vi "SpectrometerSpinCoater_v11.vi"() -> ()   [LabVIEW 2020]
uses:
  <instrlib>/Classes/CCD/Abstract_CCD/Abstract_CCD.lvclass
  <instrlib>/Classes/SpinCoater/SpinCoater.lvclass
  TypDef/DeviceQueue_TypeDef.ctl
  TypDef/DeviceQueue_Action.ctl
  TypDef/TabControl.ctl
  TypDef/DataQueue_TypeDef.ctl
  TypDef/DataQueue_Action.ctl
  <vilib>/Utility/error.llb/DialogType.ctl
  <instrlib>/Classes/CCD/Avantes/Avantes.lvclass
  C:/Program Files/National Instruments/LabVIEW 2020/instr.lib/Classes/CCD/Abstract_CCD/Abstract_CCD.lvclass
  <vilib>/Analysis/baseanly.llb/A x Vector.vi
  <vilib>/Analysis/NI_AALBase.lvlib
panel:
  out "UpperWLLimit":i32=713
  out "LowerWLLimit":i32=149
  out "Nr After Spin":u16
  out "Action":string="TimeOut"
  out "Time.spin":refnum<file>
  out "Meas.spin":refnum<file>
  out "Arduino":bool
  out "NKT":bool
  out "Spectromter":bool
  in  "Abort Button":bool
  in  "Stop Button":bool=TRUE
  in  "Tab Control":T1(tab)
  in  "Trim\nSpec":bool=TRUE
  in  "Wl \nUp":dbl[unit]=7.102291259765626e-07
  in  "Wl \nLow":dbl[unit]=3.7998095703125003e-07
  in  "Frames for Ref/Dark":dbl=10000.0
  in  "Shutter Toggle":bool
  in  "Spin at end":bool
  in  "Duration after":dbl[unit]
  in  "periodic time":dbl[unit]=2.0
  in  "Program Spin Coater":T2(array[cluster])=[{"Speed (rpm)"=1500.0, "Time (s)"=5.0, "Acc (rpm/s)"=0.0}]
  in  "Spectra Count":u16
  in  "Measure_MeasureSpectrum":bool
  out "Overall Time":dbl=13.0
  in  "Seconds after Spin":dbl[unit]=3.0
  in  "Seconds to Spin":dbl[unit]=5.0
  in  "Calculate Frames":bool=TRUE
  in  "Frames":i32=34211
  in  "StartMeasurement_Button":bool
  in  "Measure_Preview":bool
  out "Measure_Graph":T3(graph) caption="XY Graph"
  in  "Measure_FramesSpectrometer":dbl=200.0 caption="Frames for Spectrometer"
  in  "StartSpin_Button":bool
  in  "Record RefSpec":bool
  in  "Measure:\nRecord_Darkspec":bool
  in  "Measure_Comments":string="Just for testing" caption="Comments"
  in  "Measure_FileName":string="TestCutting_WithLight" caption="File Name"
  in  "Measure_SavePath":path=path "C:/Users/Cerberus/Desktop/Test/V11Test" caption="Save Path"
  out "Measure_FrameRate":dbl[unit]=2631.5791015625 caption="Frame Rate"
  in  "Measure_IntegrationTime":dbl[unit]=3e-05 caption="Integration Time"
  out "SS_StepsLeft":dbl
  out "SS_TimePrediction":dbl[unit]=-6.0
  out "Horizontal Progress Bar":u8(slide) scale=0.0..100.0
  in  "SpectralStability:\nRecord_Darkspec":bool
  in  "SpectralStability_Record":bool
  in  "SpectralStability_\nMeasurementNumber":u32 caption="Measurement Number"
  in  "SpectralStability_Duration":dbl[unit] caption="Duration"
  in  "Duration/Times":bool
  in  "SpectralStability_\nPeriodicTime":dbl[unit] caption="Periodic Time"
  in  "SpectralStability_MeasureSpectrum":bool
  in  "SpectralStability_Preview":bool
  out "SpectralStability_Graph":T3(graph) caption="XY Graph"
  in  "SpectralStability_FramesSpectrometer":dbl=200.0 caption="Frames for Spectrometer"
  in  "SpectralStability_Comments":string="Just for testing" caption="Comments"
  in  "SpectralStability_FileName":string="TestingAfter" caption="File Name"
  in  "SpectralStability_SavePath":path=path "C:/Users/Timo/Desktop/Test/180824" caption="Save Path"
  out "SpectralStability_FrameRate":dbl[unit]=2631.5791015625 caption="Frame Rate"
  in  "SpectralStability_IntegrationTime":dbl[unit]=3e-05 caption="Integration Time"
  in  "Shutter Close":bool
  in  "Shutter Open":bool
  in  "SHUTTER DEBUG":bool
  in  "Shutter Position":u16=1000
  in  "Dividider Get Spectra":u32=1 min=1
  in  "Automatically \nadjust count":bool=TRUE
  in  "Reset Count\nafter Spin Coating":bool=TRUE
  in  "ESC_Speed":dbl
  in  "ESC_Milliseconds":dbl
  in  "ESC DEBUG":bool
  in  "Port Arduino":refnum<visa-resource-name>="COM7"
  out "Error Arduino":bool caption="Error"
  in  "Init_Arduino":bool caption="Init"
  out "Caption_Settings_Arduino":string="Arduino"
  out "Caption_Settings_NKT":string="NKT Laser"
  out "Error_Spectromter":bool caption="Error"
  in  "Init_Spectrometer":bool caption="Init"
  out "Caption_Settings_Spectrometer":string="Spectromter"
  # "Speed (rpm)   Time (s)        Acceleration \n                                               (rpm/s)"
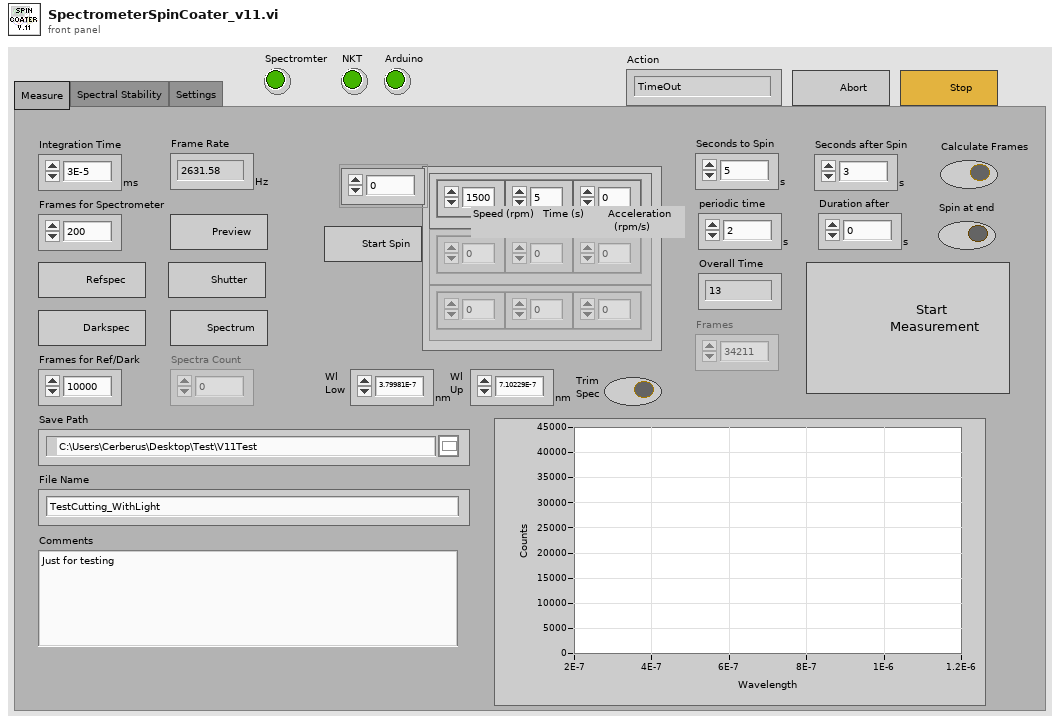
[diagram p1: front panel]
types:
  T1 = enum32{"Measure", "Spectral Stability", "Settings"}
  T2 = cluster{"Speed (rpm)":dbl, "Time (s)":dbl, "Acc (rpm/s)":dbl}[]
  T3 = cluster{"Wavlength":dbl[unit][], "Image":dbl[]}[]
  T4 = cluster{"Dark":cluster{"Image":dbl[][][], "Frame Size":cluster{"F":i32, "Y":i32, "X":i32}}[], "Ref":cluster{"Image":dbl[][][], "Frame Size":cluster{"F":i32, "Y":i32, "X":i32}}[], "Wavlength":dbl[unit][], "Wavlength Trim":dbl[unit][], "spec":dbl[][]}
  T5 = cluster{"Abstract_CCD.lvclass":refnum<class "Abstract_CCD.lvclass">, "SpinCoater.lvclass":refnum<class "SpinCoater.lvclass">}
  T6 = typedef "DataQueue_TypeDef.ctl" = cluster{"QueueAction":T7, "Data":cluster{"Image":dbl[][][], "Frame Size":cluster{"F":i32, "Y":i32, "X":i32}}[], "Data_Raw":cluster{"Image":dbl[][][], "Frame Size":cluster{"F":i32, "Y":i32, "X":i32}}[], "Data_Dark":cluster{"Image":dbl[][][], "Frame Size":cluster{"F":i32, "Y":i32, "X":i32}}[], "Data_Ref":cluster{"Image":dbl[][][], "Frame Size":cluster{"F":i32, "Y":i32, "X":i32}}[], "Device Information":string[], "Numeric Control":dbl, "Boolean":bool, "Wavelength":dbl[unit][], "Time":dbl[], "Time Stamp":timestamp, "Numeric Control 2":dbl, "TabControl":T8}
  T7 = typedef "DataQueue_Action.ctl" = enum16{"TimeOut", "Close_Program", "Abort", "Stop_Measurement", "Measure_InSituSpinCoating", "Measure_Spectrum", "Measure_SpectrumAdvanced", "Measure_SpectralStability", "Save_InSitu", "Save_SpectralStability", "Set_Ref", "Set_Dark", "Set_Wavelength", "Spectrometer_Measure", "Spectrometer_Preview", "Transfer_Settings", "Change_TrimSettings"}
  T8 = typedef "TabControl.ctl" = enum16{"Measure", "Spectral Stability", "Settings"}
  T9 = typedef "DeviceQueue_TypeDef.ctl" = cluster{"QueueAction":T10, "Numeric 1":dbl, "Numeric 2":dbl, "Boolean 1":bool, "Boolean 2":bool, "Spin Program":dbl[][], "Spin Prg v07":cluster{"Speed (rpm)":dbl, "Time (s)":dbl, "Acc (rpm/s)":dbl}[], "Time Stamp":timestamp, "TabControl":T8}
  T10 = typedef "DeviceQueue_Action.ctl" = enum16{"TimeOut", "Wait", "Close_Program", "Abort", "Spectrometer_Init", "Spectrometer_Close", "Spectrometer_DeviceInformation", "Spectrometer_Measure", "Spectrometer_MeasureAdvanced", "Spectrometer_Preview", "Spectrometer_Abort", "Spectrometer_StartMeasurement", "Spectrometer_GetData", "Spectrometer_StopMeasurement", "Spectrometer_SetIntegrationTime", "Spectrometer_SetFrames", "Spectrometer_SetDarkspec", "Spectrometer_SetReference", "Spectrometer_SetTriggerMode", "Laser_Init", "Laser_Close", "Arduino_Init", "Arduino_Close", "Arduino_LoadProgram", "Arduino_StartProgram", "Arduino_SetSpeed", "Arduino_SetMillis", "Arduino_StopSpin", "Arduino_Shutter_SetPosition", "Arduino_Shutter_Close", "Arduino_Shutter_Open", "Measure_InSitu", "Measure_Spectrum", "Measure_InSituAdvanced", "Measure_SpectralStability", "Measure_Stop"}
  T11 = cluster{"Image":dbl[][][], "Frame Size":cluster{"F":i32, "Y":i32, "X":i32}}[]
  T12 = typedef "DialogType.ctl" = u16
  T13 = enum16{"open", "replace", "create", "open or create", "replace or create", "replace or create with confirmation"}
  T14 = cluster{"Image":dbl[][][], "Frame Size":cluster{"F":i32, "Y":i32, "X":i32}}
  T15 = cluster{"Wavlength":dbl[unit][], "A x Vector":dbl[]}
  T16 = cluster{"Wavlength":dbl[unit][], "A x Vector":dbl[]}[]
  T17 = cluster{u16[][][], u16[][][], dbl[], "Numeric Control":dbl, "Numeric Control 2":dbl}
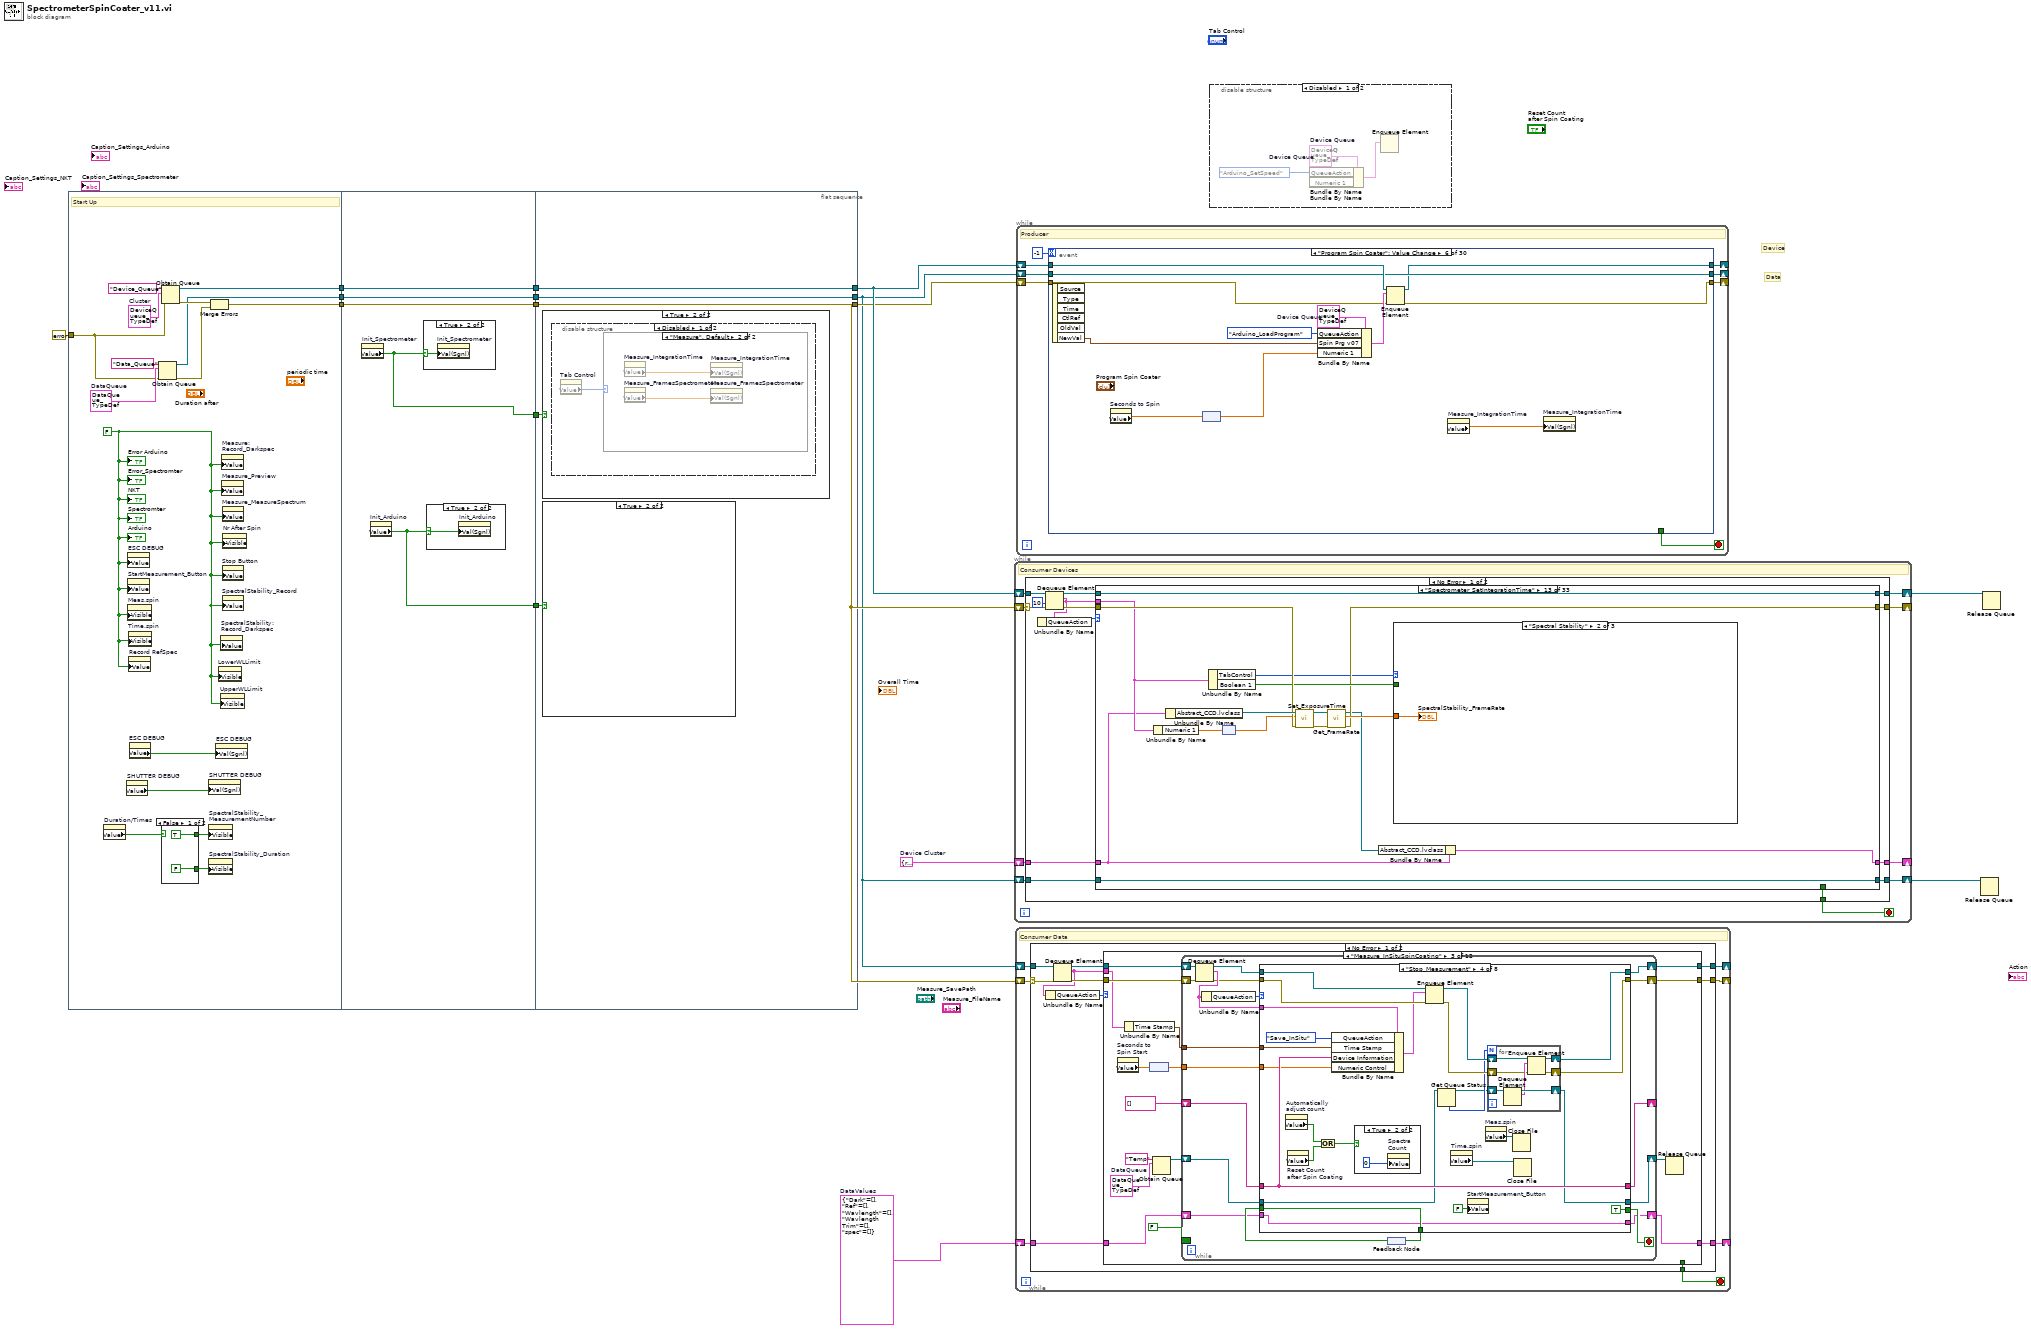
[diagram p0: block diagram]
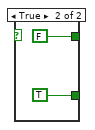
[diagram p3: hidden frame]
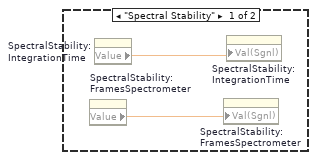
[diagram p8: hidden frame]
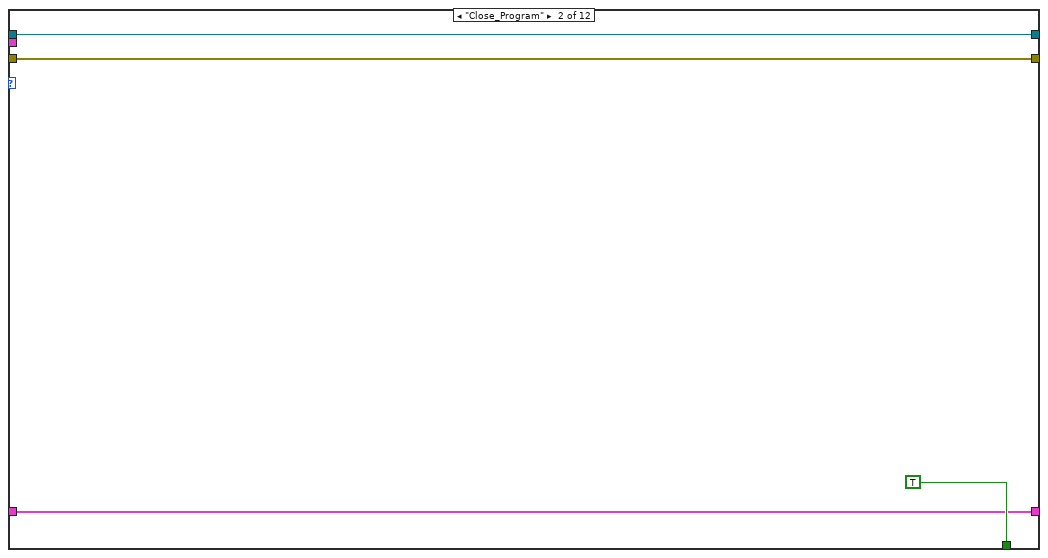
[diagram p11: hidden frame]
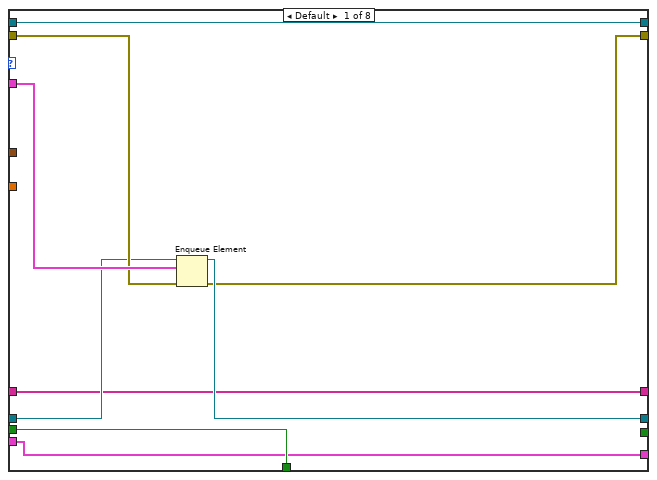
[diagram p12: hidden frame]
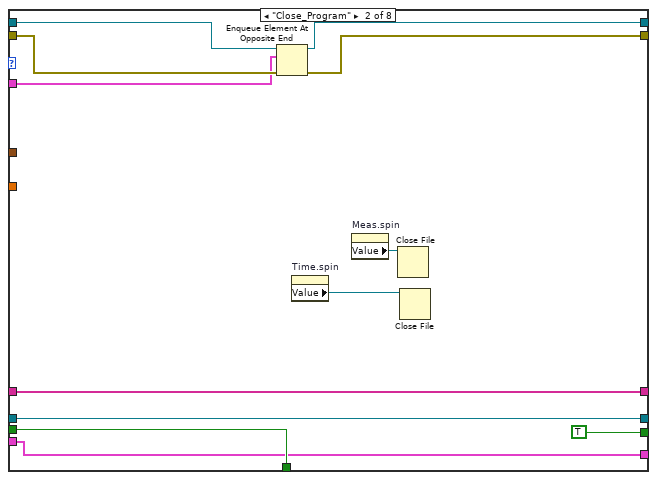
[diagram p13: hidden frame]
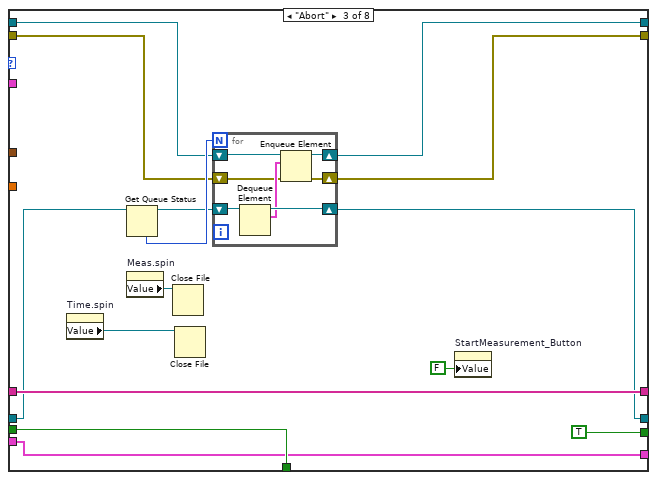
[diagram p14: hidden frame]
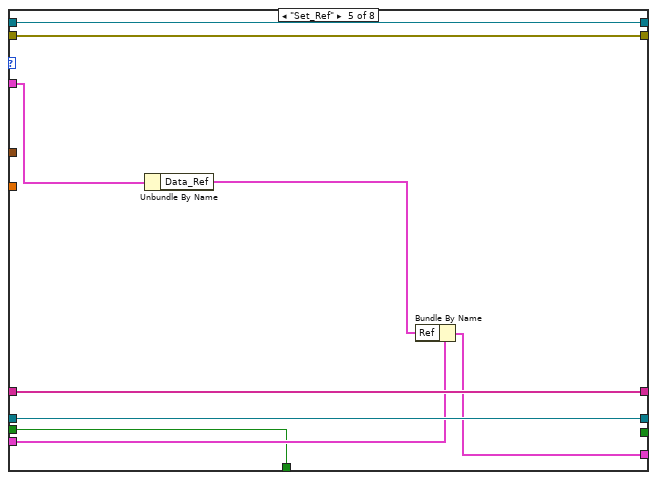
[diagram p16: hidden frame]
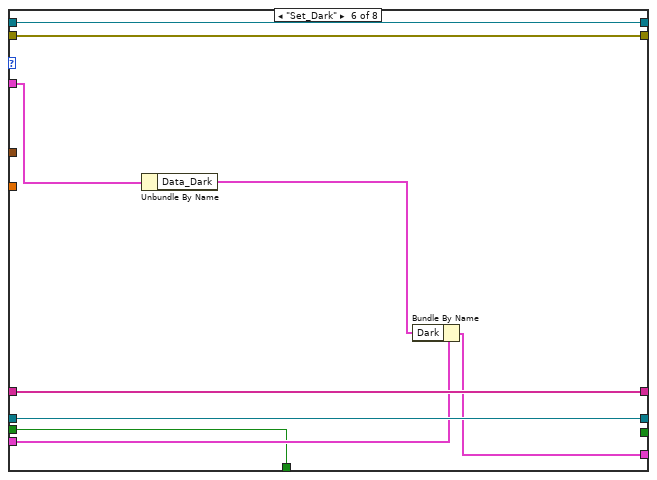
[diagram p17: hidden frame]
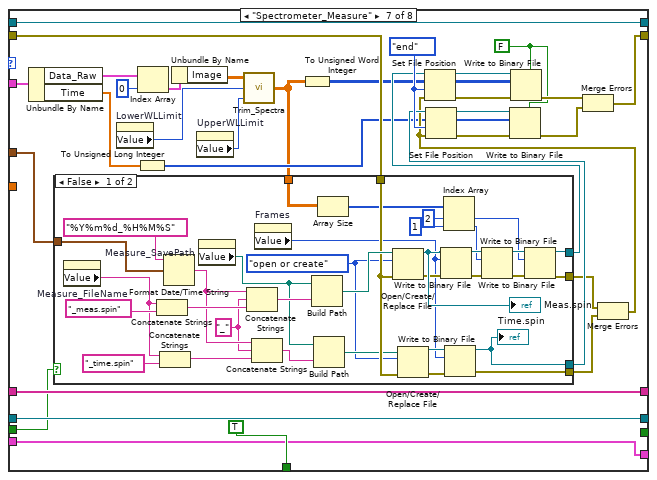
[diagram p18: hidden frame]
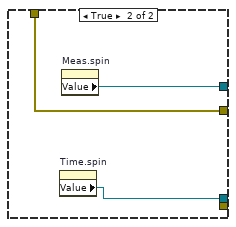
[diagram p19: hidden frame]
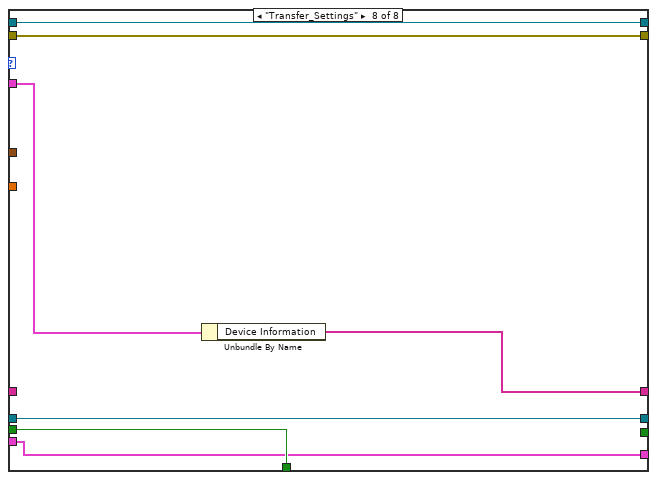
[diagram p20: hidden frame]
diagram:
  w6 = T4 {"Dark"=[], "Ref"=[], "Wavlength"=[], "Wavlength Trim"=[], "spec"=[]}  # DataValues
  w11 = T5 {"Abstract_CCD.lvclass"=refnum, "SpinCoater.lvclass"=refnum}  # Device Cluster
  # "Data"
  # "Device"
  n1 = flat-sequence {
    tunnel: errorcluster {"status"=FALSE, "code"=0, "source"=""} ("error constant") -> [w27]
    tunnel: [w30] -> w15
    tunnel: [w24] -> w14
    tunnel: [w23] -> w13
    tunnel: w15 -> [w41]
    tunnel: w14 -> [w40]
    tunnel: w13 -> [w39]
    tunnel: [w41] -> w5
    tunnel: [w40] -> w4
    tunnel: [w39] -> w3
    tunnel: [w38] -> w2
    tunnel: [w37] -> w1
    tunnel: [w46] -> w8
    tunnel: [w47] -> w7
    tunnel: [w48] -> w12
    tunnel: w5 -> [w48]
    tunnel: w4 -> [w47]
    tunnel: w3 -> [w46]
    tunnel: w2 -> [w45]
    tunnel: w1 -> [w44]
    frame #0 {
      w28 = T6 {"QueueAction"=enum."TimeOut", "Data"=[], "Data_Raw"=[], "Data_Dark"=[], "Data_Ref"=[], "Device Information"=[], "Numeric Control"=0.0, "Boolean"=FALSE, "Wavelength"=[], "Time"=[], "Time Stamp"=timestamp(0 s since 1904-01-01), "Numeric Control 2"=0.0, "TabControl"=enum."Measure"}  # DataQueue
      w31 = T9 {"QueueAction"=enum."TimeOut", "Numeric 1"=0.0, "Numeric 2"=0.0, "Boolean 1"=FALSE, "Boolean 2"=FALSE, "Spin Program"=[], "Spin Prg v07"=[], "Time Stamp"=timestamp(0 s since 1904-01-01), "TabControl"=enum."Measure"}  # Cluster
      w17 = FALSE ("Error Arduino")
      # "Start Up"
      n2 = property on="Duration/Times" class="Bool (strict)"() -> ("Value"=w19:bool)  [unwired: 2 in, 2 out]
      n3 = property on="SHUTTER DEBUG" class="Bool (strict)"() -> ("Value"=w18:bool)  [unwired: 2 in, 2 out]
      n4 = property on="ESC DEBUG" class="Bool (strict)"("Value"=w17) -> ()  [unwired: 2 in, 2 out]
      n5 = property on="StartMeasurement_Button" class="Bool (strict)"("Value"=w17) -> ()  [unwired: 2 in, 2 out]
      n6 = property on="Meas.spin" class="Ref (strict)"("Visible"=w17) -> ()  [unwired: 2 in, 2 out]
      n7 = property on="Time.spin" class="Ref (strict)"("Visible"=w17) -> ()  [unwired: 2 in, 2 out]
      n8 = property on="Record RefSpec" class="Bool (strict)"("Value"=w17) -> ()  [unwired: 2 in, 2 out]
      n9 = property on="ESC DEBUG" class="Bool (strict)"() -> ("Value"=w22:bool)  [unwired: 2 in, 2 out]
      n10 = Obtain Queue(name (unnamed)="Data_Queue", element data type=w28, error in (no error)=w27) -> (queue out=w24:refnum<queue>, error out=w25:errorcluster)  [unwired: 2 in, 1 out]
      n11 = case shown="False" w19 {
        tunnel: [FALSE TRUE] -> w21
        tunnel: [TRUE FALSE] -> w20
        frame False {
        }
        frame True {
        }
      }
      n12 = Obtain Queue(name (unnamed)="Device_Queue", element data type=w31, error in (no error)=w27) -> (queue out=w30:refnum<queue>, error out=w26:errorcluster)  [unwired: 2 in, 1 out]
      n13 = property on="SHUTTER DEBUG" class="Bool (strict)"("Val(Sgnl)"=w18) -> ()  [unwired: 2 in, 2 out]
      n14 = property on="SpectralStability_\nMeasurementNumber" class="DigNum (strict)"("Visible"=w20) -> ()  [unwired: 2 in, 2 out]
      n15 = property on="SpectralStability_Duration" class="DigNum (strict)"("Visible"=w21) -> ()  [unwired: 2 in, 2 out]
      n16 = Merge Errors(w26, w25) -> (w23:errorcluster)
      n17 = property on="ESC DEBUG" class="Bool (strict)"("Val(Sgnl)"=w22) -> ()  [unwired: 2 in, 2 out]
      n18 = property on="LowerWLLimit" class="DigNum (strict)"("Visible"=w17) -> ()  [unwired: 2 in, 2 out]
      n19 = property on="UpperWLLimit" class="DigNum (strict)"("Visible"=w17) -> ()  [unwired: 2 in, 2 out]
      n20 = property on="SpectralStability:\nRecord_Darkspec" class="Bool (strict)"("Value"=w17) -> ()  [unwired: 2 in, 2 out]
      n21 = property on="Measure:\nRecord_Darkspec" class="Bool (strict)"("Value"=w17) -> ()  [unwired: 2 in, 2 out]
      n22 = property on="Measure_Preview" class="Bool (strict)"("Value"=w17) -> ()  [unwired: 2 in, 2 out]
      n23 = property on="Measure_MeasureSpectrum" class="Bool (strict)"("Value"=w17) -> ()  [unwired: 2 in, 2 out]
      n24 = property on="Stop Button" class="Bool (strict)"("Value"=w17) -> ()  [unwired: 2 in, 2 out]
      n25 = property on="SpectralStability_Record" class="Bool (strict)"("Value"=w17) -> ()  [unwired: 2 in, 2 out]
      n26 = property on="Nr After Spin" class="DigNum (strict)"("Visible"=w17) -> ()  [unwired: 2 in, 2 out]
      "Error_Spectromter" <- w17
      "Error Arduino" <- w17
      "Spectromter" <- w17
      "NKT" <- w17
      "Arduino" <- w17
    }
    frame #1 {
      n27 = property on="Init_Spectrometer" class="Bool (strict)"() -> ("Value"=w38:bool)  [unwired: 2 in, 2 out]
      n28 = property on="Init_Arduino" class="Bool (strict)"() -> ("Value"=w37:bool)  [unwired: 2 in, 2 out]
      n29 = case shown="True" w38 {
        selector: w38 -> [_ w43]
        frame False {
        }
        frame True {
          n30 = property on="Init_Spectrometer" class="Bool (strict)"("Val(Sgnl)"=w43) -> ()  [unwired: 2 in, 2 out]
        }
      }
      n31 = case shown="True" w37 {
        selector: w37 -> [_ w42]
        frame False {
        }
        frame True {
          n32 = property on="Init_Arduino" class="Bool (strict)"("Val(Sgnl)"=w42) -> ()  [unwired: 2 in, 2 out]
        }
      }
    }
    frame #2 {
      n33 = case shown="True" w45 {
        frame False {
        }
        frame True {
          n34 = disable-structure shown="Disabled" {
            frame Disabled {
              n35 = property on="Tab Control" class="TabCtl (strict)"() -> ("Value"=w49:T1)  [unwired: 2 in, 2 out]
              n36 = case shown="\"Measure\", Default" w49 {
                frame "Spectral Stability" {
                  n37 = property on="SpectralStability:\nFramesSpectrometer" class="DigNum (strict)"() -> ("Value"=w50:dbl)  [unwired: 2 in, 2 out]
                  n38 = property on="SpectralStability:\nIntegrationTime" class="DigNum (strict)"() -> ("Value"=w51:dbl[unit])  [unwired: 2 in, 2 out]
                  n39 = property on="SpectralStability:\nFramesSpectrometer" class="DigNum (strict)"("Val(Sgnl)"=w50) -> ()  [unwired: 2 in, 2 out]
                  n40 = property on="SpectralStability:\nIntegrationTime" class="DigNum (strict)"("Val(Sgnl)"=w51) -> ()  [unwired: 2 in, 2 out]
                }
                frame "Measure", Default {
                  n41 = property on="Measure_IntegrationTime" class="DigNum (strict)"() -> ("Value"=w52:dbl[unit])  [unwired: 2 in, 2 out]
                  n42 = property on="Measure_FramesSpectrometer" class="DigNum (strict)"() -> ("Value"=w53:dbl)  [unwired: 2 in, 2 out]
                  n43 = property on="Measure_IntegrationTime" class="DigNum (strict)"("Val(Sgnl)"=w52) -> ()  [unwired: 2 in, 2 out]
                  n44 = property on="Measure_FramesSpectrometer" class="DigNum (strict)"("Val(Sgnl)"=w53) -> ()  [unwired: 2 in, 2 out]
                }
              }
            }
            frame Enabled {
            }
          }
        }
      }
      n45 = case shown="True" w44 {
        frame False {
        }
        frame True {
        }
      }
    }
  }
  n46 = while {
    shift-right: [w58] -> _
    shift-left: w8 -> [w62]
    shift-right: [w59] -> w10
    shift-left: w12 -> [w61]
    shift-right: [w56] -> w9
    shift-left: w7 -> [w57]
    shift-right: [w54] -> _
    shift-left: w11 -> [w55]
    stop <- w60 stop-if-true
    # "Consumer Devices"
    n47 = case shown="No Error" w62 {
      selector: w62 -> [w75 w792]
      tunnel: w61 -> [w76 w793]
      tunnel: [w72 _] -> w60
      tunnel: [w71 w793] -> w59
      tunnel: [w69 w789] -> w58
      tunnel: w57 -> [w67 w787]
      tunnel: [w68 w787] -> w56
      tunnel: w55 -> [w66 w788]
      tunnel: [w65 w788] -> w54
      frame No Error {
        n48 = Dequeue Element(queue=w76, timeout in ms (-1)=10, error in (no error)=w75) -> (queue out=w74:refnum<queue>, element=w64:T9, error out=w70:errorcluster)  [unwired: 1 out]
        n49 = Unbundle By Name(w64) -> ("QueueAction"=w73:T10)
        n50 = case shown="\"Spectrometer_SetIntegrationTime\"" w73 {
          tunnel: w74 -> [w81 w102 w143 w161 w172 w227 w246 w271 w282 w305 w312 w331 w333 w364 w383 w398 w408 w420 w432 w453 w475 w480 w487 w499 w505 w517 w524 w531 w540 w586 w680 w748 w758]
          tunnel: [_ _ w145 _ _ _ _ _ _ _ _ _ _ _ _ _ _ _ _ _ _ _ _ _ _ _ _ _ _ _ _ _ _] -> w72
          tunnel: [w81 w102 w128 w147 w168 w227 w246 w271 w283 w305 w312 w331 w333 w364 w383 w398 w408 w420 w431 w453 w475 w480 w487 w499 w505 w517 w524 w531 w540 w548 w596 w739 w761] -> w71
          tunnel: w70 -> [w80 w101 w127 w160 w183 w228 w245 w270 w278 w308 w316 w328 w343 w362 w373 w389 w405 w416 w427 w456 w469 w477 w485 w494 w502 w508 w520 w527 w533 w542 w641 w747 w757]
          tunnel: [w80 w101 w126 w148 w171 w222 w244 w269 w276 w306 w313 w318 w337 w361 w368 w385 w403 w410 w430 w455 w466 w476 w483 w493 w501 w507 w519 w526 w532 w549 w595 w738 w762] -> w69
          tunnel: [w78 w99 w125 w165 w169 w224 w237 w251 w287 w304 w311 w322 w345 w365 w377 w392 w399 w412 w434 w454 w474 w482 w491 w497 w506 w516 w523 w530 w535 w557 w653 w746 w778] -> w68
          tunnel: w67 -> [w78 w99 w125 w165 w170 w224 w236 w260 w288 w304 w311 w323 w345 w365 w380 w395 w399 w414 w434 w454 w474 w482 w491 w497 w506 w516 w523 w530 w536 w557 w653 w746 w778]
          tunnel: w66 -> [w79 w100 w124 w164 w180 w226 w243 w268 w281 w303 w315 w324 w336 w358 w376 w391 w402 w409 w429 w449 w468 w481 w490 w496 w504 w515 w522 w529 w534 w589 w683 w745 w777]
          tunnel: [w79 w100 w124 w164 w174 w225 w243 w268 w280 w301 w310 w324 w334 w359 w375 w390 w400 w409 w433 w447 w465 w481 w490 w496 w504 w515 w522 w529 w534 w589 w683 w745 w777] -> w65
          tunnel: w64 -> [_ w95 _ _ w167 _ w235 w262 w274 _ _ w330 w340 w366 _ _ w406 _ _ _ w473 _ w489 w498 _ w513 _ _ _ _ w623 w736 w752]
          frame "TimeOut", Default {
            n51 = property on="Action" class="Str"("Value"="TimeOut" ("Action")) -> ()  [unwired: 2 in, 2 out]
          }
          frame "Wait" {
            n52 = flat-sequence {
              tunnel: [w113] -> w96
              tunnel: w95 -> [w113]
              tunnel: [w112] -> w93
              frame #0 {
                n53 = Tick Count (ms)() -> (millisecond timer value=w112:u32)
              }
            }
            n54 = Unbundle By Name(w96) -> ("Numeric 1"=w87:dbl)
            n55 = property on="SS:PeriodicTime" class="DigNum (strict)"() -> ("Value"=w89:dbl[unit])  [unwired: 2 in, 2 out]
            n56 = Multiply(x=w87, y=1000.0) -> (x*y=w91:dbl)
            n57 = node(w87) -> (w88:dbl[unit])
            n58 = property on="SS_StepsLeft" class="DigNum (strict)"() -> ("Value"=w86:dbl)  [unwired: 2 in, 2 out]
            n59 = Round Toward -Infinity(1:w87) -> (0:w90:dbl)
            n60 = Subtract(x=w89, y=w88) -> (x-y=w83:dbl[unit])
            n61 = Decrement(x=w86) -> (x-1=w85:dbl)
            n62 = Multiply(x=w85, y=w89) -> (x*y=w84:dbl[unit])
            n63 = Add(x=w84, y=w83) -> (x+y=w82:dbl[unit])
            n64 = for {
              N: w90 -> [_]
              tunnel: 1000.0 ("y") -> [w114]
              tunnel: [w122] -> w94
              tunnel: w82 -> [w119]
              i -> [w117]
              stop <- w122 stop-if-true
              n65 = Increment(x=w117) -> (x+1=w115:i32)
              n66 = Multiply(x=w114, y=w115) -> (x*y=w116:dbl)
              n67 = node(w116) -> (w118:dbl[unit])
              n68 = property on="Stop Button" class="Bool (strict)"() -> ("Value"=w122:bool)  [unwired: 2 in, 2 out]
              n69 = Wait (ms)(milliseconds to wait=w114) -> (millisecond timer value=w120:u32)
              n70 = Subtract(x=w119, y=w118) -> (x-y=w121:dbl[unit])
              n71 = flat-sequence {
                tunnel: w121 -> [w123]
                tunnel: w120 -> [_]
                frame #0 {
                  n72 = property on="SS_TimePrediction" class="DigNum (strict)"("Value"=w123) -> ()  [unwired: 2 in, 2 out]
                }
              }
            }
            n73 = property on="Action" class="Str"("Value"="Wait" ("Action")) -> ()  [unwired: 2 in, 2 out]
            n74 = case shown="False" w94 {
              tunnel: w93 -> [w108 _]
              tunnel: w91 -> [w103 _]
              frame False {
                n75 = flat-sequence {
                  tunnel: [w111] -> w109
                  frame #0 {
                    n76 = Tick Count (ms)() -> (millisecond timer value=w111:u32)
                  }
                }
                n77 = Subtract(x=w109, y=w108) -> (x-y=w107:u32)
                n78 = To Double Precision Float(number=w107) -> (double precision float=w104:dbl)
                n79 = Subtract(x=w103, y=w104) -> (x-y=w105:dbl)
                n80 = Greater Than 0?(x=w105) -> (x > 0?=w106:bool)
                n81 = case shown="True" w106 {
                  tunnel: w105 -> [_ w110]
                  frame False {
                  }
                  frame True {
                    n82 = Wait (ms)(milliseconds to wait=w110) -> ()  [unwired: 1 out]
                  }
                }
              }
              frame True {
                # "If Aborted, do nothing"
              }
            }
          }
          frame "Close_Program" {
            w144 = T9 {"QueueAction"=enum."TimeOut", "Numeric 1"=0.0, "Numeric 2"=0.0, "Boolean 1"=FALSE, "Boolean 2"=FALSE, "Spin Program"=[], "Spin Prg v07"=[], "Time Stamp"=timestamp(0 s since 1904-01-01), "TabControl"=enum."Measure"}  # Device Queue
            n83 = Bundle By Name(cluster=w144, "QueueAction"=DeviceQueue_Action."Spectrometer_Close") -> (w139:T9)
            n84 = Bundle By Name(cluster=w139, "QueueAction"=DeviceQueue_Action."Laser_Close") -> (w137:T9)
            n85 = Bundle By Name(cluster=w137, "QueueAction"=DeviceQueue_Action."Arduino_Close") -> (w131:T9)
            n86 = Enqueue Element(queue=w143, element=w139, error in (no error)=w127) -> (queue out=w141:refnum<queue>, error out=w136:errorcluster)  [unwired: 1 in, 1 out]
            n87 = Bundle By Name(cluster=w131, "QueueAction"=DeviceQueue_Action."Close_Program") -> (w129:T9)
            n88 = Enqueue Element(queue=w141, element=w137, error in (no error)=w136) -> (queue out=w135:refnum<queue>, error out=w134:errorcluster)  [unwired: 1 in, 1 out]
            n89 = Enqueue Element(queue=w135, element=w131, error in (no error)=w134) -> (queue out=w133:refnum<queue>, error out=w132:errorcluster)  [unwired: 1 in, 1 out]
            n90 = Enqueue Element(queue=w133, element=w129, error in (no error)=w132) -> (queue out=w128:refnum<queue>, error out=w126:errorcluster)  [unwired: 1 in, 1 out]
            n91 = First Call?() -> (First Call?: T/F=w146:bool)
            n92 = Not(x=w146) -> (.not. x?=w145:bool)
          }
          frame "Abort" {
            w163 = T9 {"QueueAction"=enum."TimeOut", "Numeric 1"=0.0, "Numeric 2"=0.0, "Boolean 1"=FALSE, "Boolean 2"=FALSE, "Spin Program"=[], "Spin Prg v07"=[], "Time Stamp"=timestamp(0 s since 1904-01-01), "TabControl"=enum."Measure"}  # Device Queue
            n93 = Flush Queue(queue=w161, error in (no error)=w160) -> (queue out=w159:refnum<queue>, error out=w158:errorcluster)  [unwired: 1 out]
            n94 = Bundle By Name(cluster=w163, "QueueAction"=DeviceQueue_Action."Spectrometer_StopMeasurement") -> (w155:T9)
            n95 = Bundle By Name(cluster=w155, "QueueAction"=DeviceQueue_Action."Arduino_StopSpin") -> (w151:T9)
            n96 = Enqueue Element(queue=w159, element=w155, error in (no error)=w158) -> (queue out=w157:refnum<queue>, error out=w156:errorcluster)  [unwired: 1 in, 1 out]
            n97 = Bundle By Name(cluster=w151, "QueueAction"=DeviceQueue_Action."Measure_Stop") -> (w150:T9)
            n98 = Enqueue Element(queue=w157, element=w151, error in (no error)=w156) -> (queue out=w153:refnum<queue>, error out=w152:errorcluster)  [unwired: 1 in, 1 out]
            n99 = Enqueue Element(queue=w153, element=w150, error in (no error)=w152) -> (queue out=w147:refnum<queue>, error out=w148:errorcluster)  [unwired: 1 in, 1 out]
          }
          frame "Spectrometer_Init" {
            n100 = call-dynamic "Init.vi"("error in (no error)"=w183, "Variant"=0, "Avantes in"=refnum<class "Avantes.lvclass"> refnum ("Avantes.lvclass")) -> ("error out"=w182:errorcluster, "Avantes out"=w181:refnum<class "Avantes.lvclass">)  [unwired: 7 in]
            n101 = call-dynamic "IsInit.vi"("error in (no error)"=w182, "Avantes in"=w181) -> ("error out"=w178:errorcluster, "Is Init?"=w177:bool, "Avantes out"=w179:refnum<class "Avantes.lvclass">)  [unwired: 7 in]
            n102 = Unbundle By Name(w167) -> ("TabControl"=w166:T8)
            n103 = property on="Spectromter" class="Bool (strict)"("Value"=w177) -> ()  [unwired: 2 in, 2 out]
            n104 = property on="Init_Spectrometer" class="Bool (strict)"("Value"=w177) -> ()  [unwired: 2 in, 2 out]
            n105 = call-dynamic "Set_ExposurePerFrame.vi"("error in (no error)"=w178, "Exposure per Frame"=1, "Avantes in"=w179) -> ("error out"=w173:errorcluster, "Avantes out"=w176:refnum<class "Avantes.lvclass">)  [unwired: 7 in]
            n106 = case shown="True" w177 {
              tunnel: w176 -> [_ w206]
              tunnel: w173 -> [w189 w204]
              tunnel: [refnum<class "Abstract_CCD.lvclass"> refnum ("Abstract_CCD.lvclass") w205] -> w175
              tunnel: w172 -> [w187 w216]
              tunnel: [w189 w209] -> w171
              tunnel: w170 -> [w188 w201]
              tunnel: [w188 w199] -> w169
              tunnel: [w187 w197] -> w168
              tunnel: w167 -> [_ w194]
              tunnel: w166 -> [_ w193]
              frame False {
              }
              frame True {
                w207 = T6 {"QueueAction"=enum."TimeOut", "Data"=[], "Data_Raw"=[], "Data_Dark"=[], "Data_Ref"=[], "Device Information"=[], "Numeric Control"=0.0, "Boolean"=FALSE, "Wavelength"=[], "Time"=[], "Time Stamp"=timestamp(0 s since 1904-01-01), "Numeric Control 2"=0.0, "TabControl"=enum."Measure"}  # DataQueue
                n107 = case shown="\"Spectral Stability\"" w193 {
                  tunnel: [w218 w220] -> w192
                  tunnel: [w217 w219] -> w191
                  frame "Measure", Default {
                    n108 = property on="Measure_IntegrationTime" class="DigNum (strict)"() -> ("Value"=w218:dbl[unit])  [unwired: 2 in, 2 out]
                    n109 = property on="Measure_FramesSpectrometer" class="DigNum (strict)"() -> ("Value"=w217:dbl)  [unwired: 2 in, 2 out]
                  }
                  frame "Spectral Stability" {
                    n110 = property on="SpectralStability_FramesSpectrometer" class="DigNum (strict)"() -> ("Value"=w219:dbl)  [unwired: 2 in, 2 out]
                    n111 = property on="SpectralStability_IntegrationTime" class="DigNum (strict)"() -> ("Value"=w220:dbl[unit])  [unwired: 2 in, 2 out]
                  }
                }
                n112 = call-dynamic "Get_WavelengthAxis.vi"("error in (no error)"=w204, "Avantes in"=w206) -> ("error out"=w203:errorcluster, "lambda"=w198:dbl[unit][], "Avantes out"=w205:refnum<class "Avantes.lvclass">)  [unwired: 7 in]
                n113 = Unbundle(w203) -> ("status"=w202:bool)  [unwired: 2 out]
                n114 = property on="Error_Spectromter" class="Bool (strict)"("Value"=w202) -> ()  [unwired: 2 in, 2 out]
                n115 = property on="Calculate Frames" class="Bool (strict)"() -> ("Value"=w195:bool)  [unwired: 2 in, 2 out]
                n116 = Bundle By Name(cluster=w207, "QueueAction"=DataQueue_Action."Set_Wavelength", "Wavelength"=w198) -> (w208:T6)
                n117 = node(w192) -> (w214:dbl)
                n118 = Bundle By Name(cluster=w194, "QueueAction"=DeviceQueue_Action."Spectrometer_SetIntegrationTime", "Numeric 1"=w214, "Boolean 1"=w195) -> (w212:T9)
                n119 = Enqueue Element(queue=w201, element=w208) -> (queue out=w199:refnum<queue>)  [unwired: 2 in, 2 out]
                n120 = Bundle By Name(cluster=w212, "QueueAction"=DeviceQueue_Action."Spectrometer_SetFrames", "Numeric 1"=w191) -> (w211:T9)
                n121 = Enqueue Element(queue=w216, element=w212, error in (no error)=w204) -> (queue out=w213:refnum<queue>, error out=w210:errorcluster)  [unwired: 1 in, 1 out]
                n122 = Enqueue Element(queue=w213, element=w211, error in (no error)=w210) -> (queue out=w197:refnum<queue>, error out=w209:errorcluster)  [unwired: 1 in, 1 out]
              }
            }
            n123 = Bundle By Name(cluster=w180, "Abstract_CCD.lvclass"=w175) -> (w174:T5)
          }
          frame "Spectrometer_Close" {
            n124 = property on="Spectromter" class="Bool (strict)"("Value"=FALSE ("Spectromter")) -> ()  [unwired: 2 in, 2 out]
            n125 = Unbundle By Name(w226) -> ("Abstract_CCD.lvclass"=w229:refnum<class "Abstract_CCD.lvclass">)
            n126 = flat-sequence {
              tunnel: [refnum<class "Abstract_CCD.lvclass"> refnum ("Abstract_CCD.lvclass")] -> w223
              tunnel: w222 -> [_]
              frame #0 {
              }
            }
            n127 = call-dynamic "Close.vi"("error in (no error)"=w228, "Abstract_CCD in"=w229) -> ("error out"=w222:errorcluster)  [unwired: 8 in, 1 out]
            n128 = Bundle By Name(cluster=w226, "Abstract_CCD.lvclass"=w223) -> (w225:T5)
          }
          frame "Spectrometer_Measure" {
            w248 = T6 {"QueueAction"=enum."TimeOut", "Data"=[], "Data_Raw"=[], "Data_Dark"=[], "Data_Ref"=[], "Device Information"=[], "Numeric Control"=0.0, "Boolean"=FALSE, "Wavelength"=[], "Time"=[], "Time Stamp"=timestamp(0 s since 1904-01-01), "Numeric Control 2"=0.0, "TabControl"=enum."Measure"}  # DataQueue
            n129 = Unbundle By Name(w243) -> ("Abstract_CCD.lvclass"=w247:refnum<class "Abstract_CCD.lvclass">)
            n130 = Unbundle By Name(w235) -> ("Time Stamp"=w232:timestamp, "TabControl"=w233:T8)
            n131 = Get Date/Time In Seconds() -> (seconds since 1Jan1904=w231:timestamp)
            n132 = Subtract(x=w231, y=w232) -> (x-y=w234:dbl)
            n133 = call-dynamic "Measure.vi"("error in (no error)"=w245, "Abstract_CCD in"=w247) -> ("error out"=w244:errorcluster, "Data Raw"=w240:T11, "Data"=w241:T11, "Darkspec"=w239:T11, "Time"=w238:dbl[])  [unwired: 3 in, 2 out]
            n134 = Bundle By Name(cluster=w248, "QueueAction"=DataQueue_Action."Spectrometer_Measure", "Data"=w241, "Data_Raw"=w240, "Data_Dark"=w239, "Time"=w238, "Time Stamp"=w232, "Numeric Control 2"=w234, "TabControl"=w233) -> (w249:T6)
            n135 = Enqueue Element(queue=w236, element=w249) -> (queue out=w237:refnum<queue>)  [unwired: 2 in, 2 out]
          }
          frame "Spectrometer_MeasureAdvanced" {
            w259 = T6 {"QueueAction"=enum."TimeOut", "Data"=[], "Data_Raw"=[], "Data_Dark"=[], "Data_Ref"=[], "Device Information"=[], "Numeric Control"=0.0, "Boolean"=FALSE, "Wavelength"=[], "Time"=[], "Time Stamp"=timestamp(0 s since 1904-01-01), "Numeric Control 2"=0.0, "TabControl"=enum."Measure"}  # DataQueue
            w273 = T6 {"QueueAction"=enum."TimeOut", "Data"=[], "Data_Raw"=[], "Data_Dark"=[], "Data_Ref"=[], "Device Information"=[], "Numeric Control"=0.0, "Boolean"=FALSE, "Wavelength"=[], "Time"=[], "Time Stamp"=timestamp(0 s since 1904-01-01), "Numeric Control 2"=0.0, "TabControl"=enum."Measure"}  # DataQueue
            n136 = Unbundle By Name(w268) -> ("Abstract_CCD.lvclass"=w272:refnum<class "Abstract_CCD.lvclass">)
            n137 = Unbundle By Name(w262) -> ("Time Stamp"=w261:timestamp)
            n138 = call-dynamic "Measure.vi"("error in (no error)"=w270, "Abstract_CCD in"=w272) -> ("error out"=w269:errorcluster, "Data Raw"=w265:T11, "Data"=w266:T11, "Darkspec"=w264:T11, "Time"=w263:dbl[])  [unwired: 3 in, 2 out]
            n139 = Bundle By Name(cluster=w259, "QueueAction"=DataQueue_Action."Measure_SpectrumAdvanced") -> (w257:T6)
            n140 = Bundle By Name(cluster=w273, "QueueAction"=DataQueue_Action."Spectrometer_Measure", "Data"=w266, "Data_Raw"=w265, "Data_Dark"=w264, "Time"=w263, "Time Stamp"=w261) -> (w254:T6)
            n141 = Enqueue Element(queue=w260, element=w257) -> (queue out=w256:refnum<queue>)  [unwired: 2 in, 2 out]
            n142 = Enqueue Element(queue=w256, element=w254) -> (queue out=w255:refnum<queue>)  [unwired: 2 in, 2 out]
            n143 = Bundle By Name(cluster=w254, "QueueAction"=DataQueue_Action."Stop_Measurement") -> (w252:T6)
            n144 = property on="Action" class="Str"("Value"="Measure Spectra A" ("Action")) -> ()  [unwired: 2 in, 2 out]
            n145 = Enqueue Element(queue=w255, element=w252) -> (queue out=w251:refnum<queue>)  [unwired: 2 in, 2 out]
          }
          frame "Spectrometer_Preview" {
            w289 = T6 {"QueueAction"=enum."TimeOut", "Data"=[], "Data_Raw"=[], "Data_Dark"=[], "Data_Ref"=[], "Device Information"=[], "Numeric Control"=0.0, "Boolean"=FALSE, "Wavelength"=[], "Time"=[], "Time Stamp"=timestamp(0 s since 1904-01-01), "Numeric Control 2"=0.0, "TabControl"=enum."Measure"}  # DataQueue
            n146 = Unbundle By Name(w281) -> ("Abstract_CCD.lvclass"=w279:refnum<class "Abstract_CCD.lvclass">)
            n147 = Unbundle By Name(w274) -> ("TabControl"=w275:T8)
            n148 = call-dynamic "Measure.vi"("error in (no error)"=w278, "Abstract_CCD in"=w279) -> ("error out"=w276:errorcluster, "Data Raw"=w286:T11, "Abstract_CCD out"=w277:refnum<class "Abstract_CCD.lvclass">)  [unwired: 3 in, 4 out]
            n149 = case shown="\"Measure\"" w275 {
              tunnel: [FALSE ("Value") w293 w294] -> w284
              tunnel: w276 -> [_ w292 _]
              frame Default {
              }
              frame "Measure" {
                n150 = property on="Measure_Preview" class="Bool (strict)"(error in=w292) -> ("Value"=w293:bool)  [unwired: 1 in, 2 out]
              }
              frame "Spectral Stability" {
                n151 = property on="SpectralStability_Preview" class="Bool (strict)"() -> ("Value"=w294:bool)  [unwired: 2 in, 2 out]
              }
            }
            n152 = case shown="True" w284 {
              tunnel: [w295 w298] -> w283
              tunnel: w282 -> [w295 w297]
              tunnel: w274 -> [_ w296]
              frame False {
              }
              frame True {
                n153 = Bundle By Name(cluster=w296, "QueueAction"=DeviceQueue_Action."Spectrometer_Preview") -> (w299:T9)
                n154 = Enqueue Element(queue=w297, element=w299) -> (queue out=w298:refnum<queue>)  [unwired: 2 in, 2 out]
              }
            }
            n155 = Bundle By Name(cluster=w289, "Data_Raw"=w286, "QueueAction"=DataQueue_Action."Spectrometer_Preview", "TabControl"=w275) -> (w290:T6)
            n156 = Enqueue Element(queue=w288, element=w290) -> (queue out=w287:refnum<queue>)  [unwired: 2 in, 2 out]
            n157 = Bundle By Name(cluster=w281, "Abstract_CCD.lvclass"=w277) -> (w280:T5)
          }
          frame "Spectrometer_StartMeasurement" {
            n158 = Unbundle By Name(w303) -> ("Abstract_CCD.lvclass"=w307:refnum<class "Abstract_CCD.lvclass">)
            n159 = call-dynamic "StartMeasure.vi"("error in (no error)"=w308, "Frames"=-1, "Abstract_CCD in"=w307) -> ("error out"=w306:errorcluster, "Abstract_CCD out"=w302:refnum<class "Abstract_CCD.lvclass">)  [unwired: 7 in]
            n160 = Bundle By Name(cluster=w303, "Abstract_CCD.lvclass"=w302) -> (w301:T5)
          }
          frame "Spectrometer_StopMeasurement" {
            n161 = Unbundle By Name(w315) -> ("Abstract_CCD.lvclass"=w317:refnum<class "Abstract_CCD.lvclass">)
            n162 = call-dynamic "StopMeasurement.vi"("error in (no error)"=w316, "Abstract_CCD in"=w317) -> ("error out"=w313:errorcluster, "Abstract_CCD out"=w314:refnum<class "Abstract_CCD.lvclass">)  [unwired: 8 in]
            n163 = Bundle By Name(cluster=w315, "Abstract_CCD.lvclass"=w314) -> (w310:T5)
          }
          frame "Spectrometer_GetData" {
            w327 = T6 {"QueueAction"=enum."TimeOut", "Data"=[], "Data_Raw"=[], "Data_Dark"=[], "Data_Ref"=[], "Device Information"=[], "Numeric Control"=0.0, "Boolean"=FALSE, "Wavelength"=[], "Time"=[], "Time Stamp"=timestamp(0 s since 1904-01-01), "Numeric Control 2"=0.0, "TabControl"=enum."Measure"}  # DataQueue
            n164 = Unbundle By Name(w324) -> ("Abstract_CCD.lvclass"=w329:refnum<class "Abstract_CCD.lvclass">)
            n165 = Unbundle By Name(w330) -> ("Numeric 1"=w321:dbl)
            n166 = call-dynamic "Measure_GetData.vi"("error in (no error)"=w328, "SpectraCount"=w321, "Abstract_CCD in"=w329) -> ("error out"=w318:errorcluster, "Data_Raw"=w320:T11, "Time"=w319:dbl[])  [unwired: 5 in, 1 out]
            n167 = Bundle By Name(cluster=w327, "QueueAction"=DataQueue_Action."Spectrometer_Measure", "Data_Raw"=w320, "Time"=w319) -> (w326:T6)
            n168 = Enqueue Element(queue=w323, element=w326) -> (queue out=w322:refnum<queue>)  [unwired: 2 in, 2 out]
          }
          frame "Spectrometer_SetIntegrationTime" {
            n169 = Unbundle By Name(w340) -> ("Numeric 1"=w342:dbl)
            n170 = Unbundle By Name(w336) -> ("Abstract_CCD.lvclass"=w344:refnum<class "Abstract_CCD.lvclass">)
            n171 = Unbundle By Name(w340) -> ("TabControl"=w332:T8, "Boolean 1"=w339:bool)
            n172 = node(w342) -> (w341:dbl[unit])
            n173 = call-dynamic "Set_ExposureTime.vi"("error in (no error)"=w343, "Exposure Time"=w341, "Abstract_CCD in"=w344) -> ("error out"=w347:errorcluster, "Abstract_CCD out"=w346:refnum<class "Abstract_CCD.lvclass">)  [unwired: 7 in]
            n174 = call-dynamic "Get_FrameRate.vi"("error in (no error)"=w347, "Abstract_CCD in"=w346) -> ("error out"=w337:errorcluster, "Frame Rate"=w338:dbl[unit], "Abstract_CCD out"=w335:refnum<class "Abstract_CCD.lvclass">)  [unwired: 7 in]
            n175 = Bundle By Name(cluster=w336, "Abstract_CCD.lvclass"=w335) -> (w334:T5)
            n176 = case shown="\"Spectral Stability\"" w332 {
              tunnel: w339 -> [_ _ w350]
              tunnel: w338 -> [_ w348 w349]
              frame Default {
              }
              frame "Spectral Stability" {
                "SpectralStability_FrameRate" <- w348
              }
              frame "Measure" {
                n177 = case shown="True" w350 {
                  tunnel: w349 -> [_ w354]
                  frame False {
                  }
                  frame True {
                    n178 = property on="Program Spin Coater" class="Arr (strict)"() -> ("Value"=w351:T2)  [unwired: 2 in, 2 out]
                    n179 = property on="Seconds to Spin" class="DigNum (strict)"() -> ("Value"=w356:dbl[unit])  [unwired: 2 in, 2 out]
                    n180 = property on="Seconds after Spin" class="DigNum (strict)"() -> ("Value"=w355:dbl[unit])  [unwired: 2 in, 2 out]
                    n181 = call "CalculateFrames_v03.vi"("Program Spin Coater"=w351, "Seconds End"=w355, "Seconds Start"=w356, "Frame Rate"=w354) -> ("Time"=w353:dbl, "Frames"=w352:i32)  [unwired: 6 in]
                    n182 = property on="Frames" class="DigNum (strict)"("Value"=w352) -> ()  [unwired: 2 in, 2 out]
                    n183 = property on="Overall Time" class="DigNum (strict)"("Value"=w353) -> ()  [unwired: 2 in, 2 out]
                  }
                }
                "Measure_FrameRate" <- w349
              }
            }
          }
          frame "Spectrometer_SetFrames" {
            n184 = Unbundle By Name(w358) -> ("Abstract_CCD.lvclass"=w363:refnum<class "Abstract_CCD.lvclass">)
            n185 = Unbundle By Name(w366) -> ("Numeric 1"=w360:dbl)
            n186 = call-dynamic "Set_Frames.vi"("error in (no error)"=w362, "Frames"=w360, "Abstract_CCD in"=w363) -> ("error out"=w361:errorcluster, "Abstract_CCD out"=w357:refnum<class "Abstract_CCD.lvclass">)  [unwired: 7 in]
            n187 = Bundle By Name(cluster=w358, "Abstract_CCD.lvclass"=w357) -> (w359:T5)
          }
          frame "Spectrometer_SetDarkspec" {
            w381 = T6 {"QueueAction"=enum."TimeOut", "Data"=[], "Data_Raw"=[], "Data_Dark"=[], "Data_Ref"=[], "Device Information"=[], "Numeric Control"=0.0, "Boolean"=FALSE, "Wavelength"=[], "Time"=[], "Time Stamp"=timestamp(0 s since 1904-01-01), "Numeric Control 2"=0.0, "TabControl"=enum."Measure"}  # DataQueue
            n188 = Unbundle By Name(w376) -> ("Abstract_CCD.lvclass"=w374:refnum<class "Abstract_CCD.lvclass">)
            n189 = call-dynamic "Measure.vi"("error in (no error)"=w373, "Abstract_CCD in"=w374) -> ("error out"=w371:errorcluster, "Data Raw"=w378:T11, "Abstract_CCD out"=w372:refnum<class "Abstract_CCD.lvclass">)  [unwired: 3 in, 4 out]
            n190 = Bundle By Name(cluster=w381, "QueueAction"=DataQueue_Action."Set_Dark", "Data_Dark"=w378) -> (w382:T6)
            n191 = Enqueue Element(queue=w380, element=w382) -> (queue out=w377:refnum<queue>)  [unwired: 2 in, 2 out]
            n192 = Bundle By Name(cluster=w376, "Abstract_CCD.lvclass"=w372) -> (w375:T5)
            n193 = property on="Measure:\nRecord_Darkspec" class="Bool (strict)"(error in=w371, "Value"=FALSE ("Record_Darkspec")) -> (error out=w369:errorcluster)  [unwired: 1 in, 1 out]
            n194 = property on="SpectralStability:\nRecord_Darkspec" class="Bool (strict)"(error in=w369, "Value"=FALSE ("SpectralStability:\nRecord_Darkspec")) -> (error out=w368:errorcluster)  [unwired: 1 in, 1 out]
          }
          frame "Spectrometer_SetReference" {
            w396 = T6 {"QueueAction"=enum."TimeOut", "Data"=[], "Data_Raw"=[], "Data_Dark"=[], "Data_Ref"=[], "Device Information"=[], "Numeric Control"=0.0, "Boolean"=FALSE, "Wavelength"=[], "Time"=[], "Time Stamp"=timestamp(0 s since 1904-01-01), "Numeric Control 2"=0.0, "TabControl"=enum."Measure"}  # DataQueue
            n195 = Unbundle By Name(w391) -> ("Abstract_CCD.lvclass"=w388:refnum<class "Abstract_CCD.lvclass">)
            n196 = call-dynamic "Measure.vi"("error in (no error)"=w389, "Abstract_CCD in"=w388) -> ("error out"=w386:errorcluster, "Data Raw"=w393:T11, "Abstract_CCD out"=w387:refnum<class "Abstract_CCD.lvclass">)  [unwired: 3 in, 4 out]
            n197 = Bundle By Name(cluster=w396, "QueueAction"=DataQueue_Action."Set_Ref", "Data_Ref"=w393) -> (w397:T6)
            n198 = Enqueue Element(queue=w395, element=w397) -> (queue out=w392:refnum<queue>)  [unwired: 2 in, 2 out]
            n199 = Bundle By Name(cluster=w391, "Abstract_CCD.lvclass"=w387) -> (w390:T5)
            n200 = property on="Record RefSpec" class="Bool (strict)"(error in=w386, "Value"=FALSE ("Record RefSpec")) -> (error out=w385:errorcluster)  [unwired: 1 in, 1 out]
          }
          frame "Spectrometer_SetTriggerMode" {
            n201 = Unbundle By Name(w402) -> ("Abstract_CCD.lvclass"=w407:refnum<class "Abstract_CCD.lvclass">)
            n202 = Unbundle By Name(w406) -> ("Numeric 1"=w404:dbl)
            n203 = call-dynamic "Set_TriggerMode.vi"("error in (no error)"=w405, "Trigger Mode"=w404, "Abstract_CCD in"=w407) -> ("error out"=w403:errorcluster, "Abstract_CCD out"=w401:refnum<class "Abstract_CCD.lvclass">)  [unwired: 7 in]
            n204 = Bundle By Name(cluster=w402, "Abstract_CCD.lvclass"=w401) -> (w400:T5)
          }
          frame "Spectrometer_DeviceInformation" {
            w415 = T6 {"QueueAction"=enum."TimeOut", "Data"=[], "Data_Raw"=[], "Data_Dark"=[], "Data_Ref"=[], "Device Information"=[], "Numeric Control"=0.0, "Boolean"=FALSE, "Wavelength"=[], "Time"=[], "Time Stamp"=timestamp(0 s since 1904-01-01), "Numeric Control 2"=0.0, "TabControl"=enum."Measure"}  # DataQueue
            n205 = Unbundle By Name(w409) -> ("Abstract_CCD.lvclass"=w417:refnum<class "Abstract_CCD.lvclass">)
            n206 = call-dynamic "Get_DeviceInformation.vi"("error in (no error)"=w416, "Abstract_CCD in"=w417) -> ("error out"=w411:errorcluster, "Array"=w418:string[])  [unwired: 7 in, 1 out]
            n207 = Bundle By Name(cluster=w415, "QueueAction"=DataQueue_Action."Transfer_Settings", "Device Information"=w418) -> (w413:T6)
            n208 = Enqueue Element(queue=w414, element=w413, error in (no error)=w411) -> (queue out=w412:refnum<queue>, error out=w410:errorcluster)  [unwired: 1 in, 1 out]
          }
          frame "Arduino_Init" {
            n209 = Unbundle By Name(w429) -> ("SpinCoater.lvclass"=w428:refnum<class "SpinCoater.lvclass">)
            n210 = call-dynamic "Init.vi"("error in (no error)"=w427, "Variant"="Port Arduino", "SpinCoater in"=w428) -> ("error out"=w424:errorcluster, "SpinCoater out"=w425:refnum<class "SpinCoater.lvclass">)  [unwired: 7 in]
            n211 = call-dynamic "IsInit.vi"("error in (no error)"=w424, "SpinCoater in"=w425) -> ("error out"=w421:errorcluster, "Init"=w422:bool, "SpinCoater out"=w423:refnum<class "SpinCoater.lvclass">)  [unwired: 7 in]
            n212 = property on="Arduino" class="Bool (strict)"("Value"=w422) -> ()  [unwired: 2 in, 2 out]
            n213 = case shown="True" w422 {
              tunnel: w432 -> [w436 w445]
              tunnel: [w436 w439] -> w431
              tunnel: [w435 w438] -> w430
              tunnel: w421 -> [w435 w442]
              frame False {
              }
              frame True {
                w446 = T9 {"QueueAction"=enum."TimeOut", "Numeric 1"=0.0, "Numeric 2"=0.0, "Boolean 1"=FALSE, "Boolean 2"=FALSE, "Spin Program"=[], "Spin Prg v07"=[], "Time Stamp"=timestamp(0 s since 1904-01-01), "TabControl"=enum."Measure"}  # Device Queue
                n214 = property on="Program Spin Coater" class="Arr (strict)"() -> ("Value"=w437:T2)  [unwired: 2 in, 2 out]
                n215 = property on="Seconds to Spin" class="DigNum (strict)"() -> ("Value"=w441:dbl[unit])  [unwired: 2 in, 2 out]
                n216 = node(w441) -> (w440:dbl)
                n217 = Bundle By Name(cluster=w446, "QueueAction"=DeviceQueue_Action."Arduino_LoadProgram", "Spin Prg v07"=w437, "Numeric 1"=w440) -> (w444:T9)
                n218 = Enqueue Element(queue=w445, element=w444, error in (no error)=w442) -> (queue out=w439:refnum<queue>, error out=w438:errorcluster)  [unwired: 1 in, 1 out]
              }
            }
            n219 = Bundle By Name(cluster=w429, "SpinCoater.lvclass"=w423) -> (w433:T5)
          }
          frame "Arduino_Close" {
            n220 = Unbundle By Name(w449) -> ("SpinCoater.lvclass"=w457:refnum<class "SpinCoater.lvclass">)
            n221 = property on="Arduino" class="Bool (strict)"() -> (error out=w451:errorcluster, "Value"=w450:bool)  [unwired: 2 in, 1 out]
            n222 = property on="Arduino" class="Bool (strict)"(error in=w451, "Value"=FALSE ("Arduino")) -> ()  [unwired: 1 in, 2 out]
            n223 = case shown="False" w450 {
              tunnel: w457 -> [w458 w463]
              tunnel: w456 -> [w459 w462]
              tunnel: [w459 w461] -> w455
              tunnel: [w458 w460] -> w448
              frame False {
              }
              frame True {
                n224 = call-dynamic "Close.vi"("error in (no error)"=w462, "SpinCoater in"=w463) -> ("error out"=w461:errorcluster, "SpinCoater out"=w460:refnum<class "SpinCoater.lvclass">)  [unwired: 8 in]
              }
            }
            n225 = Bundle By Name(cluster=w449, "SpinCoater.lvclass"=w448) -> (w447:T5)
          }
          frame "Arduino_LoadProgram" {
            n226 = Unbundle By Name(w473) -> ("Spin Prg v07"=w464:T2, "Numeric 1"=w472:dbl)
            n227 = Unbundle By Name(w468) -> ("SpinCoater.lvclass"=w471:refnum<class "SpinCoater.lvclass">)
            n228 = node(w472) -> (w470:dbl[unit])
            n229 = call-dynamic "Program_Load_v02.vi"("error in (no error)"=w469, "Time Start"=w470, "Program Spin Coater"=w464, "SpinCoater in"=w471) -> ("error out"=w466:errorcluster, "SpinCoater out"=w467:refnum<class "SpinCoater.lvclass">)  [unwired: 6 in]
            n230 = Bundle By Name(cluster=w468, "SpinCoater.lvclass"=w467) -> (w465:T5)
          }
          frame "Arduino_StartProgram" {
            n231 = Unbundle By Name(w481) -> ("SpinCoater.lvclass"=w478:refnum<class "SpinCoater.lvclass">)
            n232 = call-dynamic "Program_Run.vi"("error in (no error)"=w477, "SpinCoater in"=w478) -> ("error out"=w476:errorcluster)  [unwired: 8 in, 1 out]
            n233 = property on="Action" class="Str"("Value"="Measuring" ("Action")) -> ()  [unwired: 2 in, 2 out]
          }
          frame "Arduino_SetSpeed" {
            n234 = Unbundle By Name(w490) -> ("SpinCoater.lvclass"=w486:refnum<class "SpinCoater.lvclass">)
            n235 = Unbundle By Name(w489) -> ("Numeric 1"=w488:dbl)
            n236 = To Unsigned Long Integer(number=w488) -> (unsigned 32bit integer=w484:u32)
            n237 = call-dynamic "Debug_SetSpeed.vi"("error in (no error)"=w485, "Speed"=w484, "SpinCoater in"=w486) -> ("error out"=w483:errorcluster)  [unwired: 7 in, 1 out]
          }
          frame "Arduino_SetMillis" {
            n238 = Unbundle By Name(w496) -> ("SpinCoater.lvclass"=w495:refnum<class "SpinCoater.lvclass">)
            n239 = Unbundle By Name(w498) -> ("Numeric 1"=w500:dbl)
            n240 = To Unsigned Long Integer(number=w500) -> (unsigned 32bit integer=w492:u32)
            n241 = call-dynamic "Debug_SetMillis.vi"("error in (no error)"=w494, "Milliseconds"=w492, "SpinCoater in"=w495) -> ("error out"=w493:errorcluster)  [unwired: 7 in, 1 out]
          }
          frame "Arduino_StopSpin" {
            n242 = Unbundle By Name(w504) -> ("SpinCoater.lvclass"=w503:refnum<class "SpinCoater.lvclass">)
            n243 = call-dynamic "Stop_Spin.vi"("error in (no error)"=w502, "SpinCoater in"=w503) -> ("error out"=w501:errorcluster)  [unwired: 8 in, 1 out]
          }
          frame "Arduino_Shutter_SetPosition" {
            n244 = Unbundle By Name(w513) -> ("Numeric 1"=w512:dbl)
            n245 = Unbundle By Name(w515) -> ("SpinCoater.lvclass"=w514:refnum<class "SpinCoater.lvclass">)
            n246 = Number To Decimal String(number=w512) -> (decimal integer string=w511:string)  [unwired: 1 in]
            n247 = Concatenate Strings("!shu_M" ("string"), w511) -> (w509:string)
            n248 = call-dynamic "Send_String.vi"("error in (no error)"=w508, "String"=w509, "SpinCoater in"=w514) -> ("error out"=w507:errorcluster)  [unwired: 6 in, 2 out]
          }
          frame "Arduino_Shutter_Close" {
            n249 = Unbundle By Name(w522) -> ("SpinCoater.lvclass"=w521:refnum<class "SpinCoater.lvclass">)
            n250 = call-dynamic "Send_String.vi"("error in (no error)"=w520, "String"="!shuOFF" ("string"), "SpinCoater in"=w521) -> ("error out"=w519:errorcluster)  [unwired: 6 in, 2 out]
          }
          frame "Arduino_Shutter_Open" {
            n251 = Unbundle By Name(w529) -> ("SpinCoater.lvclass"=w528:refnum<class "SpinCoater.lvclass">)
            n252 = call-dynamic "Send_String.vi"("error in (no error)"=w527, "String"="!shuON" ("string"), "SpinCoater in"=w528) -> ("error out"=w526:errorcluster)  [unwired: 6 in, 2 out]
          }
          frame "Measure_Stop" {
            w538 = T6 {"QueueAction"=enum."TimeOut", "Data"=[], "Data_Raw"=[], "Data_Dark"=[], "Data_Ref"=[], "Device Information"=[], "Numeric Control"=0.0, "Boolean"=FALSE, "Wavelength"=[], "Time"=[], "Time Stamp"=timestamp(0 s since 1904-01-01), "Numeric Control 2"=0.0, "TabControl"=enum."Measure"}  # DataQueue
            n253 = Bundle By Name(cluster=w538, "QueueAction"=DataQueue_Action."Stop_Measurement") -> (w539:T6)
            n254 = Enqueue Element(queue=w536, element=w539, error in (no error)=w533) -> (queue out=w535:refnum<queue>, error out=w532:errorcluster)  [unwired: 1 in, 1 out]
          }
          frame "Measure_InSitu" {
            w580 = T9 {"QueueAction"=enum."TimeOut", "Numeric 1"=0.0, "Numeric 2"=0.0, "Boolean 1"=FALSE, "Boolean 2"=FALSE, "Spin Program"=[], "Spin Prg v07"=[], "Time Stamp"=timestamp(0 s since 1904-01-01), "TabControl"=enum."Measure"}  # Device Queue
            w587 = T9 {"QueueAction"=enum."TimeOut", "Numeric 1"=0.0, "Numeric 2"=0.0, "Boolean 1"=FALSE, "Boolean 2"=FALSE, "Spin Program"=[], "Spin Prg v07"=[], "Time Stamp"=timestamp(0 s since 1904-01-01), "TabControl"=enum."Measure"}  # Device Queue
            n255 = Bundle By Name(cluster=w587, "QueueAction"=DeviceQueue_Action."Spectrometer_SetTriggerMode", "Numeric 1"=1.0) -> (w585:T9)
            n256 = Bundle By Name(cluster=w580, "QueueAction"=DeviceQueue_Action."Spectrometer_DeviceInformation") -> (w577:T9)
            n257 = Bundle By Name(cluster=w577, "QueueAction"=DeviceQueue_Action."Spectrometer_StartMeasurement") -> (w573:T9)
            n258 = Enqueue Element(queue=w586, element=w585, error in (no error)=w542) -> (queue out=w582:refnum<queue>, error out=w583:errorcluster)  [unwired: 1 in, 1 out]
            n259 = property on="Frames" class="DigNum (strict)"() -> ("Value"=w543:i32)  [unwired: 2 in, 2 out]
            n260 = Bundle By Name(cluster=w573, "QueueAction"=DeviceQueue_Action."Arduino_StartProgram") -> (w568:T9)
            n261 = Enqueue Element(queue=w582, element=w577, error in (no error)=w583) -> (queue out=w579:refnum<queue>, error out=w578:errorcluster)  [unwired: 1 in, 1 out]
            n262 = Bundle By Name(cluster=w568, "QueueAction"=DeviceQueue_Action."Spectrometer_GetData", "Numeric 1"="Dividider Get Spectra") -> (w563:T9)
            n263 = Divide(x=w543, y="Dividider Get Spectra") -> (x/y=w575:dbl)
            n264 = Round Toward +Infinity(x=w575) -> (ceil(x): smallest int >= x=w574:dbl)
            n265 = Enqueue Element(queue=w579, element=w573, error in (no error)=w578) -> (queue out=w572:refnum<queue>, error out=w571:errorcluster)  [unwired: 1 in, 1 out]
            n266 = Enqueue Element(queue=w572, element=w568, error in (no error)=w571) -> (queue out=w569:refnum<queue>, error out=w566:errorcluster)  [unwired: 1 in, 1 out]
            n267 = for {
              N: w574 -> [_]
              shift-right: [w590] -> w565
              shift-left: w569 -> [w594]
              tunnel: w563 -> [w591]
              shift-right: [w592] -> w564
              shift-left: w566 -> [w593]
              n268 = Enqueue Element(queue=w594, element=w591, error in (no error)=w593) -> (queue out=w590:refnum<queue>, error out=w592:errorcluster)  [unwired: 1 in, 1 out]
            }
            n269 = Bundle By Name(cluster=w563, "QueueAction"=DeviceQueue_Action."Spectrometer_StopMeasurement") -> (w559:T9)
            n270 = property on="Measure_FramesSpectrometer" class="DigNum (strict)"() -> ("Value"=w545:dbl)  [unwired: 2 in, 2 out]
            n271 = Bundle By Name(cluster=w559, "QueueAction"=DeviceQueue_Action."Measure_Stop") -> (w552:T9)
            n272 = Enqueue Element(queue=w565, element=w559, error in (no error)=w564) -> (queue out=w560:refnum<queue>, error out=w561:errorcluster)  [unwired: 1 in, 1 out]
            n273 = Bundle By Name(cluster=w552, "QueueAction"=DeviceQueue_Action."Spectrometer_SetTriggerMode", "Numeric 1"=0.0) -> (w547:T9)
            n274 = Enqueue Element(queue=w560, element=w552, error in (no error)=w561) -> (queue out=w555:refnum<queue>, error out=w556:errorcluster)  [unwired: 1 in, 1 out]
            n275 = Bundle By Name(cluster=w547, "QueueAction"=DeviceQueue_Action."Spectrometer_SetFrames", "Numeric 1"=w545) -> (w544:T9)
            n276 = Enqueue Element(queue=w555, element=w547, error in (no error)=w556) -> (queue out=w554:refnum<queue>, error out=w553:errorcluster)  [unwired: 1 in, 1 out]
            n277 = Enqueue Element(queue=w554, element=w544, error in (no error)=w553) -> (queue out=w548:refnum<queue>, error out=w549:errorcluster)  [unwired: 1 in, 1 out]
          }
          frame "Measure_InSituAdvanced" {
            w681 = T9 {"QueueAction"=enum."TimeOut", "Numeric 1"=0.0, "Numeric 2"=0.0, "Boolean 1"=FALSE, "Boolean 2"=FALSE, "Spin Program"=[], "Spin Prg v07"=[], "Time Stamp"=timestamp(0 s since 1904-01-01), "TabControl"=enum."Measure"}  # Device Queue
            n278 = property on="Dividider Get Spectra" class="DigNum (strict)"() -> ("Value"=w640:u32)  [unwired: 2 in, 2 out]
            n279 = Bundle By Name(cluster=w681, "QueueAction"=DeviceQueue_Action."Spectrometer_SetTriggerMode", "Numeric 1"=1.0) -> (w636:T9)
            n280 = Bundle By Name(cluster=w636, "QueueAction"=DeviceQueue_Action."Spectrometer_DeviceInformation") -> (w673:T9)
            n281 = Bundle By Name(cluster=w673, "QueueAction"=DeviceQueue_Action."Spectrometer_StartMeasurement") -> (w669:T9)
            n282 = Enqueue Element(queue=w680, element=w636, error in (no error)=w641) -> (queue out=w677:refnum<queue>, error out=w678:errorcluster)  [unwired: 1 in, 1 out]
            n283 = Bundle By Name(cluster=w669, "QueueAction"=DeviceQueue_Action."Arduino_StartProgram") -> (w664:T9)
            n284 = property on="Frames" class="DigNum (strict)"() -> ("Value"=w642:i32)  [unwired: 2 in, 2 out]
            n285 = Unbundle By Name(w623) -> ("Time Stamp"=w622:timestamp)
            n286 = Enqueue Element(queue=w677, element=w673, error in (no error)=w678) -> (queue out=w675:refnum<queue>, error out=w674:errorcluster)  [unwired: 1 in, 1 out]
            n287 = Divide(x=w642, y=w640) -> (x/y=w671:dbl)
            n288 = Bundle By Name(cluster=w664, "QueueAction"=DeviceQueue_Action."Spectrometer_GetData", "Numeric 1"=w640) -> (w659:T9)
            n289 = Round Toward +Infinity(x=w671) -> (ceil(x): smallest int >= x=w670:dbl)
            n290 = Enqueue Element(queue=w675, element=w669, error in (no error)=w674) -> (queue out=w668:refnum<queue>, error out=w667:errorcluster)  [unwired: 1 in, 1 out]
            n291 = Enqueue Element(queue=w668, element=w664, error in (no error)=w667) -> (queue out=w665:refnum<queue>, error out=w662:errorcluster)  [unwired: 1 in, 1 out]
            n292 = Bundle By Name(cluster=w659, "QueueAction"=DeviceQueue_Action."Spectrometer_StopMeasurement") -> (w655:T9)
            n293 = for {
              N: w670 -> [_]
              shift-right: [w731] -> w661
              shift-left: w665 -> [w735]
              tunnel: w659 -> [w732]
              shift-right: [w733] -> w660
              shift-left: w662 -> [w734]
              n294 = Enqueue Element(queue=w735, element=w732, error in (no error)=w734) -> (queue out=w731:refnum<queue>, error out=w733:errorcluster)  [unwired: 1 in, 1 out]
            }
            n295 = property on="Measure_FramesSpectrometer" class="DigNum (strict)"() -> ("Value"=w643:dbl)  [unwired: 2 in, 2 out]
            n296 = property on="periodic time" class="DigNum (strict)"() -> ("Value"=w635:dbl[unit])  [unwired: 2 in, 2 out]
            n297 = Bundle By Name(cluster=w655, "QueueAction"=DeviceQueue_Action."Measure_Stop") -> (w648:T9)
            n298 = property on="Duration after" class="DigNum (strict)"() -> ("Value"=w634:dbl[unit])  [unwired: 2 in, 2 out]
            n299 = node(w635) -> (w605:dbl)
            n300 = property on="periodic time" class="DigNum (strict)"() -> ("Value"=w633:dbl[unit])  [unwired: 2 in, 2 out]
            n301 = Bundle By Name(cluster=w648, "QueueAction"=DeviceQueue_Action."Spectrometer_SetTriggerMode", "Numeric 1"=0.0) -> (w645:T9)
            n302 = Enqueue Element(queue=w661, element=w655, error in (no error)=w660) -> (queue out=w656:refnum<queue>, error out=w657:errorcluster)  [unwired: 1 in, 1 out]
            n303 = node(w634) -> (w628:dbl)
            n304 = Bundle By Name(cluster=w645, "QueueAction"=DeviceQueue_Action."Spectrometer_SetFrames", "Numeric 1"=w643) -> (w625:T9)
            n305 = Enqueue Element(queue=w656, element=w648, error in (no error)=w657) -> (queue out=w651:refnum<queue>, error out=w652:errorcluster)  [unwired: 1 in, 1 out]
            n306 = node(w633) -> (w627:dbl)
            n307 = Bundle By Name(cluster=w625, "QueueAction"=DeviceQueue_Action."Wait", "Numeric 1"=w605) -> (w607:T9)
            n308 = Enqueue Element(queue=w651, element=w645, error in (no error)=w652) -> (queue out=w650:refnum<queue>, error out=w649:errorcluster)  [unwired: 1 in, 1 out]
            n309 = Not Equal To 0?(x=w627) -> (x != 0?=w631:bool)
            n310 = Not Equal To 0?(x=w628) -> (x != 0?=w632:bool)
            n311 = Divide(x=w628, y=w627) -> (x/y=w629:dbl)
            n312 = Bundle By Name(cluster=w607, "QueueAction"=DeviceQueue_Action."Spectrometer_MeasureAdvanced", "Time Stamp"=w622) -> (w606:T9)
            n313 = And(x=w632, y=w631) -> (x .and. y?=w630:bool)
            n314 = Round Toward +Infinity(x=w629) -> (ceil(x): smallest int >= x=w626:dbl)
            n315 = Enqueue Element(queue=w650, element=w625, error in (no error)=w649) -> (queue out=w639:refnum<queue>, error out=w638:errorcluster)  [unwired: 1 in, 1 out]
            n316 = Bundle By Name(cluster=w606, "QueueAction"=DeviceQueue_Action."Arduino_SetSpeed", "Numeric 1"=1500.0) -> (w617:T9)
            n317 = Bundle By Name(cluster=w617, "Numeric 1"=0.0) -> (w609:T9)
            n318 = property on="Measure_FrameRate" class="DigNum (strict)"() -> ("Value"=w614:dbl[unit])  [unwired: 2 in, 2 out]
            n319 = property on="Measure_FramesSpectrometer" class="DigNum (strict)"() -> ("Value"=w613:dbl)  [unwired: 2 in, 2 out]
            n320 = Divide(x=w613, y=w614) -> (x/y=w615:dbl[unit])
            n321 = Bundle By Name(cluster=w607, "Numeric 1"=1.0) -> (w610:T9)
            n322 = node(w615) -> (w604:dbl)
            n323 = Subtract(x=w605, y=w604) -> (x-y=w603:dbl)
            n324 = Bundle By Name(cluster=w607, "Numeric 1"=w603) -> (w602:T9)
            n325 = Round Toward +Infinity(x=w604) -> (ceil(x): smallest int >= x=w616:dbl)
            n326 = Add(x=w616, y=2.0) -> (x+y=w611:dbl)
            n327 = Bundle By Name(cluster=w610, "Numeric 1"=w611) -> (w599:T9)
            n328 = case shown="True" w630 {
              tunnel: w639 -> [w685 w687]
              tunnel: w638 -> [w684 w690]
              tunnel: w626 -> [_ w703]
              tunnel: w606 -> [_ w702]
              tunnel: w602 -> [_ w698]
              tunnel: w617 -> [_ w697]
              tunnel: w610 -> [_ w696]
              tunnel: w606 -> [_ w695]
              tunnel: w599 -> [_ w694]
              tunnel: w609 -> [_ w693]
              tunnel: [w684 w692] -> w601
              tunnel: [w685 w691] -> w600
              tunnel: w607 -> [_ w686]
              frame False {
              }
              frame True {
                n329 = Enqueue Element(queue=w687, element=w686, error in (no error)=w690) -> (queue out=w688:refnum<queue>, error out=w689:errorcluster)  [unwired: 1 in, 1 out]
                n330 = for {
                  N: w703 -> [_]
                  shift-right: [w724] -> w700
                  shift-left: w688 -> [w730]
                  shift-right: [w723] -> w699
                  shift-left: w689 -> [w729]
                  tunnel: w702 -> [w728]
                  tunnel: w698 -> [w725]
                  n331 = Enqueue Element(queue=w730, element=w728, error in (no error)=w729) -> (queue out=w726:refnum<queue>, error out=w727:errorcluster)  [unwired: 1 in, 1 out]
                  n332 = Enqueue Element(queue=w726, element=w725, error in (no error)=w727) -> (queue out=w724:refnum<queue>, error out=w723:errorcluster)  [unwired: 1 in, 1 out]
                }
                n333 = case shown="True" "Spin at end" {
                  tunnel: w700 -> [w705 w722]
                  tunnel: w699 -> [w704 w721]
                  tunnel: w697 -> [_ w716]
                  tunnel: w696 -> [_ w715]
                  tunnel: w695 -> [_ w714]
                  tunnel: w694 -> [_ w709]
                  tunnel: w693 -> [_ w708]
                  tunnel: [w704 w707] -> w692
                  tunnel: [w705 w706] -> w691
                  frame False {
                  }
                  frame True {
                    n334 = Enqueue Element(queue=w722, element=w716, error in (no error)=w721) -> (queue out=w720:refnum<queue>, error out=w719:errorcluster)  [unwired: 1 in, 1 out]
                    n335 = Enqueue Element(queue=w720, element=w715, error in (no error)=w719) -> (queue out=w718:refnum<queue>, error out=w717:errorcluster)  [unwired: 1 in, 1 out]
                    n336 = Enqueue Element(queue=w718, element=w714, error in (no error)=w717) -> (queue out=w713:refnum<queue>, error out=w712:errorcluster)  [unwired: 1 in, 1 out]
                    n337 = Enqueue Element(queue=w713, element=w709, error in (no error)=w712) -> (queue out=w710:refnum<queue>, error out=w711:errorcluster)  [unwired: 1 in, 1 out]
                    n338 = Enqueue Element(queue=w710, element=w708, error in (no error)=w711) -> (queue out=w706:refnum<queue>, error out=w707:errorcluster)  [unwired: 1 in, 1 out]
                  }
                }
              }
            }
            n339 = Bundle By Name(cluster=w599, "QueueAction"=DeviceQueue_Action."Arduino_Shutter_Close") -> (w598:T9)
            n340 = Enqueue Element(queue=w600, element=w598, error in (no error)=w601) -> (queue out=w596:refnum<queue>, error out=w595:errorcluster)  [unwired: 1 in, 1 out]
            "Nr After Spin" <- u16 0 ("Nr After Spin")
          }
          frame "Measure_Spectrum" {
            n341 = Unbundle By Name(w736) -> ("Time Stamp"=w737:timestamp)
            n342 = Bundle By Name(cluster=w736, "QueueAction"=DeviceQueue_Action."Spectrometer_Measure", "Time Stamp"=w737) -> (w742:T9)
            n343 = Bundle By Name(cluster=w742, "QueueAction"=DeviceQueue_Action."Measure_Stop") -> (w740:T9)
            n344 = Enqueue Element(queue=w748, element=w742, error in (no error)=w747) -> (queue out=w743:refnum<queue>, error out=w744:errorcluster)  [unwired: 1 in, 1 out]
            n345 = Enqueue Element(queue=w743, element=w740, error in (no error)=w744) -> (queue out=w739:refnum<queue>, error out=w738:errorcluster)  [unwired: 1 in, 1 out]
          }
          frame "Measure_SpectralStability" {
            n346 = Bundle By Name(cluster=w752, "QueueAction"=DeviceQueue_Action."Spectrometer_DeviceInformation") -> (w755:T9)
            n347 = property on="SpectralStability_\nFrameRate" class="DigNum (strict)"() -> ("Value"=w775:dbl[unit])  [unwired: 2 in, 2 out]
            n348 = property on="SpectralStability_\nFramesSpectrometer" class="DigNum (strict)"() -> ("Value"=w776:dbl)  [unwired: 2 in, 2 out]
            n349 = Bundle By Name(cluster=w755, "QueueAction"=DeviceQueue_Action."Spectrometer_Measure") -> (w754:T9)
            n350 = Enqueue Element(queue=w758, element=w755, error in (no error)=w757) -> (queue out=w760:refnum<queue>, error out=w759:errorcluster)  [unwired: 1 in, 1 out]
            n351 = Divide(x=w776, y=w775) -> (x/y=w770:dbl[unit])
            n352 = Unbundle By Name(w752) -> ("Numeric 1"=w751:dbl)
            n353 = Subtract(x="SpectralStability_\nPeriodicTime", y=w770) -> (x-y=w769:dbl[unit])
            n354 = Enqueue Element(queue=w760, element=w754, error in (no error)=w759) -> (queue out=w774:refnum<queue>, error out=w773:errorcluster)  [unwired: 1 in, 1 out]
            n355 = node(w769) -> (w768:dbl)
            n356 = Decrement(x=w751) -> (x-1=w750:dbl)
            n357 = Bundle By Name(cluster=w754, "QueueAction"=DeviceQueue_Action."Wait", "Numeric 1"=w768) -> (w764:T9)
            n358 = for {
              N: w750 -> [_]
              shift-right: [w780] -> w767
              shift-left: w774 -> [w786]
              shift-right: [w779] -> w766
              shift-left: w773 -> [w785]
              tunnel: w764 -> [w782]
              tunnel: w754 -> [w781]
              n359 = Enqueue Element(queue=w786, element=w782, error in (no error)=w785) -> (queue out=w784:refnum<queue>, error out=w783:errorcluster)  [unwired: 1 in, 1 out]
              n360 = Enqueue Element(queue=w784, element=w781, error in (no error)=w783) -> (queue out=w780:refnum<queue>, error out=w779:errorcluster)  [unwired: 1 in, 1 out]
            }
            n361 = Bundle By Name(cluster=w764, "QueueAction"=DeviceQueue_Action."Measure_Stop") -> (w763:T9)
            n362 = Enqueue Element(queue=w767, element=w763, error in (no error)=w766) -> (queue out=w761:refnum<queue>, error out=w762:errorcluster)  [unwired: 1 in, 1 out]
          }
        }
      }
      frame Error {
        w791 = T12 4 items=["no dialog", "OK message", "continue or stop message", "OK message + warnings", "continue/stop + warnings"] ("type of dialog (OK msg:1)")
        n363 = call <vilib>:"General Error Handler.vi"("type of dialog (OK msg:1)"=w791, "error in (no error)"=w792) -> ("error out"=w790:errorcluster)  [unwired: 9 in, 4 out]
        n364 = call <vilib>:"Clear Errors.vi"("error in (no error)"=w790) -> ("error out"=w789:errorcluster)  [unwired: 5 in, 1 out]
      }
    }
  }
  n365 = while {
    shift-right: [w794] -> _
    shift-left: w8 -> [w800]
    shift-right: [w795] -> _
    shift-left: w7 -> [w799]
    shift-right: [w796] -> _
    shift-left: w6 -> [w798]
    stop <- w797 stop-if-true
    # "Consumer Data"
    n366 = case shown="No Error" w800 {
      selector: w800 -> [w811 w1565]
      tunnel: w799 -> [w810 w1566]
      tunnel: w798 -> [w808 w1563]
      tunnel: [w807 _] -> w797
      tunnel: [w806 w1563] -> w796
      tunnel: [w805 w1566] -> w795
      tunnel: [w803 w1564] -> w794
      frame No Error {
        n367 = Dequeue Element(queue=w810, error in (no error)=w811) -> (queue out=w804:refnum<queue>, element=w801:T6, error out=w802:errorcluster)  [unwired: 1 in, 1 out]
        n368 = Unbundle By Name(w801) -> ("QueueAction"=w809:T7)
        n369 = case shown="\"Measure_InSituSpinCoating\"" w809 {
          tunnel: w808 -> [w812 w817 w820 w1026 w1131 w1233 w1445 w1481 w1490 w1513 w1526 w1533]
          tunnel: [_ TRUE _ _ _ _ _ _ _ _ _ _] -> w807
          tunnel: [w812 w817 w819 w1026 w1131 w1224 w1445 w1485 w1504 w1512 w1526 w1532] -> w806
          tunnel: [w814 w816 w834 w1032 w1137 w1217 w1468 w1486 w1505 w1509 w1528 w1539] -> w805
          tunnel: w804 -> [w814 w816 w832 w1033 w1138 w1228 w1468 w1486 w1505 w1509 w1528 w1539]
          tunnel: [w813 w815 w833 w1031 w1136 w1218 w1467 w1487 w1506 w1510 w1527 w1536] -> w803
          tunnel: w802 -> [w813 w815 w831 w1034 w1139 w1227 w1467 w1487 w1506 w1510 w1527 w1536]
          tunnel: w801 -> [_ _ w826 _ _ w1220 w1458 w1488 w1507 w1511 w1517 w1538]
          frame "TimeOut", Default {
          }
          frame "Close_Program" {
          }
          frame "Measure_InSituSpinCoating" {
            w829 = T6 {"QueueAction"=enum."TimeOut", "Data"=[], "Data_Raw"=[], "Data_Dark"=[], "Data_Ref"=[], "Device Information"=[], "Numeric Control"=0.0, "Boolean"=FALSE, "Wavelength"=[], "Time"=[], "Time Stamp"=timestamp(0 s since 1904-01-01), "Numeric Control 2"=0.0, "TabControl"=enum."Measure"}  # DataQueue
            n370 = property on="Seconds to\nSpin Start" class="DigNum (strict)"() -> ("Value"=w822:dbl[unit])  [unwired: 2 in, 2 out]
            n371 = Unbundle By Name(w826) -> ("Time Stamp"=w825:timestamp)
            n372 = node(w822) -> (w821:dbl)
            n373 = Obtain Queue(name (unnamed)="Temp", element data type=w829) -> (queue out=w828:refnum<queue>)  [unwired: 3 in, 2 out]
            n374 = while {
              shift-right: [w844] -> w834
              shift-left: w832 -> [w853]
              shift-right: [w845] -> w833
              shift-left: w831 -> [w852]
              shift-right: [w846] -> w827
              shift-left: w828 -> [w847]
              tunnel: w825 -> [w840]
              shift-right: [w841] -> _
              shift-left: string[] [] ("Device Information") -> [w842]
              border: FALSE -> [_]
              tunnel: w821 -> [w837]
              shift-right: [w835] -> w819
              shift-left: w820 -> [w836]
              stop <- w843 stop-if-true
              n375 = Dequeue Element(queue=w853, error in (no error)=w852) -> (queue out=w848:refnum<queue>, element=w850:T6, error out=w849:errorcluster)  [unwired: 1 in, 1 out]
              n376 = Unbundle By Name(w850) -> ("QueueAction"=w851:T7)
              n377 = feedback #1() -> (w839:bool)
              n378 = case shown="\"Stop_Measurement\"" w851 {
                tunnel: w850 -> [w862 w872 _ w920 w938 w947 w979 w1024]
                tunnel: w849 -> [w861 w873 w880 w917 w936 w945 w970 w1021]
                tunnel: w848 -> [w857 w874 w879 w916 w937 w946 w978 w1022]
                tunnel: w847 -> [w860 w869 w881 w911 w934 w943 w967 w1025]
                tunnel: [w859 w869 w876 w908 w934 w943 w967 w1025] -> w846
                tunnel: [w858 w870 w878 w907 w936 w945 w968 w1021] -> w845
                tunnel: [w857 w871 w877 w906 w937 w946 w978 w1022] -> w844
                tunnel: [_ TRUE TRUE TRUE _ _ _ _] -> w843
                tunnel: w842 -> [w856 w867 w888 w918 w935 w944 w965 _]
                tunnel: [w856 w867 w888 w918 w935 w944 w965 w1023] -> w841
                tunnel: w840 -> [_ _ _ w919 _ _ w980 _]
                tunnel: w839 -> [w855 w866 w887 w905 w930 w939 w963 w1020]
                tunnel: [w855 w866 w887 w905 w930 w939 TRUE w1020] -> w838
                tunnel: w837 -> [_ _ _ w902 _ _ _ _]
                tunnel: w836 -> [w854 w863 w875 w897 w933 w942 w948 w1019]
                tunnel: [w854 w863 w875 w897 w931 w940 w948 w1019] -> w835
                frame Default {
                  n379 = Enqueue Element(queue=w860, element=w862, error in (no error)=w861) -> (queue out=w859:refnum<queue>, error out=w858:errorcluster)  [unwired: 1 in, 1 out]
                }
                frame "Close_Program" {
                  n380 = Enqueue Element At Opposite End(queue=w874, element=w872, error in (no error)=w873) -> (queue out=w871:refnum<queue>, error out=w870:errorcluster)  [unwired: 1 in, 1 out]
                  n381 = property on="Time.spin" class="Ref (strict)"() -> ("Value"=w864:refnum<file>)  [unwired: 2 in, 2 out]
                  n382 = property on="Meas.spin" class="Ref (strict)"() -> ("Value"=w865:refnum<file>)  [unwired: 2 in, 2 out]
                  n383 = Close File(refnum=w865) -> ()  [unwired: 1 in, 2 out]
                  n384 = Close File(refnum=w864) -> ()  [unwired: 1 in, 2 out]
                }
                frame "Abort" {
                  n385 = property on="Time.spin" class="Ref (strict)"() -> ("Value"=w885:refnum<file>)  [unwired: 2 in, 2 out]
                  n386 = Get Queue Status(queue=w881) -> (queue out=w882:refnum<queue>, # elements in queue=w883:i32)  [unwired: 2 in, 6 out]
                  n387 = property on="Meas.spin" class="Ref (strict)"() -> ("Value"=w886:refnum<file>)  [unwired: 2 in, 2 out]
                  n388 = Close File(refnum=w886) -> ()  [unwired: 1 in, 2 out]
                  n389 = Close File(refnum=w885) -> ()  [unwired: 1 in, 2 out]
                  n390 = for {
                    N: w883 -> [_]
                    shift-right: [w895] -> w876
                    shift-left: w882 -> [w896]
                    shift-right: [w892] -> w877
                    shift-left: w879 -> [w893]
                    shift-right: [w890] -> w878
                    shift-left: w880 -> [w891]
                    n391 = Dequeue Element(queue=w896) -> (queue out=w895:refnum<queue>, element=w894:T6)  [unwired: 2 in, 2 out]
                    n392 = Enqueue Element(queue=w893, element=w894, error in (no error)=w891) -> (queue out=w892:refnum<queue>, error out=w890:errorcluster)  [unwired: 1 in, 1 out]
                  }
                  n393 = property on="StartMeasurement_Button" class="Bool (strict)"("Value"=FALSE ("StartMeasurement_Button")) -> ()  [unwired: 2 in, 2 out]
                }
                frame "Stop_Measurement" {
                  n394 = property on="Automatically \nadjust count" class="Bool (strict)"() -> ("Value"=w899:bool)  [unwired: 2 in, 2 out]
                  n395 = property on="Reset Count\nafter Spin Coating" class="Bool (strict)"() -> ("Value"=w900:bool)  [unwired: 2 in, 2 out]
                  n396 = Or(x=w899, y=w900) -> (x .or. y?=w898:bool)
                  n397 = Bundle By Name(cluster=w920, "QueueAction"=DataQueue_Action."Save_InSitu", "Time Stamp"=w919, "Device Information"=w918, "Numeric Control"=w902) -> (w915:T6)
                  n398 = case shown="True" w898 {
                    frame False {
                    }
                    frame True {
                      n399 = property on="Spectra \nCount" class="DigNum (strict)"("Value"=u16 0 ("Spectra Count")) -> ()  [unwired: 2 in, 2 out]
                    }
                  }
                  n400 = Enqueue Element(queue=w916, element=w915, error in (no error)=w917) -> (queue out=w913:refnum<queue>, error out=w912:errorcluster)  [unwired: 1 in, 1 out]
                  n401 = Get Queue Status(queue=w911) -> (queue out=w909:refnum<queue>, # elements in queue=w910:i32)  [unwired: 2 in, 6 out]
                  n402 = property on="Time.spin" class="Ref (strict)"() -> ("Value"=w903:refnum<file>)  [unwired: 2 in, 2 out]
                  n403 = property on="StartMeasurement_Button" class="Bool (strict)"("Value"=FALSE ("StartMeasurement_Button")) -> ()  [unwired: 2 in, 2 out]
                  n404 = property on="Meas.spin" class="Ref (strict)"() -> ("Value"=w904:refnum<file>)  [unwired: 2 in, 2 out]
                  n405 = for {
                    N: w910 -> [_]
                    shift-right: [w928] -> w908
                    shift-left: w909 -> [w929]
                    shift-right: [w925] -> w906
                    shift-left: w913 -> [w926]
                    shift-right: [w923] -> w907
                    shift-left: w912 -> [w924]
                    n406 = Dequeue Element(queue=w929) -> (queue out=w928:refnum<queue>, element=w927:T6)  [unwired: 2 in, 2 out]
                    n407 = Enqueue Element(queue=w926, element=w927, error in (no error)=w924) -> (queue out=w925:refnum<queue>, error out=w923:errorcluster)  [unwired: 1 in, 1 out]
                  }
                  n408 = Close File(refnum=w904) -> ()  [unwired: 1 in, 2 out]
                  n409 = Close File(refnum=w903) -> ()  [unwired: 1 in, 2 out]
                }
                frame "Set_Ref" {
                  n410 = Unbundle By Name(w938) -> ("Data_Ref"=w932:T11)
                  n411 = Bundle By Name(cluster=w933, "Ref"=w932) -> (w931:T4)
                }
                frame "Set_Dark" {
                  n412 = Unbundle By Name(w947) -> ("Data_Dark"=w941:T11)
                  n413 = Bundle By Name(cluster=w942, "Dark"=w941) -> (w940:T4)
                }
                frame "Spectrometer_Measure" {
                  w953 = FALSE ("prepend array or string size? (T)")
                  w966 = enum16{"start", "end", "current"}."end" ("from (0:start)")
                  n414 = Unbundle By Name(w979) -> ("Data_Raw"=w975:T11, "Time"=w969:dbl[])
                  n415 = property on="LowerWLLimit" class="DigNum (strict)"() -> ("Value"=w950:i32)  [unwired: 2 in, 2 out]
                  n416 = To Unsigned Long Integer(number=w969) -> (unsigned 32bit integer=w955:u32[])
                  n417 = Index Array(array=w975, index=0) -> (element=w974:T14)
                  n418 = Unbundle By Name(w974) -> ("Image"=w952:dbl[][][])
                  n419 = property on="UpperWLLimit" class="DigNum (strict)"() -> ("Value"=w949:i32)  [unwired: 2 in, 2 out]
                  n420 = call "Trim_Spectra.vi"("WL_UpperIndex"=w949, "WL_LowerIndex"=w950, "Image"=w952) -> ("ImageCut"=w951:dbl[][][])
                  n421 = case shown="False" w963 {
                    tunnel: w980 -> [w1012 _]
                    tunnel: w970 -> [w1007 w1018]
                    tunnel: [w993 w1018] -> w957
                    tunnel: [w981 _] -> w958
                    tunnel: [w992 w1017] -> w960
                    tunnel: [w982 w1016] -> w959
                    tunnel: w951 -> [w990 _]
                    frame False {
                      w1002 = T13."open or create" ("operation (0:open)")
                      w1001 = "_" ("string")
                      n422 = property on="Measure_FileName" class="Str"() -> ("Value"=w1010:string)  [unwired: 2 in, 2 out]
                      n423 = Concatenate Strings(w1010, "_meas.spin" ("string")) -> (w1013:string)
                      n424 = Concatenate Strings(w1010, "_time.spin" ("string")) -> (w1005:string)
                      n425 = Format Date/Time String(time format string (%c)="%Y%m%d_%H%M%S", seconds (now)=w1012) -> (date/time string=w1006:string)  [unwired: 1 in]
                      n426 = property on="Measure_SavePath" class="Path"() -> ("Value"=w984:path)  [unwired: 2 in, 2 out]
                      n427 = Concatenate Strings(w1006, w1001, w1013) -> (w1011:string)
                      n428 = Concatenate Strings(w1006, w1001, w1005) -> (w1004:string)
                      n429 = property on="Frames" class="DigNum (strict)"() -> ("Value"=w983:i32)  [unwired: 2 in, 2 out]
                      n430 = Build Path(base path=w984, name or relative path=w1011) -> (appended path=w1008:path)
                      n431 = Build Path(base path=w984, name or relative path=w1004) -> (appended path=w1003:path)
                      n432 = Array Size(array=w990) -> (size(s)=w989:i32[])
                      n433 = Open/Create/Replace File(file path (use dialog)=w1008, error in=w1007, operation (0:open)=w1002) -> (refnum out=w1000:refnum<file>, error out=w999:errorcluster)  [unwired: 3 in, 1 out]
                      "Meas.spin" <- w1000
                      n434 = Open/Create/Replace File(file path (use dialog)=w1003, error in=w1007, operation (0:open)=w1002) -> (refnum out=w998:refnum<file>, error out=w997:errorcluster)  [unwired: 3 in, 1 out]
                      n435 = Write to Binary File(file (use dialog)=w1000, data=w983, error in=w999) -> (refnum out=w996:refnum<file>, error out=w995:errorcluster)  [unwired: 3 in, 1 out]
                      n436 = Index Array(array=w989, index #1=2 ("index"), index #2=1 ("index")) -> (element #1=w985:i32, element #2=w986:i32)
                      n437 = Write to Binary File(file (use dialog)=w998, data=w983, error in=w997) -> (refnum out=w982:refnum<file>, error out=w981:errorcluster)  [unwired: 3 in, 1 out]
                      "Time.spin" <- w982
                      n438 = Write to Binary File(file (use dialog)=w996, data=w986, error in=w995) -> (refnum out=w991:refnum<file>, error out=w994:errorcluster)  [unwired: 3 in, 1 out]
                      n439 = Write to Binary File(file (use dialog)=w991, data=w985, error in=w994) -> (refnum out=w992:refnum<file>, error out=w993:errorcluster)  [unwired: 3 in, 1 out]
                    }
                    frame True {
                      n440 = property on="Time.spin" class="Ref (strict)"() -> ("Value"=w1016:refnum<file>)  [unwired: 2 in, 2 out]
                      n441 = property on="Meas.spin" class="Ref (strict)"() -> ("Value"=w1017:refnum<file>)  [unwired: 2 in, 2 out]
                    }
                  }
                  n442 = To Unsigned Word Integer(number=w951) -> (unsigned 16bit integer=w954:u16[][][])
                  n443 = Merge Errors(w957, w958) -> (w956:errorcluster)
                  n444 = Set File Position(refnum=w960, from (0:start)=w966, error in=w956) -> (refnum out=w972:refnum<file>, error out=w971:errorcluster)  [unwired: 1 in]
                  n445 = Set File Position(refnum=w959, from (0:start)=w966, error in=w956) -> (refnum out=w977:refnum<file>, error out=w976:errorcluster)  [unwired: 1 in]
                  n446 = Write to Binary File(file (use dialog)=w977, data=w955, error in=w976, 5:w953) -> (error out=w961:errorcluster)  [unwired: 2 in, 2 out]
                  n447 = Write to Binary File(file (use dialog)=w972, data=w954, error in=w971, 5:w953) -> (error out=w962:errorcluster)  [unwired: 2 in, 2 out]
                  n448 = Merge Errors(w962, w961) -> (w968:errorcluster)
                }
                frame "Transfer_Settings" {
                  n449 = Unbundle By Name(w1024) -> ("Device Information"=w1023:string[])
                }
              }
              n450 = feedback-in #1(w838) -> ()
            }
            n451 = Release Queue(queue=w827) -> ()  [unwired: 2 in, 3 out]
          }
          frame "Measure_Spectrum" {
            w1029 = T6 {"QueueAction"=enum."TimeOut", "Data"=[], "Data_Raw"=[], "Data_Dark"=[], "Data_Ref"=[], "Device Information"=[], "Numeric Control"=0.0, "Boolean"=FALSE, "Wavelength"=[], "Time"=[], "Time Stamp"=timestamp(0 s since 1904-01-01), "Numeric Control 2"=0.0, "TabControl"=enum."Measure"}  # DataQueue
            n452 = Obtain Queue(name (unnamed)="Temp", element data type=w1029) -> (queue out=w1028:refnum<queue>)  [unwired: 3 in, 2 out]
            n453 = while {
              shift-right: [w1038] -> w1032
              shift-left: w1033 -> [w1046]
              shift-right: [w1039] -> w1031
              shift-left: w1034 -> [w1047]
              shift-right: [w1040] -> w1027
              shift-left: w1028 -> [w1042]
              tunnel: w1026 -> [w1036]
              stop <- w1037 stop-if-true
              n454 = Dequeue Element(queue=w1046, error in (no error)=w1047) -> (queue out=w1044:refnum<queue>, element=w1041:T6, error out=w1043:errorcluster)  [unwired: 1 in, 1 out]
              n455 = Unbundle By Name(w1041) -> ("QueueAction"=w1045:T7, "TabControl"=w1035:T8)
              n456 = case shown="\"Spectrometer_Measure\"" w1045 {
                tunnel: w1044 -> [w1048 w1076 w1116]
                tunnel: w1043 -> [w1051 w1086 w1115]
                tunnel: w1042 -> [w1053 w1092 w1118]
                tunnel: w1041 -> [w1049 w1065 _]
                tunnel: [w1052 w1092 w1114] -> w1040
                tunnel: [w1050 w1077 w1112] -> w1039
                tunnel: [w1048 w1076 w1113] -> w1038
                tunnel: [_ _ TRUE] -> w1037
                tunnel: w1036 -> [_ w1069 _]
                tunnel: w1035 -> [_ w1063 w1110]
                frame Default {
                  n457 = Enqueue Element(queue=w1053, element=w1049, error in (no error)=w1051) -> (queue out=w1052:refnum<queue>, error out=w1050:errorcluster)  [unwired: 1 in, 1 out]
                }
                frame "Spectrometer_Measure" {
                  n458 = Unbundle By Name(w1065) -> ("Data_Raw"=w1083:T11)
                  n459 = case shown="\"Spectral Stability\"" w1063 {
                    tunnel: [w1105 "SpectralStability_SavePath"] -> w1056
                    tunnel: [w1104 "SpectralStability_FileName"] -> w1054
                    tunnel: [w1100 "SpectralStability_Comments"] -> w1057
                    frame "Measure", Default {
                      n460 = property on="Spectra Count" class="DigNum (strict)"() -> ("Value"=w1106:u16)  [unwired: 2 in, 2 out]
                      n461 = property on="Measure_SavePath" class="Path"() -> ("Value"=w1105:path)  [unwired: 2 in, 2 out]
                      n462 = property on="Measure_Comments" class="Str"() -> ("Value"=w1100:string)  [unwired: 2 in, 2 out]
                      n463 = property on="Measure_FileName" class="Str"() -> ("Value"=w1101:string)  [unwired: 2 in, 2 out]
                      n464 = Number To Decimal String(number=w1106) -> (decimal integer string=w1102:string)  [unwired: 1 in]
                      n465 = Concatenate Strings(w1101, "_", w1102) -> (w1104:string)
                    }
                    frame "Spectral Stability" {
                    }
                  }
                  n466 = Index Array(array=w1083, index=0) -> (element=w1081:T14)
                  n467 = Unbundle By Name(w1065) -> ("Time Stamp"=w1064:timestamp)
                  n468 = Unbundle By Name(w1081) -> ("Image"=w1059:dbl[][][])
                  n469 = Index Array(array=w1059, index (dim 1)=0 ("disabled index (row)")) -> (element=w1075:dbl[][])  [unwired: 2 in]
                  n470 = Transpose 2D Array(2D array=w1075) -> (transposed array=w1072:dbl[][])
                  n471 = Format Date/Time String(time format string (%c)="%Y%m%d_%H%M%S", seconds (now)=w1064) -> (date/time string=w1090:string)  [unwired: 1 in]
                  n472 = Matrix Size(0:w1072) -> (2:w1073:i32)  [unwired: 1 out]
                  n473 = Empty String/Path?(string/path=w1057) -> (empty?=w1058:bool)
                  n474 = Reciprocal(x=w1073) -> (1/x=w1074:dbl)
                  n475 = Concatenate Strings(w1090, "_") -> (w1055:string)
                  n476 = case shown="False" w1058 {
                    tunnel: w1057 -> [w1099 _]
                    tunnel: w1056 -> [w1098 _]
                    tunnel: w1055 -> [w1097 _]
                    tunnel: w1054 -> [w1096 _]
                    frame False {
                      n477 = Concatenate Strings(w1097, w1096, "_comments.txt" ("string")) -> (w1093:string)
                      n478 = Build Path(base path=w1098, name or relative path=w1093) -> (appended path=w1094:path)
                      n479 = Write to Text File(file (use dialog)=w1094, text=w1099) -> ()  [unwired: 2 in, 3 out]
                    }
                    frame True {
                    }
                  }
                  n480 = Initialize Array(w1074, w1073) -> (w1071:dbl[])
                  n481 = Concatenate Strings(w1055, w1054, ".spectra" ("string")) -> (w1061:string)
                  n482 = Unbundle By Name(w1069) -> ("Wavlength"=w1066:dbl[unit][])
                  n483 = call-poly <vilib>:"A x B.vi"("Vector"=w1071, "A"=w1072) -> ("A x Vector"=w1060:dbl[])  [unwired: 1 out]
                  n484 = Build Path(base path=w1056, name or relative path=w1061) -> (appended path=w1088:path)
                  n485 = Bundle("Wavlength"=w1066, "A x Vector"=w1060) -> (w1068:T15)  [unwired: 1 in]
                  n486 = Open/Create/Replace File(file path (use dialog)=w1088, error in=w1086, operation (0:open)=T13."open or create") -> (refnum out=w1085:refnum<file>, error out=w1084:errorcluster)  [unwired: 3 in, 1 out]
                  n487 = Build Array(w1068) -> (w1067:T16)
                  n488 = To Unsigned Word Integer(number=w1059) -> (unsigned 16bit integer=w1080:u16[][][])
                  n489 = property on="Measure_Graph" class="XYGraph (strict)"("Value"=w1067) -> ()  [unwired: 2 in, 2 out]
                  n490 = Write to Binary File(file (use dialog)=w1085, data=w1080, error in=w1084) -> (refnum out=w1078:refnum<file>, error out=w1079:errorcluster)  [unwired: 3 in, 1 out]
                  n491 = Close File(refnum=w1078, error in=w1079) -> (error out=w1077:errorcluster)  [unwired: 1 out]
                }
                frame "Stop_Measurement" {
                  w1111 = FALSE ("Measure Spectrum")
                  n492 = case shown="Default" w1110 {
                    frame Default {
                    }
                    frame "Measure" {
                      n493 = property on="Automatically \nadjust count" class="Bool (strict)"() -> ("Value"=w1121:bool)  [unwired: 2 in, 2 out]
                      n494 = case shown="True" w1121 {
                        frame False {
                        }
                        frame True {
                          n495 = Increment(x="Spectra Count") -> (x+1=w1122:u16)
                          n496 = property on="Spectra Count" class="DigNum (strict)"("Value"=w1122) -> ()  [unwired: 2 in, 2 out]
                        }
                      }
                    }
                  }
                  n497 = Get Queue Status(queue=w1118) -> (queue out=w1119:refnum<queue>, # elements in queue=w1117:i32)  [unwired: 2 in, 6 out]
                  n498 = property on="SpectralStability_MeasureSpectrum" class="Bool (strict)"("Value"=w1111) -> ()  [unwired: 2 in, 2 out]
                  n499 = property on="Measure_MeasureSpectrum" class="Bool (strict)"("Value"=w1111) -> ()  [unwired: 2 in, 2 out]
                  n500 = for {
                    N: w1117 -> [_]
                    shift-right: [w1129] -> w1114
                    shift-left: w1119 -> [w1130]
                    shift-right: [w1126] -> w1113
                    shift-left: w1116 -> [w1127]
                    shift-right: [w1124] -> w1112
                    shift-left: w1115 -> [w1125]
                    n501 = Dequeue Element(queue=w1130) -> (queue out=w1129:refnum<queue>, element=w1128:T6)  [unwired: 2 in, 2 out]
                    n502 = Enqueue Element(queue=w1127, element=w1128, error in (no error)=w1125) -> (queue out=w1126:refnum<queue>, error out=w1124:errorcluster)  [unwired: 1 in, 1 out]
                  }
                }
              }
            }
            n503 = Release Queue(queue=w1027) -> ()  [unwired: 2 in, 3 out]
          }
          frame "Measure_SpectrumAdvanced" {
            w1134 = T6 {"QueueAction"=enum."TimeOut", "Data"=[], "Data_Raw"=[], "Data_Dark"=[], "Data_Ref"=[], "Device Information"=[], "Numeric Control"=0.0, "Boolean"=FALSE, "Wavelength"=[], "Time"=[], "Time Stamp"=timestamp(0 s since 1904-01-01), "Numeric Control 2"=0.0, "TabControl"=enum."Measure"}  # DataQueue
            n504 = Obtain Queue(name (unnamed)="Temp", element data type=w1134) -> (queue out=w1133:refnum<queue>)  [unwired: 3 in, 2 out]
            n505 = while {
              shift-right: [w1142] -> w1137
              shift-left: w1138 -> [w1150]
              shift-right: [w1143] -> w1136
              shift-left: w1139 -> [w1151]
              shift-right: [w1144] -> w1132
              shift-left: w1133 -> [w1146]
              tunnel: w1131 -> [w1140]
              stop <- w1141 stop-if-true
              n506 = Dequeue Element(queue=w1150, error in (no error)=w1151) -> (queue out=w1148:refnum<queue>, element=w1145:T6, error out=w1147:errorcluster)  [unwired: 1 in, 1 out]
              n507 = Unbundle By Name(w1145) -> ("QueueAction"=w1149:T7)
              n508 = case shown="\"Stop_Measurement\"" w1149 {
                tunnel: w1148 -> [w1152 w1176 w1202]
                tunnel: w1147 -> [w1155 w1186 w1201]
                tunnel: w1146 -> [w1157 w1195 w1204]
                tunnel: w1145 -> [w1153 w1163 _]
                tunnel: [w1156 w1195 w1200] -> w1144
                tunnel: [w1154 w1177 w1198] -> w1143
                tunnel: [w1152 w1176 w1199] -> w1142
                tunnel: [_ _ TRUE] -> w1141
                tunnel: w1140 -> [_ w1168 _]
                frame Default {
                  n509 = Enqueue Element(queue=w1157, element=w1153, error in (no error)=w1155) -> (queue out=w1156:refnum<queue>, error out=w1154:errorcluster)  [unwired: 1 in, 1 out]
                }
                frame "Spectrometer_Measure" {
                  w1192 = "_"
                  n510 = Unbundle By Name(w1163) -> ("Time Stamp"=w1162:timestamp)
                  n511 = property on="Nr After Spin" class="DigNum (strict)"() -> ("Value"=w1161:u16)  [unwired: 2 in, 2 out]
                  n512 = Unbundle By Name(w1168) -> ("Wavlength"=w1165:dbl[unit][])
                  n513 = property on="Measure_FileName" class="Str"() -> ("Value"=w1191:string)  [unwired: 2 in, 2 out]
                  n514 = Number To Decimal String(number=w1161) -> (decimal integer string=w1159:string)  [unwired: 1 in]
                  n515 = Format Date/Time String(time format string (%c)="%Y%m%d_%H%M%S", seconds (now)=w1162) -> (date/time string=w1193:string)  [unwired: 1 in]
                  n516 = Concatenate Strings(w1193, w1192, w1191, w1192, "a" ("string"), w1159, ".spectra" ("string")) -> (w1190:string)
                  n517 = property on="Measure_SavePath" class="Path"() -> ("Value"=w1189:path)  [unwired: 2 in, 2 out]
                  n518 = Build Path(base path=w1189, name or relative path=w1190) -> (appended path=w1188:path)
                  n519 = Unbundle By Name(w1163) -> ("Data_Raw"=w1183:T11)
                  n520 = Open/Create/Replace File(file path (use dialog)=w1188, error in=w1186, operation (0:open)=T13."open or create") -> (refnum out=w1185:refnum<file>, error out=w1184:errorcluster)  [unwired: 3 in, 1 out]
                  n521 = Index Array(array=w1183, index=0) -> (element=w1181:T14)
                  n522 = Unbundle By Name(w1181) -> ("Image"=w1169:dbl[][][])
                  n523 = Index Array(array=w1169, index (dim 1)=0 ("disabled index (row)")) -> (element=w1175:dbl[][])  [unwired: 2 in]
                  n524 = Transpose 2D Array(2D array=w1175) -> (transposed array=w1172:dbl[][])
                  n525 = To Unsigned Word Integer(number=w1169) -> (unsigned 16bit integer=w1180:u16[][][])
                  n526 = Matrix Size(0:w1172) -> (2:w1173:i32)  [unwired: 1 out]
                  n527 = Write to Binary File(file (use dialog)=w1185, data=w1180, error in=w1184) -> (refnum out=w1178:refnum<file>, error out=w1179:errorcluster)  [unwired: 3 in, 1 out]
                  n528 = Reciprocal(x=w1173) -> (1/x=w1174:dbl)
                  n529 = Close File(refnum=w1178, error in=w1179) -> (error out=w1177:errorcluster)  [unwired: 1 out]
                  n530 = Initialize Array(w1174, w1173) -> (w1171:dbl[])
                  n531 = call-poly <vilib>:"A x B.vi"("Vector"=w1171, "A"=w1172) -> ("A x Vector"=w1164:dbl[])  [unwired: 1 out]
                  n532 = Bundle("Wavlength"=w1165, "A x Vector"=w1164) -> (w1167:T15)  [unwired: 1 in]
                  n533 = Build Array(w1167) -> (w1166:T16)
                  n534 = property on="Measure_Graph" class="XYGraph (strict)"("Value"=w1166) -> ()  [unwired: 2 in, 2 out]
                }
                frame "Stop_Measurement" {
                  n535 = property on="Automatically \nadjust count" class="Bool (strict)"() -> ("Value"=w1196:bool)  [unwired: 2 in, 2 out]
                  n536 = case shown="True" w1196 {
                    frame False {
                    }
                    frame True {
                      n537 = property on="Nr After Spin" class="DigNum (strict)"() -> ("Value"=w1208:u16)  [unwired: 2 in, 2 out]
                      n538 = Increment(x=w1208) -> (x+1=w1207:u16)
                      n539 = property on="Nr After Spin" class="DigNum (strict)"("Value"=w1207) -> ()  [unwired: 2 in, 2 out]
                    }
                  }
                  n540 = Get Queue Status(queue=w1204) -> (queue out=w1205:refnum<queue>, # elements in queue=w1203:i32)  [unwired: 2 in, 6 out]
                  n541 = property on="Measure_MeasureSpectrum" class="Bool (strict)"("Value"=FALSE ("Measure Spectrum")) -> ()  [unwired: 2 in, 2 out]
                  n542 = for {
                    N: w1203 -> [_]
                    shift-right: [w1214] -> w1200
                    shift-left: w1205 -> [w1215]
                    shift-right: [w1211] -> w1199
                    shift-left: w1202 -> [w1212]
                    shift-right: [w1209] -> w1198
                    shift-left: w1201 -> [w1210]
                    n543 = Dequeue Element(queue=w1215) -> (queue out=w1214:refnum<queue>, element=w1213:T6)  [unwired: 2 in, 2 out]
                    n544 = Enqueue Element(queue=w1212, element=w1213, error in (no error)=w1210) -> (queue out=w1211:refnum<queue>, error out=w1209:errorcluster)  [unwired: 1 in, 1 out]
                  }
                }
              }
            }
            n545 = Release Queue(queue=w1132) -> ()  [unwired: 2 in, 3 out]
          }
          frame "Measure_SpectralStability" {
            w1231 = T6 {"QueueAction"=enum."TimeOut", "Data"=[], "Data_Raw"=[], "Data_Dark"=[], "Data_Ref"=[], "Device Information"=[], "Numeric Control"=0.0, "Boolean"=FALSE, "Wavelength"=[], "Time"=[], "Time Stamp"=timestamp(0 s since 1904-01-01), "Numeric Control 2"=0.0, "TabControl"=enum."Measure"}  # DataQueue
            n546 = Unbundle By Name(w1220) -> ("Time Stamp"=w1226:timestamp)
            n547 = Unbundle By Name(w1220) -> ("Numeric Control"=w1216:dbl)
            n548 = property on="SpectralStability\n_SavePath" class="Path"() -> ("Value"=w1222:path)  [unwired: 2 in, 2 out]
            n549 = property on="SpectralStability\n_FileName" class="Str"() -> ("Value"=w1221:string)  [unwired: 2 in, 2 out]
            n550 = Obtain Queue(name (unnamed)="Temp", element data type=w1231) -> (queue out=w1230:refnum<queue>)  [unwired: 3 in, 2 out]
            n551 = call "Num2Str_TrailingZero.vi"("Numeric Control"=w1216) -> ("format string"=w1219:string)  [unwired: 10 in]
            n552 = Format Date/Time String(time format string (%c)="%Y%m%d_%H%M%S", seconds (now)=w1226) -> (date/time string=w1223:string)  [unwired: 1 in]
            n553 = while {
              shift-right: [w1236] -> w1224
              shift-left: w1233 -> [w1236]
              shift-right: [w1242] -> _
              shift-left: w1230 -> [w1244]
              border: 0 -> [_]
              shift-right: [w1243] -> w1217
              shift-left: w1228 -> [w1252]
              shift-right: [w1241] -> w1218
              shift-left: w1227 -> [w1251]
              tunnel: w1223 -> [w1239]
              tunnel: w1222 -> [w1238]
              tunnel: w1221 -> [w1237]
              tunnel: w1219 -> [w1235]
              tunnel: w1216 -> [w1234]
              stop <- w1240 stop-if-true
              n554 = Dequeue Element(queue=w1252, error in (no error)=w1251) -> (queue out=w1250:refnum<queue>, element=w1248:T6, error out=w1249:errorcluster)  [unwired: 1 in, 1 out]
              n555 = Unbundle By Name(w1248) -> ("QueueAction"=w1247:T7)
              n556 = feedback #2() -> (w1245:i32)
              n557 = case shown="\"Spectrometer_Measure\"" w1247 {
                tunnel: w1250 -> [w1256 w1265 w1271 w1289 w1372 w1379]
                tunnel: w1249 -> [w1255 w1262 w1272 w1290 _ w1380]
                tunnel: w1248 -> [w1257 w1261 _ _ w1326 w1411]
                tunnel: [w1259 w1267 w1278 w1296 w1310 w1412] -> w1246
                tunnel: w1245 -> [w1259 w1267 w1278 w1296 w1370 w1412]
                tunnel: w1244 -> [w1258 w1266 w1274 w1292 w1371 w1389]
                tunnel: [w1256 w1264 w1269 w1287 w1372 w1379] -> w1243
                tunnel: [w1254 w1266 w1273 w1291 w1371 w1389] -> w1242
                tunnel: [w1253 w1263 w1270 w1288 w1315 w1380] -> w1241
                tunnel: [_ TRUE TRUE TRUE _ _] -> w1240
                tunnel: w1239 -> [_ _ _ _ w1368 w1409]
                tunnel: w1238 -> [_ _ _ _ w1335 w1377]
                tunnel: w1237 -> [_ _ _ _ w1367 w1407]
                tunnel: w1236 -> [_ _ _ _ w1342 w1406]
                tunnel: w1235 -> [_ _ _ _ w1369 _]
                tunnel: w1234 -> [_ _ _ _ w1311 _]
                frame Default {
                  n558 = Enqueue Element(queue=w1258, element=w1257, error in (no error)=w1255) -> (queue out=w1254:refnum<queue>, error out=w1253:errorcluster)  [unwired: 1 in, 1 out]
                }
                frame "Close_Program" {
                  n559 = Enqueue Element At Opposite End(queue=w1265, element=w1261, error in (no error)=w1262) -> (queue out=w1264:refnum<queue>, error out=w1263:errorcluster)  [unwired: 1 in, 1 out]
                }
                frame "Abort" {
                  n560 = Get Queue Status(queue=w1274) -> (queue out=w1276:refnum<queue>, # elements in queue=w1277:i32)  [unwired: 2 in, 6 out]
                  n561 = for {
                    N: w1277 -> [_]
                    shift-right: [w1284] -> w1273
                    shift-left: w1276 -> [w1285]
                    shift-right: [w1281] -> w1269
                    shift-left: w1271 -> [w1282]
                    shift-right: [w1279] -> w1270
                    shift-left: w1272 -> [w1280]
                    n562 = Dequeue Element(queue=w1285) -> (queue out=w1284:refnum<queue>, element=w1283:T6)  [unwired: 2 in, 2 out]
                    n563 = Enqueue Element(queue=w1282, element=w1283, error in (no error)=w1280) -> (queue out=w1281:refnum<queue>, error out=w1279:errorcluster)  [unwired: 1 in, 1 out]
                  }
                  n564 = property on="SpectralStability_Record" class="Bool (strict)"("Value"=FALSE ("SpectralStability_Record")) -> ()  [unwired: 2 in, 2 out]
                }
                frame "Stop_Measurement" {
                  n565 = Get Queue Status(queue=w1292) -> (queue out=w1294:refnum<queue>, # elements in queue=w1295:i32)  [unwired: 2 in, 6 out]
                  n566 = for {
                    N: w1295 -> [_]
                    shift-right: [w1302] -> w1291
                    shift-left: w1294 -> [w1303]
                    shift-right: [w1299] -> w1287
                    shift-left: w1289 -> [w1300]
                    shift-right: [w1297] -> w1288
                    shift-left: w1290 -> [w1298]
                    n567 = Dequeue Element(queue=w1303) -> (queue out=w1302:refnum<queue>, element=w1301:T6)  [unwired: 2 in, 2 out]
                    n568 = Enqueue Element(queue=w1300, element=w1301, error in (no error)=w1298) -> (queue out=w1299:refnum<queue>, error out=w1297:errorcluster)  [unwired: 1 in, 1 out]
                  }
                  n569 = property on="SpectralStability_Record" class="Bool (strict)"("Value"=FALSE ("SpectralStability_Record")) -> ()  [unwired: 2 in, 2 out]
                }
                frame "Spectrometer_Measure" {
                  w1366 = "_"
                  n570 = Increment(x=w1370) -> (x+1=w1310:i32)
                  n571 = Unbundle By Name(w1326) -> ("Numeric Control 2"=w1325:dbl)
                  n572 = Unbundle By Name(w1326) -> ("Data_Raw"=w1364:T11)
                  n573 = Format Into String(format string=w1369, w1370) -> (resulting string=w1324:string)  [unwired: 2 in, 1 out]
                  n574 = Concatenate Strings(w1368, w1366, w1367, w1366) -> (w1337:string)
                  n575 = Unbundle By Name(w1342) -> ("Wavlength"=w1340:dbl[unit][])
                  n576 = Index Array(array=w1364, index=0) -> (element=w1362:T14)
                  n577 = Divide(x=w1310, y=w1311) -> (x/y=w1314:dbl)
                  n578 = Concatenate Strings(w1337, "s" ("string"), w1324, ".smean" ("string")) -> (w1346:string)
                  n579 = Concatenate Strings(w1337, "raw" ("string"), w1324, ".spectra" ("string")) -> (w1354:string)
                  n580 = Unbundle By Name(w1362) -> ("Image"=w1350:dbl[][][])
                  n581 = Concatenate Strings(w1337, "timing.txt" ("string")) -> (w1334:string)
                  n582 = Subtract(x=w1311, y=w1310) -> (x-y=w1306:dbl)
                  "SS_StepsLeft" <- w1306
                  n583 = Number To Exponential String(number=w1325, 1:FALSE ("use system decimal point (T)")) -> (E-format string=w1322:string)  [unwired: 2 in]
                  n584 = Build Path(base path=w1335, name or relative path=w1346) -> (appended path=w1343:path)
                  n585 = Build Path(base path=w1335, name or relative path=w1334) -> (appended path=w1333:path)
                  n586 = Multiply(x=w1314, y=100.0) -> (x*y=w1313:dbl)
                  n587 = property on="SS:PeriodicTime" class="DigNum (strict)"() -> ("Value"=w1308:dbl[unit])  [unwired: 2 in, 2 out]
                  n588 = Build Path(base path=w1335, name or relative path=w1354) -> (appended path=w1351:path)
                  n589 = Index Array(array=w1350, index (dim 1)=0 ("disabled index (row)")) -> (element=w1361:dbl[][])  [unwired: 2 in]
                  n590 = To Unsigned Byte Integer(number=w1313) -> (unsigned 8bit integer=→"Horizontal Progress Bar":u8)
                  n591 = To Unsigned Word Integer(number=w1350) -> (unsigned 16bit integer=w1349:u16[][][])
                  n592 = Open/Create/Replace File(file path (use dialog)=w1333, operation (0:open)=T13."open or create") -> (refnum out=w1331:refnum<file>, error out=w1328:errorcluster)  [unwired: 4 in, 1 out]
                  n593 = Concatenate Strings(w1324, "\t", w1322, "\r\n") -> (w1321:string)
                  n594 = Transpose 2D Array(2D array=w1361) -> (transposed array=w1358:dbl[][])
                  n595 = Write to Binary File(file (use dialog)=w1351, data=w1349) -> (refnum out=w1347:refnum<file>, error out=w1348:errorcluster)  [unwired: 4 in, 1 out]
                  n596 = Multiply(x=w1308, y=w1306) -> (x*y=→"SS_TimePrediction":dbl[unit])
                  n597 = Set File Position(refnum=w1331, from (0:start)=enum16{"start", "end", "current"}."end", error in=w1328) -> (refnum out=w1329:refnum<file>, error out=w1327:errorcluster)  [unwired: 1 in]
                  n598 = Matrix Size(0:w1358) -> (2:w1359:i32)  [unwired: 1 out]
                  n599 = Close File(refnum=w1347, error in=w1348) -> (error out=w1318:errorcluster)  [unwired: 1 out]
                  n600 = Reciprocal(x=w1359) -> (1/x=w1360:dbl)
                  n601 = Write to Text File(file (use dialog)=w1329, text=w1321, error in=w1327) -> (refnum out=w1320:refnum<file>, error out=w1319:errorcluster)  [unwired: 1 in, 1 out]
                  n602 = Initialize Array(w1360, w1359) -> (w1357:dbl[])
                  n603 = call-poly <vilib>:"A x B.vi"("Vector"=w1357, "A"=w1358) -> ("A x Vector"=w1339:dbl[])  [unwired: 1 out]
                  n604 = Bundle("Wavlength"=w1340, "A x Vector"=w1339) -> (w1341:T15)  [unwired: 1 in]
                  n605 = Close File(refnum=w1320, error in=w1319) -> (error out=w1316:errorcluster)  [unwired: 1 out]
                  n606 = Write to Binary File(file (use dialog)=w1343, data=w1339) -> (refnum out=w1345:refnum<file>, error out=w1344:errorcluster)  [unwired: 4 in, 1 out]
                  n607 = Build Array(w1341) -> (w1338:T16)
                  n608 = Close File(refnum=w1345, error in=w1344) -> (error out=w1317:errorcluster)  [unwired: 1 out]
                  n609 = property on="SpectralStability:\nGraph" class="XYGraph (strict)"("Value"=w1338) -> ()  [unwired: 2 in, 2 out]
                  n610 = Merge Errors(w1318, w1317, w1316) -> (w1315:errorcluster)
                }
                frame "Transfer_Settings" {
                  w1382 = "\r\n"
                  w1396 = 0.0
                  w1402 = 0 ("index")
                  n611 = Unbundle By Name(w1406) -> ("Dark"=w1403:T11, "Ref"=w1404:T11, "Wavlength"=w1405:dbl[unit][])
                  n612 = Concatenate Strings(w1409, "_", w1407) -> (w1395:string)
                  n613 = property on="SpectralStability_\nPeriodicTime" class="DigNum (strict)"() -> ("Value"=w1388:dbl[unit])  [unwired: 2 in, 2 out]
                  n614 = Unbundle By Name(w1411) -> ("Device Information"=w1410:string[])
                  n615 = property on="SpectralStability_Duration" class="DigNum (strict)"() -> ("Value"=w1387:dbl[unit])  [unwired: 2 in, 2 out]
                  n616 = Index Array(array=w1403, index=w1402) -> (element=w1400:T14)
                  n617 = Index Array(array=w1404, index=w1402) -> (element=w1401:T14)
                  n618 = Concatenate Strings(w1395, "_add.spin" ("string")) -> (w1392:string)
                  n619 = Concatenate Strings(w1395, "_comments.txt" ("string")) -> (w1378:string)
                  n620 = Unbundle By Name(w1400) -> ("Image"=w1374:dbl[][][])
                  n621 = Unbundle By Name(w1401) -> ("Image"=w1373:dbl[][][])
                  n622 = property on="SpectralStability_\nMeasurementNumber" class="DigNum (strict)"() -> ("Value"=w1386:u32)  [unwired: 2 in, 2 out]
                  n623 = Build Path(base path=w1377, name or relative path=w1392) -> (appended path=w1391:path)
                  n624 = Build Path(base path=w1377, name or relative path=w1378) -> (appended path=w1376:path)
                  n625 = node(w1405) -> (w1397:dbl[])
                  n626 = property on="Duration/Times" class="Bool (strict)"() -> ("Value"=w1385:bool)  [unwired: 2 in, 2 out]
                  n627 = To Unsigned Word Integer(number=w1374) -> (unsigned 16bit integer=w1399:u16[][][])
                  n628 = To Unsigned Word Integer(number=w1373) -> (unsigned 16bit integer=w1398:u16[][][])
                  n629 = call "DeviceInfo2Str.vi"("Device Information"=w1410) -> ("String"=w1384:string)  [unwired: 10 in]
                  n630 = property on="SpectralStability:\nComments" class="Str"() -> ("Value"=w1381:string)  [unwired: 2 in, 2 out]
                  n631 = Bundle(w1399, w1398, w1397, w1396, w1396) -> (w1390:cluster{u16[][][], u16[][][], dbl[], dbl, dbl})  [unwired: 1 in]
                  n632 = call "String_SpectralStabilitySettings.vi"("Duration/Times"=w1385, "Measurement Number"=w1386, "Duration"=w1387, "Periodic Time"=w1388) -> ("String"=w1383:string)  [unwired: 7 in]
                  n633 = Concatenate Strings(w1384, w1382, w1383, w1382, w1381) -> (w1375:string)
                  n634 = Write to Binary File(file (use dialog)=w1391, data=w1390) -> ()  [unwired: 4 in, 3 out]
                  n635 = Write to Text File(file (use dialog)=w1376, text=w1375) -> ()  [unwired: 2 in, 3 out]
                }
              }
              n636 = feedback-in #2(w1246) -> ()
            }
          }
          frame "Save_InSitu" {
            w1420 = "\r\n"
            n637 = Unbundle By Name(w1458) -> ("Time Stamp"=w1456:timestamp, "Device Information"=w1447:string[], "Numeric Control"=w1444:dbl, "Numeric Control 2"=w1443:dbl)
            n638 = Unbundle By Name(w1445) -> ("Dark"=w1464:T11, "Ref"=w1462:T11, "Wavlength Trim"=w1466:dbl[unit][])
            n639 = property on="LowerWLLimit" class="DigNum (strict)"() -> ("Value"=w1416:i32)  [unwired: 2 in, 2 out]
            n640 = node(w1466) -> (w1459:dbl[])
            n641 = property on="Frames" class="DigNum (strict)"() -> ("Value"=w1431:i32)  [unwired: 2 in, 2 out]
            n642 = call "DeviceInfo2Str.vi"("Device Information"=w1447) -> ("String"=w1446:string)  [unwired: 10 in]
            n643 = Number To Decimal String(number=w1431) -> (decimal integer string=w1430:string)  [unwired: 1 in]
            n644 = property on="Seconds after Spin" class="DigNum (strict)"() -> ("Value"=w1427:dbl[unit])  [unwired: 2 in, 2 out]
            n645 = property on="Seconds to Spin" class="DigNum (strict)"() -> ("Value"=w1428:dbl[unit])  [unwired: 2 in, 2 out]
            n646 = Index Array(array=w1462, index=0) -> (element=w1460:T14)
            n647 = property on="UpperWLLimit" class="DigNum (strict)"() -> ("Value"=w1415:i32)  [unwired: 2 in, 2 out]
            n648 = Index Array(array=w1464, index=0) -> (element=w1461:T14)
            n649 = property on="Measure_FileName" class="Str"() -> ("Value"=w1440:string)  [unwired: 2 in, 2 out]
            n650 = property on="Program Spin Coater" class="Arr (strict)"() -> ("Value"=w1429:T2)  [unwired: 2 in, 2 out]
            n651 = Unbundle By Name(w1461) -> ("Image"=w1417:dbl[][][])
            n652 = Unbundle By Name(w1460) -> ("Image"=w1418:dbl[][][])
            n653 = Format Date/Time String(time format string (%c)="%Y%m%d_%H%M%S", seconds (now)=w1456) -> (date/time string=w1455:string)  [unwired: 1 in]
            n654 = call "MeasurementSpin2String.vi"("Seconds after Spin Stop"=w1427, "Seconds to Spin Start"=w1428, "Program Spin Coater"=w1429) -> ("concatenated string"=w1426:string)
            n655 = property on="Duration after" class="DigNum (strict)"() -> ("Value"=w1423:dbl[unit])  [unwired: 2 in, 2 out]
            n656 = Concatenate Strings(w1455, "_" ("string"), w1440) -> (w1453:string)
            n657 = call "Trim_Spectra.vi"("WL_UpperIndex"=w1415, "WL_LowerIndex"=w1416, "Image"=w1418) -> ("ImageCut"=w1413:dbl[][][])
            n658 = property on="periodic time" class="DigNum (strict)"() -> ("Value"=w1424:dbl[unit])  [unwired: 2 in, 2 out]
            n659 = call "Trim_Spectra.vi"("WL_UpperIndex"=w1415, "WL_LowerIndex"=w1416, "Image"=w1417) -> ("ImageCut"=w1414:dbl[][][])
            n660 = property on="Spin at end" class="Bool (strict)"() -> ("Value"=w1422:bool)  [unwired: 2 in, 2 out]
            n661 = To Unsigned Word Integer(number=w1413) -> (unsigned 16bit integer=w1433:u16[][][])
            n662 = call "AfterSpinOptions.vi"("Spin at end"=w1422, "Duration after"=w1423, "periodic time"=w1424) -> ("concatenated string"=w1425:string)  [unwired: 8 in]
            n663 = To Unsigned Word Integer(number=w1414) -> (unsigned 16bit integer=w1434:u16[][][])
            n664 = Concatenate Strings(w1446, w1420, "Frames:\t" ("string"), w1430, w1420, w1426, w1420, w1425, w1420, "Comments:" ("string"), w1420, "Measure_Comments") -> (w1442:string)
            n665 = Bundle(w1434, w1433, w1459, "Numeric Control"=w1444, "Numeric Control 2"=w1443) -> (w1437:T17)  [unwired: 1 in]
            n666 = property on="Measure_SavePath" class="Path"() -> ("Value"=w1439:path)  [unwired: 2 in, 2 out]
            n667 = Concatenate Strings(w1453, "_add.spin" ("string")) -> (w1451:string)
            n668 = Concatenate Strings(w1453, "_comments.txt" ("string")) -> (w1450:string)
            n669 = Build Path(base path=w1439, name or relative path=w1451) -> (appended path=w1438:path)
            n670 = Build Path(base path=w1439, name or relative path=w1450) -> (appended path=w1449:path)
            n671 = Write to Text File(file (use dialog)=w1449, text=w1442) -> (error out=w1436:errorcluster)  [unwired: 2 in, 2 out]
            n672 = Write to Binary File(file (use dialog)=w1438, data=w1437) -> (error out=w1435:errorcluster)  [unwired: 4 in, 2 out]
            n673 = flat-sequence {
              tunnel: w1436 -> [_]
              tunnel: w1435 -> [_]
              frame #0 {
                n674 = property on="Action" class="Str"("Value"="" ("Action")) -> ()  [unwired: 2 in, 2 out]
              }
            }
            n675 = property on="Action" class="Str"("Value"="Saving" ("Action")) -> ()  [unwired: 2 in, 2 out]
          }
          frame "Set_Dark" {
            # "Averaging"
            n676 = Unbundle By Name(w1481) -> ("Wavlength"=w1480:dbl[unit][])
            n677 = Unbundle By Name(w1488) -> ("Data_Dark"=w1478:T11)
            n678 = Index Array(array=w1478, index=0) -> (element=w1483:T14)
            n679 = Unbundle By Name(w1483) -> ("Image"=w1477:dbl[][][])
            n680 = Index Array(array=w1477, index (dim 1)=0 ("disabled index (row)")) -> (element=w1475:dbl[][])  [unwired: 2 in]
            n681 = Transpose 2D Array(2D array=w1475) -> (transposed array=w1472:dbl[][])
            n682 = Matrix Size(0:w1472) -> (2:w1473:i32)  [unwired: 1 out]
            n683 = Reciprocal(x=w1473) -> (1/x=w1474:dbl)
            n684 = Initialize Array(w1474, w1473) -> (w1471:dbl[])
            n685 = call-poly <vilib>:"A x B.vi"("Vector"=w1471, "A"=w1472) -> ("A x Vector"=w1470:dbl[])  [unwired: 1 out]
            n686 = Bundle("Wavlength"=w1480, "A x Vector"=w1470) -> (w1482:T15)  [unwired: 1 in]
            n687 = Build Array(w1482) -> (w1479:T16)
            n688 = property on="Measure_Graph" class="XYGraph (strict)"("Value"=w1479) -> ()  [unwired: 2 in, 2 out]
            n689 = Bundle By Name(cluster=w1481, "Dark"=w1478) -> (w1485:T4)
          }
          frame "Set_Ref" {
            # "Averaging"
            n690 = Unbundle By Name(w1490) -> ("Wavlength"=w1489:dbl[unit][])
            n691 = Unbundle By Name(w1507) -> ("Data_Ref"=w1494:T11)
            n692 = Index Array(array=w1494, index=0) -> (element=w1502:T14)
            n693 = Unbundle By Name(w1502) -> ("Image"=w1501:dbl[][][])
            n694 = Index Array(array=w1501, index (dim 1)=0 ("disabled index (row)")) -> (element=w1499:dbl[][])  [unwired: 2 in]
            n695 = Transpose 2D Array(2D array=w1499) -> (transposed array=w1496:dbl[][])
            n696 = Matrix Size(0:w1496) -> (2:w1497:i32)  [unwired: 1 out]
            n697 = Reciprocal(x=w1497) -> (1/x=w1498:dbl)
            n698 = Initialize Array(w1498, w1497) -> (w1495:dbl[])
            n699 = call-poly <vilib>:"A x B.vi"("Vector"=w1495, "A"=w1496) -> ("A x Vector"=w1491:dbl[])  [unwired: 1 out]
            n700 = Bundle("Wavlength"=w1489, "A x Vector"=w1491) -> (w1493:T15)  [unwired: 1 in]
            n701 = Build Array(w1493) -> (w1492:T16)
            n702 = Bundle By Name(cluster=w1490, "Ref"=w1494) -> (w1504:T4)
            n703 = property on="Measure_Graph" class="XYGraph (strict)"("Value"=w1492) -> ()  [unwired: 2 in, 2 out]
          }
          frame "Set_Wavelength" {
            n704 = Unbundle By Name(w1511) -> ("Wavelength"=w1514:dbl[unit][])
            n705 = Bundle By Name(cluster=w1513, "Wavlength"=w1514) -> (w1512:T4)
            n706 = property on="Trim\nSpec" class="Bool (strict)"() -> ("Value"=w1508:bool)  [unwired: 2 in, 2 out]
            n707 = property on="Trim\nSpec" class="Bool (strict)"("Val(Sgnl)"=w1508) -> ()  [unwired: 2 in, 2 out]
          }
          frame "Spectrometer_Preview" {
            w1521 = 0 ("index (page)")
            n708 = Unbundle By Name(w1517) -> ("Data_Raw"=w1525:T11)
            n709 = Unbundle By Name(w1526) -> ("Wavlength"=w1520:dbl[unit][])
            n710 = Unbundle By Name(w1517) -> ("TabControl"=w1516:T8)
            n711 = Index Array(array=w1525, index=0) -> (element=w1523:T14)
            n712 = Unbundle By Name(w1523) -> ("Image"=w1522:dbl[][][])
            n713 = Index Array(array=w1522, index (dim 0)=w1521, index (dim 1)=w1521) -> (element=w1519:dbl[])  [unwired: 1 in]
            n714 = Bundle("Wavlength"=w1520, "Image"=w1519) -> (w1518:cluster{"Wavlength":dbl[unit][], "Image":dbl[]})  [unwired: 1 in]
            n715 = Build Array(w1518) -> (w1515:T3)
            n716 = case shown="Default" w1516 {
              tunnel: w1515 -> [w1529 w1530 _]
              frame "Measure" {
                "Measure_Graph" <- w1529
              }
              frame "Spectral Stability" {
                "SpectralStability_Graph" <- w1530
              }
              frame Default {
              }
            }
          }
          frame "Change_TrimSettings" {
            n717 = Unbundle By Name(w1538) -> ("Boolean"=w1537:bool)
            n718 = case shown="True" w1537 {
              tunnel: w1533 -> [w1544 w1562]
              tunnel: w1538 -> [_ w1557]
              tunnel: [0 w1548] -> w1535
              tunnel: [w1542 w1549] -> w1534
              tunnel: [w1540 w1545] -> w1531
              frame False {
                n719 = Unbundle By Name(w1544) -> ("Wavlength"=w1540:dbl[unit][])
                n720 = Array Size(array=w1540) -> (size(s)=w1543:i32)
                n721 = Decrement(x=w1543) -> (x-1=w1542:i32)
              }
              frame True {
                n722 = Unbundle By Name(w1557) -> ("Numeric Control"=w1561:dbl, "Numeric Control 2"=w1555:dbl)
                n723 = Unbundle By Name(w1562) -> ("Wavlength"=w1550:dbl[unit][])
                n724 = node(w1561) -> (w1560:dbl[unit])
                n725 = node(w1555) -> (w1554:dbl[unit])
                n726 = Subtract(x=w1550, y=w1554) -> (x-y=w1553:dbl[unit][])
                n727 = Subtract(x=w1550, y=w1560) -> (x-y=w1559:dbl[unit][])
                n728 = Absolute Value(x=w1553) -> (abs(x)=w1552:dbl[unit][])
                n729 = Absolute Value(x=w1559) -> (abs(x)=w1558:dbl[unit][])
                n730 = Array Max & Min(array=w1552) -> (min index (indices)=w1549:i32)  [unwired: 3 out]
                n731 = Array Max & Min(array=w1558) -> (min index (indices)=w1548:i32)  [unwired: 3 out]
                n732 = Subtract(x=w1549, y=w1548) -> (x-y=w1547:i32)
                n733 = Index Array(array=w1550, index=w1549) -> (element=w1551:dbl[unit])
                n734 = Index Array(array=w1550, index=w1548) -> (element=w1556:dbl[unit])
                n735 = Increment(x=w1547) -> (x+1=w1546:i32)
                n736 = Array Subset(array=w1550, index=w1548, length=w1546) -> (w1545:dbl[unit][])
                n737 = property on="Wl \nLow" class="DigNum (strict)"("Value"=w1556) -> ()  [unwired: 2 in, 2 out]
                n738 = property on="Wl \nUp" class="DigNum (strict)"("Value"=w1551) -> ()  [unwired: 2 in, 2 out]
              }
            }
            "LowerWLLimit" <- w1535
            "UpperWLLimit" <- w1534
            n739 = Bundle By Name(cluster=w1533, "Wavlength Trim"=w1531) -> (w1532:T4)
          }
        }
      }
      frame Error {
        w1568 = T12 4 items=["no dialog", "OK message", "continue or stop message", "OK message + warnings", "continue/stop + warnings"] ("type of dialog (OK msg:1)")
        n740 = call <vilib>:"General Error Handler.vi"("type of dialog (OK msg:1)"=w1568, "error in (no error)"=w1565) -> ("error out"=w1567:errorcluster)  [unwired: 9 in, 4 out]
        n741 = call <vilib>:"Clear Errors.vi"("error in (no error)"=w1567) -> ("error out"=w1564:errorcluster)  [unwired: 5 in, 1 out]
      }
    }
  }
  n742 = while {
    shift-right: [w1571] -> _
    shift-left: w12 -> [w1569]
    shift-right: [w1574] -> _
    shift-left: w7 -> [w1575]
    shift-right: [w1572] -> _
    shift-left: w8 -> [w1573]
    stop <- w1570 stop-if-true
    # "Producer"
    n743 = event shown="[5] \"Program Spin Coater\": Value Change" {
      selector: _ -> [_ _ _ _ _ _ _ _ _ _ _ _ _ _ _ _ _ _ _ _ _ _ _ _ _ _ _ _ _ _]
      dyn-events: _ -> [_ _ _ _ _ _ _ _ _ _ _ _ _ _ _ _ _ _ _ _ _ _ _ _ _ _ _ _ _ _]
      timeout: -1 -> [_ _ _ _ _ _ _ _ _ _ _ _ _ _ _ _ _ _ _ _ _ _ _ _ _ _ _ _ _ _]
      tunnel: w1575 -> [w1578 w1593 w1601 w1614 w1629 w1644 w1649 w1664 w1668 w1677 w1689 w1704 w1728 w1731 w1738 w1784 w1789 w1828 w1833 w1853 w1862 w1871 w1879 w1885 w1899 w1926 w1943 w1949 w1964 w2005]
      tunnel: [w1578 w1590 w1600 w1614 w1629 w1644 w1649 w1664 w1668 w1677 w1689 w1704 w1728 w1731 w1738 w1784 w1789 w1828 w1832 w1853 w1862 w1871 w1879 w1885 w1897 w1924 w1943 w1949 w1964 w2004] -> w1574
      tunnel: w1573 -> [w1577 w1592 w1604 w1612 w1626 w1643 w1648 w1661 w1669 w1678 w1690 w1702 w1723 w1730 w1735 w1769 w1788 w1819 w1839 w1852 w1861 w1870 w1878 w1884 w1902 w1930 w1944 w1948 w1962 w1997]
      tunnel: [w1577 w1586 w1595 w1608 w1625 w1641 w1648 w1660 w1670 w1679 w1691 w1700 w1722 w1730 w1733 w1763 w1786 w1802 w1831 w1847 w1858 w1867 w1878 w1884 w1902 w1930 w1944 w1948 w1959 w1997] -> w1572
      tunnel: w1569 -> [w1579 w1594 w1605 w1613 w1628 w1645 w1650 w1663 w1672 w1681 w1693 w1703 w1725 w1732 w1736 w1770 w1790 w1820 w1841 w1854 w1863 w1872 w1880 w1886 w1895 w1931 w1942 w1950 w1963 w2008]
      tunnel: [w1579 w1591 w1603 w1609 w1627 w1642 w1650 w1662 w1671 w1680 w1692 w1701 w1724 w1732 w1737 w1762 w1787 w1801 w1840 w1848 w1859 w1868 w1880 w1883 w1890 w1929 w1942 w1950 w1960 w2008] -> w1571
      tunnel: [_ TRUE _ _ _ _ _ _ _ _ _ _ _ _ _ _ _ _ _ _ _ _ _ _ _ _ _ _ _ _] -> w1570
      event Timeout {
        n744 = event-data() -> ()  [unwired: 1 in, 3 out]
      }
      event "Stop Button": Value Change {
        w1582 = T6 {"QueueAction"=enum."TimeOut", "Data"=[], "Data_Raw"=[], "Data_Dark"=[], "Data_Ref"=[], "Device Information"=[], "Numeric Control"=0.0, "Boolean"=FALSE, "Wavelength"=[], "Time"=[], "Time Stamp"=timestamp(0 s since 1904-01-01), "Numeric Control 2"=0.0, "TabControl"=enum."Measure"}  # DataQueue
        w1585 = T9 {"QueueAction"=enum."TimeOut", "Numeric 1"=0.0, "Numeric 2"=0.0, "Boolean 1"=FALSE, "Boolean 2"=FALSE, "Spin Program"=[], "Spin Prg v07"=[], "Time Stamp"=timestamp(0 s since 1904-01-01), "TabControl"=enum."Measure"}  # Device Queue
        n745 = event-data() -> ()  [unwired: 1 in, 6 out]
        n746 = Bundle By Name(cluster=w1585, "QueueAction"=DeviceQueue_Action."Close_Program") -> (w1583:T9)
        n747 = Enqueue Element At Opposite End(queue=w1594, element=w1583, error in (no error)=w1592) -> (queue out=w1591:refnum<queue>, error out=w1587:errorcluster)  [unwired: 1 in, 1 out]
        n748 = Bundle By Name(cluster=w1582, "QueueAction"=DataQueue_Action."Close_Program") -> (w1580:T6)
        n749 = Enqueue Element At Opposite End(queue=w1593, element=w1580, error in (no error)=w1592) -> (queue out=w1590:refnum<queue>, error out=w1588:errorcluster)  [unwired: 1 in, 1 out]
        n750 = Merge Errors(w1588, w1587) -> (w1586:errorcluster)
      }
      event "Abort Button": Value Change {
        w1599 = T6 {"QueueAction"=enum."TimeOut", "Data"=[], "Data_Raw"=[], "Data_Dark"=[], "Data_Ref"=[], "Device Information"=[], "Numeric Control"=0.0, "Boolean"=FALSE, "Wavelength"=[], "Time"=[], "Time Stamp"=timestamp(0 s since 1904-01-01), "Numeric Control 2"=0.0, "TabControl"=enum."Measure"}  # DataQueue
        w1607 = T9 {"QueueAction"=enum."TimeOut", "Numeric 1"=0.0, "Numeric 2"=0.0, "Boolean 1"=FALSE, "Boolean 2"=FALSE, "Spin Program"=[], "Spin Prg v07"=[], "Time Stamp"=timestamp(0 s since 1904-01-01), "TabControl"=enum."Measure"}  # Device Queue
        n751 = event-data() -> ()  [unwired: 1 in, 6 out]
        n752 = Bundle By Name(cluster=w1607, "QueueAction"=DeviceQueue_Action."Abort") -> (w1606:T9)
        n753 = Bundle By Name(cluster=w1599, "QueueAction"=DataQueue_Action."Abort") -> (w1597:T6)
        n754 = Enqueue Element At Opposite End(queue=w1605, element=w1606, error in (no error)=w1604) -> (queue out=w1603:refnum<queue>, error out=w1596:errorcluster)  [unwired: 1 in, 1 out]
        n755 = Enqueue Element At Opposite End(queue=w1601, element=w1597, error in (no error)=w1596) -> (queue out=w1600:refnum<queue>, error out=w1595:errorcluster)  [unwired: 1 in, 1 out]
      }
      event "Init_Spectrometer": Value Change {
        n756 = event-data() -> ()  [unwired: 1 in, 6 out]
        n757 = case shown="False" "Init_Spectrometer" {
          tunnel: [w1616 w1619] -> w1610
          frame True {
            n758 = property on="Tab Control" class="TabCtl (strict)"() -> ("Value"=w1615:T1)  [unwired: 2 in, 2 out]
            n759 = Bundle By Name(cluster=T9 {"QueueAction"=enum."TimeOut", "Numeric 1"=0.0, "Numeric 2"=0.0, "Boolean 1"=FALSE, "Boolean 2"=FALSE, "Spin Program"=[], "Spin Prg v07"=[], "Time Stamp"=timestamp(0 s since 1904-01-01), "TabControl"=enum."Measure"} ("element"), "QueueAction"=DeviceQueue_Action."Spectrometer_Init", "TabControl"=w1615) -> (w1616:T9)
          }
          frame False {
            n760 = Bundle By Name(cluster=T9 {"QueueAction"=enum."TimeOut", "Numeric 1"=0.0, "Numeric 2"=0.0, "Boolean 1"=FALSE, "Boolean 2"=FALSE, "Spin Program"=[], "Spin Prg v07"=[], "Time Stamp"=timestamp(0 s since 1904-01-01), "TabControl"=enum."Measure"} ("element"), "QueueAction"=DeviceQueue_Action."Spectrometer_Close") -> (w1619:T9)
          }
        }
        n761 = Enqueue Element(queue=w1613, element=w1610, error in (no error)=w1612) -> (queue out=w1609:refnum<queue>, error out=w1608:errorcluster)  [unwired: 1 in, 1 out]
      }
      event "Init_Arduino": Value Change {
        # "Shutter is closed after init"
        n762 = event-data() -> ("NewVal"=w1624:bool)  [unwired: 1 in, 5 out]
        n763 = case shown="True" w1624 {
          tunnel: [w1630 w1633] -> w1623
          frame False {
            w1632 = T9 {"QueueAction"=enum."TimeOut", "Numeric 1"=0.0, "Numeric 2"=0.0, "Boolean 1"=FALSE, "Boolean 2"=FALSE, "Spin Program"=[], "Spin Prg v07"=[], "Time Stamp"=timestamp(0 s since 1904-01-01), "TabControl"=enum."Measure"}  # Device Queue
            n764 = Bundle By Name(cluster=w1632, "QueueAction"=DeviceQueue_Action."Arduino_Close") -> (w1630:T9)
          }
          frame True {
            w1635 = T9 {"QueueAction"=enum."TimeOut", "Numeric 1"=0.0, "Numeric 2"=0.0, "Boolean 1"=FALSE, "Boolean 2"=FALSE, "Spin Program"=[], "Spin Prg v07"=[], "Time Stamp"=timestamp(0 s since 1904-01-01), "TabControl"=enum."Measure"}  # Device Queue
            n765 = Bundle By Name(cluster=w1635, "QueueAction"=DeviceQueue_Action."Arduino_Init") -> (w1633:T9)
          }
        }
        n766 = property on="Shutter Toggle" class="Bool (strict)"("Value"=FALSE ("Shutter Toggle")) -> ()  [unwired: 2 in, 2 out]
        n767 = Enqueue Element(queue=w1628, element=w1623, error in (no error)=w1626) -> (queue out=w1627:refnum<queue>, error out=w1625:errorcluster)  [unwired: 1 in, 1 out]
      }
      event "Program Spin Coater": Value Change {
        w1647 = T9 {"QueueAction"=enum."TimeOut", "Numeric 1"=0.0, "Numeric 2"=0.0, "Boolean 1"=FALSE, "Boolean 2"=FALSE, "Spin Program"=[], "Spin Prg v07"=[], "Time Stamp"=timestamp(0 s since 1904-01-01), "TabControl"=enum."Measure"}  # Device Queue
        n768 = event-data() -> ("NewVal"=w1636:T2)  [unwired: 1 in, 5 out]
        n769 = property on="Seconds to Spin" class="DigNum (strict)"() -> ("Value"=w1638:dbl[unit])  [unwired: 2 in, 2 out]
        n770 = node(w1638) -> (w1637:dbl)
        n771 = Bundle By Name(cluster=w1647, "QueueAction"=DeviceQueue_Action."Arduino_LoadProgram", "Spin Prg v07"=w1636, "Numeric 1"=w1637) -> (w1646:T9)
        n772 = Enqueue Element(queue=w1645, element=w1646, error in (no error)=w1643) -> (queue out=w1642:refnum<queue>, error out=w1641:errorcluster)  [unwired: 1 in, 1 out]
        n773 = property on="Measure_IntegrationTime" class="DigNum (strict)"() -> ("Value"=w1639:dbl[unit])  [unwired: 2 in, 2 out]
        n774 = property on="Measure_IntegrationTime" class="DigNum (strict)"("Val(Sgnl)"=w1639) -> ()  [unwired: 2 in, 2 out]
      }
      event "SHUTTER DEBUG": Value Change {
        n775 = event-data() -> ("NewVal"=w1652:bool)  [unwired: 1 in, 5 out]
        n776 = Select(t=u8 0, s=w1652, f=u8 2) -> (s? t:f=w1651:u8)
        n777 = property on="Shutter Position" class="DigNum (strict)"("DisabledEnum"=w1651) -> ()  [unwired: 2 in, 2 out]
        n778 = property on="Shutter Close" class="Bool (strict)"("DisabledEnum"=w1651) -> ()  [unwired: 2 in, 2 out]
        n779 = property on="Shutter Open" class="Bool (strict)"("DisabledEnum"=w1651) -> ()  [unwired: 2 in, 2 out]
      }
      event "Shutter Position": Value Change {
        w1659 = FALSE ("Shutter Close")
        w1657 = T9 {"QueueAction"=enum."TimeOut", "Numeric 1"=0.0, "Numeric 2"=0.0, "Boolean 1"=FALSE, "Boolean 2"=FALSE, "Spin Program"=[], "Spin Prg v07"=[], "Time Stamp"=timestamp(0 s since 1904-01-01), "TabControl"=enum."Measure"}  # Device Queue
        (unwired) DeviceQueue_Action."Arduino_SetSpeed" ("QueueAction")
        (unwired) T9 {"QueueAction"=enum."TimeOut", "Numeric 1"=0.0, "Numeric 2"=0.0, "Boolean 1"=FALSE, "Boolean 2"=FALSE, "Spin Program"=[], "Spin Prg v07"=[], "Time Stamp"=timestamp(0 s since 1904-01-01), "TabControl"=enum."Measure"}  # Device Queue
        n780 = event-data() -> ("NewVal"=w1655:u16)  [unwired: 1 in, 5 out]
        n781 = property on="Shutter Close" class="Bool (strict)"("Value"=w1659) -> ()  [unwired: 2 in, 2 out]
        n782 = property on="Shutter Open" class="Bool (strict)"("Value"=w1659) -> ()  [unwired: 2 in, 2 out]
        n783 = Bundle By Name(cluster=w1657, "QueueAction"=DeviceQueue_Action."Arduino_Shutter_SetPosition", "Numeric 1"=w1655) -> (w1658:T9)
        n784 = Enqueue Element(queue=w1663, element=w1658, error in (no error)=w1661) -> (queue out=w1662:refnum<queue>, error out=w1660:errorcluster)  [unwired: 1 in, 1 out]
      }
      event "Shutter Close": Value Change {
        w1667 = T9 {"QueueAction"=enum."TimeOut", "Numeric 1"=0.0, "Numeric 2"=0.0, "Boolean 1"=FALSE, "Boolean 2"=FALSE, "Spin Program"=[], "Spin Prg v07"=[], "Time Stamp"=timestamp(0 s since 1904-01-01), "TabControl"=enum."Measure"}  # Device Queue
        (unwired) DeviceQueue_Action."Arduino_SetSpeed" ("QueueAction")
        (unwired) T9 {"QueueAction"=enum."TimeOut", "Numeric 1"=0.0, "Numeric 2"=0.0, "Boolean 1"=FALSE, "Boolean 2"=FALSE, "Spin Program"=[], "Spin Prg v07"=[], "Time Stamp"=timestamp(0 s since 1904-01-01), "TabControl"=enum."Measure"}  # Device Queue
        n785 = event-data() -> ()  [unwired: 1 in, 6 out]
        n786 = property on="Shutter Open" class="Bool (strict)"("Value"=FALSE ("Shutter Open")) -> ()  [unwired: 2 in, 2 out]
        n787 = Bundle By Name(cluster=w1667, "QueueAction"=DeviceQueue_Action."Arduino_Shutter_Close") -> (w1666:T9)
        n788 = Enqueue Element(queue=w1672, element=w1666, error in (no error)=w1669) -> (queue out=w1671:refnum<queue>, error out=w1670:errorcluster)  [unwired: 1 in, 1 out]
      }
      event "Shutter Open": Value Change {
        w1676 = T9 {"QueueAction"=enum."TimeOut", "Numeric 1"=0.0, "Numeric 2"=0.0, "Boolean 1"=FALSE, "Boolean 2"=FALSE, "Spin Program"=[], "Spin Prg v07"=[], "Time Stamp"=timestamp(0 s since 1904-01-01), "TabControl"=enum."Measure"}  # Device Queue
        (unwired) DeviceQueue_Action."Arduino_SetSpeed" ("QueueAction")
        (unwired) T9 {"QueueAction"=enum."TimeOut", "Numeric 1"=0.0, "Numeric 2"=0.0, "Boolean 1"=FALSE, "Boolean 2"=FALSE, "Spin Program"=[], "Spin Prg v07"=[], "Time Stamp"=timestamp(0 s since 1904-01-01), "TabControl"=enum."Measure"}  # Device Queue
        n789 = event-data() -> ()  [unwired: 1 in, 6 out]
        n790 = property on="Shutter Close" class="Bool (strict)"("Value"=FALSE ("Shutter Open")) -> ()  [unwired: 2 in, 2 out]
        n791 = Bundle By Name(cluster=w1676, "QueueAction"=DeviceQueue_Action."Arduino_Shutter_Open") -> (w1675:T9)
        n792 = Enqueue Element(queue=w1681, element=w1675, error in (no error)=w1678) -> (queue out=w1680:refnum<queue>, error out=w1679:errorcluster)  [unwired: 1 in, 1 out]
      }
      event "Shutter Toggle": Value Change {
        w1688 = T9 {"QueueAction"=enum."TimeOut", "Numeric 1"=0.0, "Numeric 2"=0.0, "Boolean 1"=FALSE, "Boolean 2"=FALSE, "Spin Program"=[], "Spin Prg v07"=[], "Time Stamp"=timestamp(0 s since 1904-01-01), "TabControl"=enum."Measure"}  # Device Queue
        (unwired) T9 {"QueueAction"=enum."TimeOut", "Numeric 1"=0.0, "Numeric 2"=0.0, "Boolean 1"=FALSE, "Boolean 2"=FALSE, "Spin Program"=[], "Spin Prg v07"=[], "Time Stamp"=timestamp(0 s since 1904-01-01), "TabControl"=enum."Measure"}  # Device Queue
        n793 = event-data() -> ("NewVal"=w1686:bool)  [unwired: 1 in, 5 out]
        n794 = Select(t=DeviceQueue_Action."Arduino_Shutter_Open" ("QueueAction"), s=w1686, f=DeviceQueue_Action."Arduino_Shutter_Close" ("QueueAction")) -> (s? t:f=w1683:T10)
        n795 = Bundle By Name(cluster=w1688, "QueueAction"=w1683) -> (w1687:T9)
        n796 = Enqueue Element(queue=w1693, element=w1687, error in (no error)=w1690) -> (queue out=w1692:refnum<queue>, error out=w1691:errorcluster)  [unwired: 1 in, 1 out]
      }
      event "Measure_IntegrationTime", "SpectralStability_IntegrationTime": Value Change {
        w1706 = T9 {"QueueAction"=enum."TimeOut", "Numeric 1"=0.0, "Numeric 2"=0.0, "Boolean 1"=FALSE, "Boolean 2"=FALSE, "Spin Program"=[], "Spin Prg v07"=[], "Time Stamp"=timestamp(0 s since 1904-01-01), "TabControl"=enum."Measure"}  # Device Queue
        n797 = event-data() -> ("NewVal"=w1698:dbl[unit])  [unwired: 1 in, 5 out]
        n798 = property on="Calculate Frames" class="Bool (strict)"() -> ("Value"=w1694:bool)  [unwired: 2 in, 2 out]
        n799 = node(w1698) -> (w1697:dbl)
        n800 = property on="Tab Control" class="TabCtl (strict)"() -> ("Value"=w1696:T1)  [unwired: 2 in, 2 out]
        n801 = property on="Tab Control" class="TabCtl (strict)"() -> ("Value"=w1695:T1)  [unwired: 2 in, 2 out]
        n802 = case shown="\"Measure\"" w1696 {
          tunnel: w1706 -> [w1707 w1713 w1719]
          tunnel: [w1707 w1710 w1716] -> w1705
          tunnel: DeviceQueue_Action."Spectrometer_SetIntegrationTime" ("QueueAction") -> [_ w1712 w1718]
          tunnel: w1697 -> [_ w1711 w1717]
          tunnel: w1695 -> [_ w1709 w1714]
          tunnel: w1694 -> [_ w1708 _]
          frame Default {
          }
          frame "Measure" {
            n803 = Bundle By Name(cluster=w1713, "QueueAction"=w1712, "Numeric 1"=w1711, "Boolean 1"=w1708, "TabControl"=w1709) -> (w1710:T9)
          }
          frame "Spectral Stability" {
            n804 = Bundle By Name(cluster=w1719, "QueueAction"=w1718, "Numeric 1"=w1717, "Boolean 1"=FALSE, "TabControl"=w1714) -> (w1716:T9)
          }
        }
        n805 = Enqueue Element(queue=w1703, element=w1705, error in (no error)=w1702) -> (queue out=w1701:refnum<queue>, error out=w1700:errorcluster)  [unwired: 1 in, 1 out]
      }
      event "Frames": Value Change {
        w1727 = T9 {"QueueAction"=enum."TimeOut", "Numeric 1"=0.0, "Numeric 2"=0.0, "Boolean 1"=FALSE, "Boolean 2"=FALSE, "Spin Program"=[], "Spin Prg v07"=[], "Time Stamp"=timestamp(0 s since 1904-01-01), "TabControl"=enum."Measure"}  # Device Queue
        n806 = event-data() -> ()  [unwired: 1 in, 6 out]
        n807 = Bundle By Name(cluster=w1727, "QueueAction"=DeviceQueue_Action."Spectrometer_SetFrames", "Numeric 1"="Frames") -> (w1726:T9)
        n808 = Enqueue Element(queue=w1725, element=w1726, error in (no error)=w1723) -> (queue out=w1724:refnum<queue>, error out=w1722:errorcluster)  [unwired: 1 in, 1 out]
      }
      event "Seconds to Spin", "Seconds after Spin": Value Change {
        n809 = event-data() -> ()  [unwired: 1 in, 6 out]
        n810 = property on="Program Spin Coater" class="Arr (strict)"() -> ("Value"=w1729:T2)  [unwired: 2 in, 2 out]
        n811 = property on="Program Spin Coater" class="Arr (strict)"("Val(Sgnl)"=w1729) -> ()  [unwired: 2 in, 2 out]
      }
      event "Calculate Frames": Value Change {
        n812 = event-data() -> ("NewVal"=w1739:bool)  [unwired: 1 in, 5 out]
        n813 = case shown="False" w1739 {
          tunnel: [0 2] -> w1734
          tunnel: w1736 -> [w1741 w1750]
          tunnel: [w1741 w1748] -> w1737
          tunnel: w1735 -> [w1740 w1747]
          tunnel: [w1740 w1743] -> w1733
          frame False {
          }
          frame True {
            w1749 = T9 {"QueueAction"=enum."TimeOut", "Numeric 1"=0.0, "Numeric 2"=0.0, "Boolean 1"=FALSE, "Boolean 2"=FALSE, "Spin Program"=[], "Spin Prg v07"=[], "Time Stamp"=timestamp(0 s since 1904-01-01), "TabControl"=enum."Measure"}  # Device Queue
            n814 = property on="Measure_IntegrationTime" class="DigNum (strict)"() -> ("Value"=w1745:dbl[unit])  [unwired: 2 in, 2 out]
            n815 = node(w1745) -> (w1744:dbl)
            n816 = Bundle By Name(cluster=w1749, "QueueAction"=DeviceQueue_Action."Spectrometer_SetIntegrationTime", "Numeric 1"=w1744) -> (w1751:T9)
            n817 = Enqueue Element(queue=w1750, element=w1751, error in (no error)=w1747) -> (queue out=w1748:refnum<queue>, error out=w1743:errorcluster)  [unwired: 1 in, 1 out]
          }
        }
        n818 = property on="Frames" class="DigNum (strict)"("DisabledEnum"=w1734) -> ()  [unwired: 2 in, 2 out]
      }
      event "Record RefSpec": Value Change {
        w1780 = T9 {"QueueAction"=enum."TimeOut", "Numeric 1"=0.0, "Numeric 2"=0.0, "Boolean 1"=FALSE, "Boolean 2"=FALSE, "Spin Program"=[], "Spin Prg v07"=[], "Time Stamp"=timestamp(0 s since 1904-01-01), "TabControl"=enum."Measure"}  # Device Queue
        n819 = event-data() -> ()  [unwired: 1 in, 6 out]
        n820 = property on="Shutter Toggle" class="Bool (strict)"("Value"=FALSE ("Shutter Toggle")) -> ()  [unwired: 2 in, 2 out]
        n821 = property on="Frames for Ref/Dark" class="DigNum (strict)"() -> ("Value"=w1759:dbl)  [unwired: 2 in, 2 out]
        n822 = property on="Measure_FramesSpectrometer" class="DigNum (strict)"() -> ("Value"=w1754:dbl)  [unwired: 2 in, 2 out]
        n823 = Bundle By Name(cluster=w1780, "QueueAction"=DeviceQueue_Action."Arduino_Shutter_Open") -> (w1777:T9)
        n824 = Bundle By Name(cluster=w1777, "QueueAction"=DeviceQueue_Action."Wait", "Numeric 1"=0.5) -> (w1760:T9)
        n825 = Bundle By Name(cluster=w1760, "QueueAction"=DeviceQueue_Action."Spectrometer_SetFrames", "Numeric 1"=w1759) -> (w1758:T9)
        n826 = Enqueue Element(queue=w1770, element=w1777, error in (no error)=w1769) -> (queue out=w1776:refnum<queue>, error out=w1773:errorcluster)  [unwired: 1 in, 1 out]
        n827 = Bundle By Name(cluster=w1758, "QueueAction"=DeviceQueue_Action."Spectrometer_SetReference") -> (w1757:T9)
        n828 = Enqueue Element(queue=w1776, element=w1760, error in (no error)=w1773) -> (queue out=w1775:refnum<queue>, error out=w1772:errorcluster)  [unwired: 1 in, 1 out]
        n829 = Bundle By Name(cluster=w1757, "QueueAction"=DeviceQueue_Action."Arduino_Shutter_Close") -> (w1755:T9)
        n830 = Enqueue Element(queue=w1775, element=w1758, error in (no error)=w1772) -> (queue out=w1774:refnum<queue>, error out=w1771:errorcluster)  [unwired: 1 in, 1 out]
        n831 = Bundle By Name(cluster=w1755, "QueueAction"=DeviceQueue_Action."Spectrometer_SetFrames", "Numeric 1"=w1754) -> (w1753:T9)
        n832 = Enqueue Element(queue=w1774, element=w1757, error in (no error)=w1771) -> (queue out=w1766:refnum<queue>, error out=w1767:errorcluster)  [unwired: 1 in, 1 out]
        n833 = Enqueue Element(queue=w1766, element=w1755, error in (no error)=w1767) -> (queue out=w1764:refnum<queue>, error out=w1765:errorcluster)  [unwired: 1 in, 1 out]
        n834 = Enqueue Element(queue=w1764, element=w1753, error in (no error)=w1765) -> (queue out=w1762:refnum<queue>, error out=w1763:errorcluster)  [unwired: 1 in, 1 out]
      }
      event "Measure_Preview", "SpectralStability_Preview": Value Change {
        n835 = event-data() -> ("NewVal"=w1785:bool)  [unwired: 1 in, 5 out]
        n836 = case shown="False" w1785 {
          tunnel: w1790 -> [w1792 w1797]
          tunnel: w1788 -> [w1791 w1796]
          tunnel: [w1792 w1795] -> w1787
          tunnel: [w1791 w1794] -> w1786
          frame False {
          }
          frame True {
            w1800 = T9 {"QueueAction"=enum."TimeOut", "Numeric 1"=0.0, "Numeric 2"=0.0, "Boolean 1"=FALSE, "Boolean 2"=FALSE, "Spin Program"=[], "Spin Prg v07"=[], "Time Stamp"=timestamp(0 s since 1904-01-01), "TabControl"=enum."Measure"}  # Device Queue
            n837 = property on="Tab Control" class="TabCtl (strict)"() -> ("Value"=w1793:T1)  [unwired: 2 in, 2 out]
            n838 = Bundle By Name(cluster=w1800, "QueueAction"=DeviceQueue_Action."Spectrometer_Preview", "TabControl"=w1793) -> (w1799:T9)
            n839 = Enqueue Element(queue=w1797, element=w1799, error in (no error)=w1796) -> (queue out=w1795:refnum<queue>, error out=w1794:errorcluster)  [unwired: 1 in, 1 out]
          }
        }
      }
      event "Measure:\nRecord_Darkspec", "SpectralStability:\nRecord_Darkspec": Value Change {
        w1826 = T9 {"QueueAction"=enum."TimeOut", "Numeric 1"=0.0, "Numeric 2"=0.0, "Boolean 1"=FALSE, "Boolean 2"=FALSE, "Spin Program"=[], "Spin Prg v07"=[], "Time Stamp"=timestamp(0 s since 1904-01-01), "TabControl"=enum."Measure"}  # Device Queue
        n840 = event-data() -> ()  [unwired: 1 in, 6 out]
        n841 = property on="Shutter Toggle" class="Bool (strict)"("Value"=FALSE ("Shutter Toggle")) -> ()  [unwired: 2 in, 2 out]
        n842 = property on="Frames for Ref/Dark" class="DigNum (strict)"() -> ("Value"=w1809:dbl)  [unwired: 2 in, 2 out]
        n843 = property on="Measure_FramesSpectrometer" class="DigNum (strict)"() -> ("Value"=w1803:dbl)  [unwired: 2 in, 2 out]
        n844 = Bundle By Name(cluster=w1826, "QueueAction"=DeviceQueue_Action."Arduino_Shutter_Close") -> (w1825:T9)
        n845 = Bundle By Name(cluster=w1825, "QueueAction"=DeviceQueue_Action."Wait", "Numeric 1"=0.5) -> (w1824:T9)
        n846 = Bundle By Name(cluster=w1824, "QueueAction"=DeviceQueue_Action."Spectrometer_SetFrames", "Numeric 1"=w1809) -> (w1807:T9)
        n847 = Enqueue Element(queue=w1820, element=w1825, error in (no error)=w1819) -> (queue out=w1818:refnum<queue>, error out=w1817:errorcluster)  [unwired: 1 in, 1 out]
        n848 = Bundle By Name(cluster=w1807, "QueueAction"=DeviceQueue_Action."Spectrometer_SetDarkspec") -> (w1805:T9)
        n849 = Enqueue Element(queue=w1818, element=w1824, error in (no error)=w1817) -> (queue out=w1815:refnum<queue>, error out=w1816:errorcluster)  [unwired: 1 in, 1 out]
        n850 = Enqueue Element(queue=w1815, element=w1807, error in (no error)=w1816) -> (queue out=w1813:refnum<queue>, error out=w1812:errorcluster)  [unwired: 1 in, 1 out]
        n851 = Bundle By Name(cluster=w1805, "QueueAction"=DeviceQueue_Action."Spectrometer_SetFrames", "Numeric 1"=w1803) -> (w1806:T9)
        n852 = Enqueue Element(queue=w1813, element=w1805, error in (no error)=w1812) -> (queue out=w1811:refnum<queue>, error out=w1810:errorcluster)  [unwired: 1 in, 1 out]
        n853 = Enqueue Element(queue=w1811, element=w1806, error in (no error)=w1810) -> (queue out=w1801:refnum<queue>, error out=w1802:errorcluster)  [unwired: 1 in, 1 out]
      }
      event "StartMeasurement_Button": Value Change {
        w1835 = T6 {"QueueAction"=enum."TimeOut", "Data"=[], "Data_Raw"=[], "Data_Dark"=[], "Data_Ref"=[], "Device Information"=[], "Numeric Control"=0.0, "Boolean"=FALSE, "Wavelength"=[], "Time"=[], "Time Stamp"=timestamp(0 s since 1904-01-01), "Numeric Control 2"=0.0, "TabControl"=enum."Measure"}  # DataQueue
        w1843 = T9 {"QueueAction"=enum."TimeOut", "Numeric 1"=0.0, "Numeric 2"=0.0, "Boolean 1"=FALSE, "Boolean 2"=FALSE, "Spin Program"=[], "Spin Prg v07"=[], "Time Stamp"=timestamp(0 s since 1904-01-01), "TabControl"=enum."Measure"}  # Device Queue
        n854 = event-data() -> ()  [unwired: 1 in, 6 out]
        n855 = property on="Measure_Preview" class="Bool (strict)"("Value"=FALSE ("Preview")) -> ()  [unwired: 2 in, 2 out]
        n856 = Get Date/Time In Seconds() -> (seconds since 1Jan1904=w1829:timestamp)
        n857 = Bundle By Name(cluster=w1843, "QueueAction"=DeviceQueue_Action."Measure_InSituAdvanced", "Time Stamp"=w1829) -> (w1842:T9)
        n858 = Enqueue Element(queue=w1841, element=w1842, error in (no error)=w1839) -> (queue out=w1840:refnum<queue>, error out=w1830:errorcluster)  [unwired: 1 in, 1 out]
        n859 = Bundle By Name(cluster=w1835, "QueueAction"=DataQueue_Action."Measure_InSituSpinCoating", "Time Stamp"=w1829) -> (w1836:T6)
        n860 = Enqueue Element(queue=w1833, element=w1836, error in (no error)=w1830) -> (queue out=w1832:refnum<queue>, error out=w1831:errorcluster)  [unwired: 1 in, 1 out]
      }
      event "StartSpin_Button": Value Change {
        w1855 = T9 {"QueueAction"=enum."TimeOut", "Numeric 1"=0.0, "Numeric 2"=0.0, "Boolean 1"=FALSE, "Boolean 2"=FALSE, "Spin Program"=[], "Spin Prg v07"=[], "Time Stamp"=timestamp(0 s since 1904-01-01), "TabControl"=enum."Measure"}  # Device Queue
        n861 = event-data() -> ()  [unwired: 1 in, 6 out]
        n862 = Bundle By Name(cluster=w1855, "QueueAction"=DeviceQueue_Action."Arduino_StartProgram") -> (w1846:T9)
        n863 = Bundle By Name(cluster=w1846, "QueueAction"=DeviceQueue_Action."Arduino_Shutter_Close") -> (w1844:T9)
        n864 = Enqueue Element(queue=w1854, element=w1846, error in (no error)=w1852) -> (queue out=w1849:refnum<queue>, error out=w1850:errorcluster)  [unwired: 1 in, 1 out]
        n865 = Enqueue Element(queue=w1849, element=w1844, error in (no error)=w1850) -> (queue out=w1848:refnum<queue>, error out=w1847:errorcluster)  [unwired: 1 in, 1 out]
      }
      event "ESC_Milliseconds": Value Change {
        w1864 = T9 {"QueueAction"=enum."TimeOut", "Numeric 1"=0.0, "Numeric 2"=0.0, "Boolean 1"=FALSE, "Boolean 2"=FALSE, "Spin Program"=[], "Spin Prg v07"=[], "Time Stamp"=timestamp(0 s since 1904-01-01), "TabControl"=enum."Measure"}  # Device Queue
        n866 = event-data() -> ()  [unwired: 1 in, 6 out]
        n867 = Bundle By Name(cluster=w1864, "QueueAction"=DeviceQueue_Action."Arduino_SetMillis", "Numeric 1"="ESC_Milliseconds") -> (w1860:T9)
        n868 = Enqueue Element(queue=w1863, element=w1860, error in (no error)=w1861) -> (queue out=w1859:refnum<queue>, error out=w1858:errorcluster)  [unwired: 1 in, 1 out]
      }
      event "ESC_Speed": Value Change {
        w1873 = T9 {"QueueAction"=enum."TimeOut", "Numeric 1"=0.0, "Numeric 2"=0.0, "Boolean 1"=FALSE, "Boolean 2"=FALSE, "Spin Program"=[], "Spin Prg v07"=[], "Time Stamp"=timestamp(0 s since 1904-01-01), "TabControl"=enum."Measure"}  # Device Queue
        n869 = event-data() -> ()  [unwired: 1 in, 6 out]
        n870 = Bundle By Name(cluster=w1873, "QueueAction"=DeviceQueue_Action."Arduino_SetSpeed", "Numeric 1"="ESC_Speed") -> (w1869:T9)
        n871 = Enqueue Element(queue=w1872, element=w1869, error in (no error)=w1870) -> (queue out=w1868:refnum<queue>, error out=w1867:errorcluster)  [unwired: 1 in, 1 out]
      }
      event "ESC DEBUG": Value Change {
        n872 = event-data() -> ()  [unwired: 1 in, 6 out]
        n873 = Select(t=u8 0, s="ESC DEBUG", f=u8 2) -> (s? t:f=w1874:u8)
        n874 = property on="ESC_Milliseconds" class="DigNum (strict)"("DisabledEnum"=w1874) -> ()  [unwired: 2 in, 2 out]
        n875 = property on="ESC_Speed" class="DigNum (strict)"("DisabledEnum"=w1874) -> ()  [unwired: 2 in, 2 out]
      }
      event "Measure_FramesSpectrometer", "SpectralStability_FramesSpectrometer": Value Change {
        w1888 = T9 {"QueueAction"=enum."TimeOut", "Numeric 1"=0.0, "Numeric 2"=0.0, "Boolean 1"=FALSE, "Boolean 2"=FALSE, "Spin Program"=[], "Spin Prg v07"=[], "Time Stamp"=timestamp(0 s since 1904-01-01), "TabControl"=enum."Measure"}  # Device Queue
        n876 = event-data() -> ("NewVal"=w1882:dbl)  [unwired: 1 in, 5 out]
        n877 = property on="Tab Control" class="TabCtl (strict)"() -> ("Value"=w1881:T1)  [unwired: 2 in, 2 out]
        n878 = Bundle By Name(cluster=w1888, "QueueAction"=DeviceQueue_Action."Spectrometer_SetFrames", "Numeric 1"=w1882, "TabControl"=w1881) -> (w1889:T9)
        n879 = Enqueue Element(queue=w1886, element=w1889) -> (queue out=w1883:refnum<queue>)  [unwired: 2 in, 2 out]
      }
      event "Measure_MeasureSpectrum", "SpectralStability_MeasureSpectrum": Value Change {
        w1901 = T6 {"QueueAction"=enum."TimeOut", "Data"=[], "Data_Raw"=[], "Data_Dark"=[], "Data_Ref"=[], "Device Information"=[], "Numeric Control"=0.0, "Boolean"=FALSE, "Wavelength"=[], "Time"=[], "Time Stamp"=timestamp(0 s since 1904-01-01), "Numeric Control 2"=0.0, "TabControl"=enum."Measure"}  # DataQueue
        n880 = event-data() -> ()  [unwired: 1 in, 6 out]
        n881 = property on="Tab Control" class="TabCtl (strict)"() -> ("Value"=w1893:T1)  [unwired: 2 in, 2 out]
        n882 = case shown="\"Measure\"" w1893 {
          tunnel: w1895 -> [w1913 w1916]
          tunnel: [w1913 w1915] -> w1894
          tunnel: [w1912 w1914] -> w1892
          frame Default {
            w1912 = T9 {"QueueAction"=enum."TimeOut", "Numeric 1"=0.0, "Numeric 2"=0.0, "Boolean 1"=FALSE, "Boolean 2"=FALSE, "Spin Program"=[], "Spin Prg v07"=[], "Time Stamp"=timestamp(0 s since 1904-01-01), "TabControl"=enum."Measure"}  # Device Queue
          }
          frame "Measure" {
            w1919 = T9 {"QueueAction"=enum."TimeOut", "Numeric 1"=0.0, "Numeric 2"=0.0, "Boolean 1"=FALSE, "Boolean 2"=FALSE, "Spin Program"=[], "Spin Prg v07"=[], "Time Stamp"=timestamp(0 s since 1904-01-01), "TabControl"=enum."Measure"}  # Device Queue
            (unwired) T9 {"QueueAction"=enum."TimeOut", "Numeric 1"=0.0, "Numeric 2"=0.0, "Boolean 1"=FALSE, "Boolean 2"=FALSE, "Spin Program"=[], "Spin Prg v07"=[], "Time Stamp"=timestamp(0 s since 1904-01-01), "TabControl"=enum."Measure"}  # Device Queue
            n883 = Bundle By Name(cluster=w1919, "QueueAction"=DeviceQueue_Action."Spectrometer_SetFrames", "Numeric 1"="Frames for Ref/Dark") -> (w1914:T9)
            n884 = Enqueue Element(queue=w1916, element=w1914) -> (queue out=w1915:refnum<queue>)  [unwired: 2 in, 2 out]
          }
        }
        n885 = Get Date/Time In Seconds() -> (seconds since 1Jan1904=w1896:timestamp)
        n886 = Bundle By Name(cluster=w1892, "QueueAction"=DeviceQueue_Action."Measure_Spectrum", "Time Stamp"=w1896, "TabControl"=w1893) -> (w1904:T9)
        n887 = Enqueue Element(queue=w1894, element=w1904) -> (queue out=w1891:refnum<queue>)  [unwired: 2 in, 2 out]
        n888 = case shown="Default" w1893 {
          tunnel: w1892 -> [_ w1910]
          tunnel: w1891 -> [w1905 w1909]
          tunnel: [w1905 w1908] -> w1890
          frame Default {
          }
          frame "Measure" {
            n889 = property on="Measure_FramesSpectrometer" class="DigNum (strict)"() -> ("Value"=w1907:dbl)  [unwired: 2 in, 2 out]
            n890 = Bundle By Name(cluster=w1910, "QueueAction"=DeviceQueue_Action."Spectrometer_SetFrames", "Numeric 1"=w1907) -> (w1906:T9)
            n891 = Enqueue Element(queue=w1909, element=w1906) -> (queue out=w1908:refnum<queue>)  [unwired: 2 in, 2 out]
          }
        }
        n892 = Bundle By Name(cluster=w1901, "QueueAction"=DataQueue_Action."Measure_Spectrum", "TabControl"=w1893) -> (w1898:T6)
        n893 = Enqueue Element(queue=w1899, element=w1898) -> (queue out=w1897:refnum<queue>)  [unwired: 2 in, 2 out]
      }
      event "SpectralStability_Record": Value Change {
        w1928 = T6 {"QueueAction"=enum."TimeOut", "Data"=[], "Data_Raw"=[], "Data_Dark"=[], "Data_Ref"=[], "Device Information"=[], "Numeric Control"=0.0, "Boolean"=FALSE, "Wavelength"=[], "Time"=[], "Time Stamp"=timestamp(0 s since 1904-01-01), "Numeric Control 2"=0.0, "TabControl"=enum."Measure"}  # DataQueue
        w1933 = T9 {"QueueAction"=enum."TimeOut", "Numeric 1"=0.0, "Numeric 2"=0.0, "Boolean 1"=FALSE, "Boolean 2"=FALSE, "Spin Program"=[], "Spin Prg v07"=[], "Time Stamp"=timestamp(0 s since 1904-01-01), "TabControl"=enum."Measure"}  # Device Queue
        n894 = event-data() -> ()  [unwired: 1 in, 6 out]
        n895 = property on="Duration/\nTimes" class="Bool (strict)"() -> ("Value"=w1921:bool)  [unwired: 2 in, 2 out]
        n896 = case shown="False" w1921 {
          tunnel: ["SpectralStability_\nMeasurementNumber" w1936] -> w1920
          frame False {
            # "Number"
          }
          frame True {
            # "Duration"
            n897 = property on="SpectralStability_\nPeriodicTime" class="DigNum (strict)"() -> ("Value"=w1938:dbl[unit])  [unwired: 2 in, 2 out]
            n898 = Divide(x="SpectralStability_Duration", y=w1938) -> (x/y=w1939:dbl)
            n899 = Round Toward +Infinity(x=w1939) -> (ceil(x): smallest int >= x=w1937:dbl)
            n900 = Increment(x=w1937) -> (x+1=w1936:dbl)
          }
        }
        n901 = Get Date/Time In Seconds() -> (seconds since 1Jan1904=w1922:timestamp)
        n902 = property on="Tab Control" class="TabCtl (strict)"() -> ("Value"=w1923:T1)  [unwired: 2 in, 2 out]
        n903 = Bundle By Name(cluster=w1933, "QueueAction"=DeviceQueue_Action."Measure_SpectralStability", "Time Stamp"=w1922, "TabControl"=w1923, "Numeric 1"=w1920) -> (w1934:T9)
        n904 = property on="SS_StepsLeft" class="DigNum (strict)"("Value"=w1920) -> ()  [unwired: 2 in, 2 out]
        n905 = Enqueue Element(queue=w1931, element=w1934) -> (queue out=w1929:refnum<queue>)  [unwired: 2 in, 2 out]
        n906 = Bundle By Name(cluster=w1928, "QueueAction"=DataQueue_Action."Measure_SpectralStability", "TabControl"=w1923, "Time Stamp"=w1922, "Numeric Control"=w1920) -> (w1925:T6)
        n907 = Enqueue Element(queue=w1926, element=w1925) -> (queue out=w1924:refnum<queue>)  [unwired: 2 in, 2 out]
      }
      event "Automatically \nadjust count": Value Change {
        n908 = event-data() -> ("NewVal"=w1947:bool)  [unwired: 1 in, 5 out]
        n909 = Select(t=u8 2, s=w1947, f=u8 0) -> (s? t:f=w1941:u8)
        n910 = property on="Spectra Count" class="DigNum (strict)"("DisabledEnum"=w1941) -> ()  [unwired: 2 in, 2 out]
      }
      event "Duration/Times": Value Change {
        n911 = event-data() -> ("NewVal"=w1953:bool)  [unwired: 1 in, 5 out]
        n912 = case shown="False" w1953 {
          tunnel: [FALSE TRUE] -> w1952
          tunnel: [TRUE FALSE] -> w1951
          frame False {
          }
          frame True {
          }
        }
        n913 = property on="SpectralStability_Duration" class="DigNum (strict)"("Visible"=w1952) -> ()  [unwired: 2 in, 2 out]
        n914 = property on="SpectralStability_\nMeasurementNumber" class="DigNum (strict)"("Visible"=w1951) -> ()  [unwired: 2 in, 2 out]
      }
      event "Tab Control": Value Change {
        w1958 = FALSE ("SpectralStability_Preview")
        n915 = event-data() -> ("NewVal"=w1961:T1)  [unwired: 1 in]
        n916 = case shown="\"Spectral Stability\"" w1961 {
          tunnel: w1963 -> [w1966 w1979 w1994]
          tunnel: [w1966 w1968 w1985] -> w1960
          tunnel: w1962 -> [w1965 w1978 w1993]
          tunnel: w1961 -> [_ w1977 w1992]
          tunnel: [w1965 w1967 w1984] -> w1959
          frame Default {
          }
          frame "Measure" {
            w1981 = T9 {"QueueAction"=enum."TimeOut", "Numeric 1"=0.0, "Numeric 2"=0.0, "Boolean 1"=FALSE, "Boolean 2"=FALSE, "Spin Program"=[], "Spin Prg v07"=[], "Time Stamp"=timestamp(0 s since 1904-01-01), "TabControl"=enum."Measure"}  # Device Queue
            n917 = property on="Measure_IntegrationTime" class="DigNum (strict)"() -> ("Value"=w1976:dbl[unit])  [unwired: 2 in, 2 out]
            n918 = node(w1976) -> (w1975:dbl)
            n919 = Bundle By Name(cluster=w1981, "QueueAction"=DeviceQueue_Action."Spectrometer_SetIntegrationTime", "Numeric 1"=w1975, "TabControl"=w1977) -> (w1972:T9)
            n920 = property on="Measure_FramesSpectrometer" class="DigNum (strict)"() -> ("Value"=w1970:dbl)  [unwired: 2 in, 2 out]
            n921 = Enqueue Element(queue=w1979, element=w1972, error in (no error)=w1978) -> (queue out=w1974:refnum<queue>, error out=w1973:errorcluster)  [unwired: 1 in, 1 out]
            n922 = Bundle By Name(cluster=w1972, "QueueAction"=DeviceQueue_Action."Spectrometer_SetFrames", "Numeric 1"=w1970) -> (w1969:T9)
            n923 = Enqueue Element(queue=w1974, element=w1969, error in (no error)=w1973) -> (queue out=w1968:refnum<queue>, error out=w1967:errorcluster)  [unwired: 1 in, 1 out]
          }
          frame "Spectral Stability" {
            w1996 = T9 {"QueueAction"=enum."TimeOut", "Numeric 1"=0.0, "Numeric 2"=0.0, "Boolean 1"=FALSE, "Boolean 2"=FALSE, "Spin Program"=[], "Spin Prg v07"=[], "Time Stamp"=timestamp(0 s since 1904-01-01), "TabControl"=enum."Measure"}  # Device Queue
            n924 = property on="SpectralStability_IntegrationTime" class="DigNum (strict)"() -> ("Value"=w1983:dbl[unit])  [unwired: 2 in, 2 out]
            n925 = node(w1983) -> (w1991:dbl)
            n926 = property on="SpectralStability_FramesSpectrometer" class="DigNum (strict)"() -> ("Value"=w1982:dbl)  [unwired: 2 in, 2 out]
            n927 = Bundle By Name(cluster=w1996, "QueueAction"=DeviceQueue_Action."Spectrometer_SetIntegrationTime", "Numeric 1"=w1991, "TabControl"=w1992) -> (w1988:T9)
            n928 = Enqueue Element(queue=w1994, element=w1988, error in (no error)=w1993) -> (queue out=w1990:refnum<queue>, error out=w1989:errorcluster)  [unwired: 1 in, 1 out]
            n929 = Bundle By Name(cluster=w1988, "QueueAction"=DeviceQueue_Action."Spectrometer_SetFrames", "Numeric 1"=w1982) -> (w1986:T9)
            n930 = Enqueue Element(queue=w1990, element=w1986, error in (no error)=w1989) -> (queue out=w1985:refnum<queue>, error out=w1984:errorcluster)  [unwired: 1 in, 1 out]
          }
        }
        n931 = property on="SpectralStability_Preview" class="Bool (strict)"("Value"=w1958) -> ()  [unwired: 2 in, 2 out]
        n932 = property on="Measure_Preview" class="Bool (strict)"("Value"=w1958) -> ()  [unwired: 2 in, 2 out]
      }
      event "Trim\nSpec", "Wl \nUp", "Wl \nLow": Value Change {
        w2006 = T6 {"QueueAction"=enum."TimeOut", "Data"=[], "Data_Raw"=[], "Data_Dark"=[], "Data_Ref"=[], "Device Information"=[], "Numeric Control"=0.0, "Boolean"=FALSE, "Wavelength"=[], "Time"=[], "Time Stamp"=timestamp(0 s since 1904-01-01), "Numeric Control 2"=0.0, "TabControl"=enum."Measure"}  # DataQueue
        n933 = event-data() -> ()  [unwired: 1 in, 6 out]
        n934 = node("Wl \nLow") -> (w2000:dbl)
        n935 = node("Wl \nUp") -> (w1999:dbl)
        n936 = Bundle By Name(cluster=w2006, "QueueAction"=DataQueue_Action."Change_TrimSettings", "Numeric Control"=w2000, "Numeric Control 2"=w1999, "Boolean"="Trim\nSpec") -> (w2007:T6)
        n937 = Enqueue Element(queue=w2005, element=w2007) -> (queue out=w2004:refnum<queue>)  [unwired: 2 in, 2 out]
      }
    }
  }
  n938 = disable-structure shown="Disabled" {
    frame Disabled {
      w2010 = T9 {"QueueAction"=enum."TimeOut", "Numeric 1"=0.0, "Numeric 2"=0.0, "Boolean 1"=FALSE, "Boolean 2"=FALSE, "Spin Program"=[], "Spin Prg v07"=[], "Time Stamp"=timestamp(0 s since 1904-01-01), "TabControl"=enum."Measure"}  # Device Queue
      w2012 = T9 {"QueueAction"=enum."TimeOut", "Numeric 1"=0.0, "Numeric 2"=0.0, "Boolean 1"=FALSE, "Boolean 2"=FALSE, "Spin Program"=[], "Spin Prg v07"=[], "Time Stamp"=timestamp(0 s since 1904-01-01), "TabControl"=enum."Measure"}  # Device Queue
      n939 = Bundle By Name(cluster=w2010, "QueueAction"=DeviceQueue_Action."Arduino_SetSpeed") -> (w2011:T9)  [unwired: 1 in]
      n940 = Bundle By Name(cluster=w2012) -> ()  [unwired: 2 in, 1 out]
      n941 = Enqueue Element(element=w2011) -> ()  [unwired: 3 in, 3 out]
    }
    frame Enabled {
    }
  }
  n942 = Release Queue(queue=w9) -> ()  [unwired: 2 in, 3 out]
  n943 = Release Queue(queue=w10) -> ()  [unwired: 2 in, 3 out]
